vi "VFD.vi"() -> ()   [LabVIEW 2013]
uses:
  <vilib>/NI/Modbus Library/API/Master/Modbus Master.lvclass
  Variables globales/Temporales.vi
  Variables globales/Permanentes.vi
panel:
  out "Coincidentes":bool[](array[boolean])
  out "Iteración":u32
  out "Estatus (color)":u32(colorbox)
  in  "Modos":enum32{"Parámetros", "Control", "Recetas"}(tab)
  in  "Escanear":bool
  in  "Download":bool
  in  "Contenedor Fabricantes":T1(tab)
  in  "Referencias PowerFlex":T2 {"Referencia velocidad 2" items=["Potenciómetro"=1, "Teclado"=2, "Modbus"=3, "Analógica (0-10V)"=5, "Analógica (4-20mA)"=6]; "Referencia arranque 2" items=["Teclado"=1, "Terminales"=2, "Modbus"=3]; "Referencia velocidad 1" items=["Potenciómetro"=1, "Teclado"=2, "Modbus"=3, "Analógica (0-10V)"=5, "Analógica (4-20mA)"=6]; "Referencia arranque 1" items=["Teclado"=1, "Terminales"=2, "Modbus"=3]}
  in  "I/O PowerFlex":T3 {"Relevador" items=["Listo/Fallo"=0, "A frecuencia"=1, "Alimentación"=2, "Sobrefrecuencia"=6, "Sobrecorriente"=7, "Sobretensión"=8, "Modbus"=13]; "Entrada 6 (06)" items=["No asignar"=0, "Referencia vel. 2"=1, "Referencia vel. 3"=2, "Fallo auxiliar"=12, "Reset"=13, "Entrada lógica 1"=24, "Entrada lógica 2"=25]; "Entrada 5 (05)" items=["No asignar"=0, "Referencia vel. 2"=1, "Referencia vel. 3"=2, "Fallo auxiliar"=12, "Reset"=13, "Entrada lógica 1"=24, "Entrada lógica 2"=25]; "Entrada 3 (03)" items=["No asignar"=0, "Referencia vel. 2"=1, "Referencia vel. 3"=2, "Fallo auxiliar"=12, "Reset"=13, "Entrada lógica 1"=24, "Entrada lógica 2"=25, "REV 2 hilos"=50, "DIR 3 hilos"=51]; "Entrada 2 (02)" items=["No asignar"=0, "Referencia vel. 2"=1, "Referencia vel. 3"=2, "Fallo auxiliar"=12, "Reset"=13, "Entrada lógica 1"=24, "Entrada lógica 2"=25, "FWD 2 hilos"=48, "RUN 3 hilos"=49]}
  in  "Motor PowerFlex":T4={"Voltaje nominal"=0, "Frecuencia nominal"=0, "Corriente sobrecarga"=0.0, "Corriente nominal"=0.0, "Polos"=2, "Velocidad nominal"=0, "T. Aceleración"=0.0, "T. Desaleceración"=0.0, "Descargar"=FALSE} {"T. Desaleceración" format="%#_g seg"; "T. Aceleración" format="%#_g seg"; "Velocidad nominal" format="%.0f rpm"; "Voltaje nominal" format="%.0f V"; "Frecuencia nominal" format="%.0f Hz"; "Corriente sobrecarga" format="%#_g Amp"; "Corriente nominal" format="%#_g Amp"; "Polos" min=2 max=40}
  in  "Modbus PowerFlex":T5={"Velocidad datos"=0, "Identificador"=1, "Acc. pérdida comun."=0, "Tmp. pérdida comun."=1.0, "Formato RS485"=0, "Descargar"=FALSE} {"Tmp. pérdida comun." min=0.0 max=60.0 format="%#_g seg."; "Identificador" min=1 max=247; "Formato RS485" items=["RTU 8-N-1", "RTU 8-E-1", "RTU 8-O-1", "RTU 8-N-2", "RTU 8-E-2", "RTU 8-O-2"]; "Acc. pérdida comun." items=["Fallo", "Paro inercia", "Paro", "Nada"]; "Velocidad datos" items=["9600 bps", "2400 bps", "4800 bps", "9600 bps", "19200 bps", "38400 bps"]}
  in  "Referencias Schneider":T2 {"Referencia velocidad 2" items=["No asignar"=0, "Analógica (AI1)"=1, "Analógica (AI2)"=2, "Analógica (AI3)"=3, "Modbus"=164, "Potenciómetro (AIU1)"=183]; "Referencia arranque 2" items=["Terminales"=1, "Modbus"=10]; "Referencia velocidad 1" items=["No asignar"=0, "Analógica (AI1)"=1, "Analógica (AI2)"=2, "Analógica (AI3)"=3, "Modbus"=164, "Potenciómetro (AIU1)"=183]; "Referencia arranque 1" items=["Terminales"=1, "Modbus"=10]}
  in  "I/O Schneider":T6 {"Transistor" items=["Listo/Fallo"=0, "A frecuencia"=1, "Alimentación"=2, "Sobrefrecuencia"=6, "Sobrecorriente"=7, "Sobretensión"=8, "Modbus"=13]; "Relevador 2 (R2)" items=["Listo/Fallo"=0, "A frecuencia"=1, "Alimentación"=2, "Sobrefrecuencia"=6, "Sobrecorriente"=7, "Sobretensión"=8, "Modbus"=13]; "Relevador 1 (R1)" items=["Listo/Fallo"=0, "A frecuencia"=1, "Alimentación"=2, "Sobrefrecuencia"=6, "Sobrecorriente"=7, "Sobretensión"=8, "Modbus"=13]; "Entrada 6 (DI6)" items=["Listo/Fallo"=0, "A frecuencia"=1, "Alimentación"=2, "Sobrefrecuencia"=6, "Sobrecorriente"=7, "Sobretensión"=8, "Modbus"=13]; "Entrada 5 (DI5)" items=["Listo/Fallo"=0, "A frecuencia"=1, "Alimentación"=2, "Sobrefrecuencia"=6, "Sobrecorriente"=7, "Sobretensión"=8, "Modbus"=13]; "Entrada 4 (DI4)" items=["Sin asignar"=0, "Referencia vel. 2"=1, "Referencia vel. 3"=2, "Fallo auxiliar"=12, "Reset"=13, "Entrada lógica 1"=24, "Entrada lógica 2"=25]; "Entrada 3 (DI3)" items=["No asignar"=0, "Referencia vel. 2"=1, "Referencia vel. 3"=2, "Fallo auxiliar"=12, "Reset"=13, "Entrada lógica 1"=24, "Entrada lógica 2"=25]; "Entrada 2 (DI2)" items=["No asignar"=0, "Referencia vel. 2"=1, "Referencia vel. 3"=2, "Fallo auxiliar"=12, "Reset"=13, "Entrada lógica 1"=24, "Entrada lógica 2"=25, "REV 2 hilos"=50, "DIR 3 hilos"=51]; "Entrada 1 (DI1)" items=["No asignar"=0, "Referencia vel. 2"=1, "Referencia vel. 3"=2, "Fallo auxiliar"=12, "Reset"=13, "Entrada lógica 1"=24, "Entrada lógica 2"=25, "FWD 2 hilos"=48, "RUN 3 hilos"=49]}
  in  "Referencias Delta":T2 {"Referencia velocidad 2" items=["Potenciómetro"=1, "Teclado"=2, "Modbus"=3, "Analógico (0-10V)"=5, "Analógico (4-20mA)"=6]; "Referencia arranque 2" items=["Teclado"=1, "Terminales"=2, "Modbus"=3]; "Referencia velocidad 1" items=["Potenciómetro"=1, "Teclado"=2, "Modbus"=3, "Analógico (0-10V)"=5, "Analógico (4-20mA)"=6]; "Referencia arranque 1" items=["Teclado"=1, "Terminales"=2, "Modbus"=3]}
  in  "I/O Delta":T7 {"Entrada 6 (MI6)" items=["Listo/Fallo"=0, "A frecuencia"=1, "Alimentación"=2, "Sobrefrecuencia"=6, "Sobrecorriente"=7, "Sobretensión"=8, "Modbus"=13]; "Entrada 5 (MI5)" items=["Listo/Fallo"=0, "A frecuencia"=1, "Alimentación"=2, "Sobrefrecuencia"=6, "Sobrecorriente"=7, "Sobretensión"=8, "Modbus"=13]; "Entrada 4 (MI4)" items=["Sin asignar"=0, "Referencia vel. 2"=1, "Referencia vel. 3"=2, "Fallo auxiliar"=12, "Reset"=13, "Entrada lógica 1"=24, "Entrada lógica 2"=25]; "Entrada 3 (MI3)" items=["No asignar"=0, "Referencia vel. 2"=1, "Referencia vel. 3"=2, "Fallo auxiliar"=12, "Reset"=13, "Entrada lógica 1"=24, "Entrada lógica 2"=25]; "Entrada 2 (MI2)" items=["No asignar"=0, "Referencia vel. 2"=1, "Referencia vel. 3"=2, "Fallo auxiliar"=12, "Reset"=13, "Entrada lógica 1"=24, "Entrada lógica 2"=25, "REV 2 hilos"=50, "DIR 3 hilos"=51]; "Entrada 1 (MI1)" items=["No asignar"=0, "Referencia vel. 2"=1, "Referencia vel. 3"=2, "Fallo auxiliar"=12, "Reset"=13, "Entrada lógica 1"=24, "Entrada lógica 2"=25, "FWD 2 hilos"=48, "RUN 3 hilos"=49]}
  in  "Referencias ABB":T2 {"Referencia velocidad 2" items=["Potenciómetro"=1, "Teclado"=2, "Modbus"=3, "Analógico (0-10V)"=5, "Analógico (4-20mA)"=6]; "Referencia arranque 2" items=["Teclado"=1, "Terminales"=2, "Modbus"=3]; "Referencia velocidad 1" items=["Potenciómetro"=1, "Teclado"=2, "Modbus"=3, "Analógico (0-10V)"=5, "Analógico (4-20mA)"=6]; "Referencia arranque 1" items=["Teclado"=1, "Terminales"=2, "Modbus"=3]}
  in  "I/O ABB":T8 {"Entrada 4 (DI4)" items=["Sin asignar"=0, "Referencia vel. 2"=1, "Referencia vel. 3"=2, "Fallo auxiliar"=12, "Reset"=13, "Entrada lógica 1"=24, "Entrada lógica 2"=25]; "Entrada 3 (DI3)" items=["No asignar"=0, "Referencia vel. 2"=1, "Referencia vel. 3"=2, "Fallo auxiliar"=12, "Reset"=13, "Entrada lógica 1"=24, "Entrada lógica 2"=25]; "Entrada 2 (DI2)" items=["No asignar"=0, "Referencia vel. 2"=1, "Referencia vel. 3"=2, "Fallo auxiliar"=12, "Reset"=13, "Entrada lógica 1"=24, "Entrada lógica 2"=25, "REV 2 hilos"=50, "DIR 3 hilos"=51]; "Entrada 1 (DI1)" items=["No asignar"=0, "Referencia vel. 2"=1, "Referencia vel. 3"=2, "Fallo auxiliar"=12, "Reset"=13, "Entrada lógica 1"=24, "Entrada lógica 2"=25, "FWD 2 hilos"=48, "RUN 3 hilos"=49]}
  in  "Referencias LS-Electric":T2 {"Referencia velocidad 2" items=["Teclado"=0, "Analógica (V1)"=2, "Analógica (I2)"=5, "Modbus"=6]; "Referencia arranque 2" items=["Teclado"=0, "Terminales"=1, "Modbus"=3]; "Referencia velocidad 1" items=["Teclado"=0, "Analógica (V1)"=2, "Analógica (I2)"=5, "Modbus"=6]; "Referencia arranque 1" items=["Teclado"=0, "Terminales"=1, "Modbus"=3]}
  in  "I/O LS-Electric":T9 {"Relevador 2" items=["Modbus"=0, "FDT-1"=1, "FDT-2"=2, "FDT-3"=3, "FDT-4"=4, "Sobrecarga"=5, "Sobrevoltaje"=10, "Bajo voltaje"=11, "Sobrecalentamiento"=12, "RUN"=14, "STOP"=15, "Listo"=22]; "Relevador 1" items=["Modbus"=0, "FDT-1"=1, "FDT-2"=2, "FDT-3"=3, "FDT-4"=4, "Sobrecarga"=5, "Sobrevoltaje"=10, "Bajo voltaje"=11, "Sobrecalentamiento"=12, "RUN"=14, "STOP"=15, "Listo"=22]; "Entrada 5 (P5)" items=["No asignar"=0, "FWD"=1, "REV"=2, "Reset"=3, "Fallo auxiliar (BX)"=5, "Habilitar RUN"=13, "3 hilos"=14, "Segunda referencia"=15, "Segundo motor"=26]; "Entrada 4 (P4)" items=["Sin asignar"=0, "FWD"=1, "REV"=2, "Reset"=3, "Fallo auxiliar (BX)"=5, "Habilitar RUN"=13, "3 hilos"=14, "Segunda referencia"=15, "Segundo motor"=26]; "Entrada 3 (P3)" items=["No asignar"=0, "FWD"=1, "REV"=2, "Reset"=3, "Fallo auxiliar (BX)"=5, "Habilitar RUN"=13, "3 hilos"=14, "Segunda referencia"=15, "Segundo motor"=26]; "Entrada 2 (P2)" items=["No asignar"=0, "FWD"=1, "REV"=2, "Reset"=3, "Fallo auxiliar (BX)"=5, "Habilitar RUN"=13, "3 hilos"=14, "Segunda referencia"=15, "Segundo motor"=26]; "Entrada 1 (P1)" items=["No asignar"=0, "FWD"=1, "REV"=2, "Reset"=3, "Fallo auxiliar (BX)"=5, "Habilitar RUN"=13, "3 hilos"=14, "Segunda referencia"=15, "Segundo motor"=26]}
  in  "Motor LS-Electric":T10={"Frecuencia nominal"=0, "Polos"=2, "Velocidad nominal"=0, "Corriente nominal"=0.0, "Corriente sin carga"=0.0, "Voltaje nominal"=170, "Potencia nominal"=0, "Frecuencia mínima"=0.0, "Frecuencia máxima"=0.0, "T. Aceleración"=0.0, "T. Desaceleración"=0.0, "Descargar"=FALSE} {"Voltaje nominal" min=170 max=480 format="%.0f V"; "Potencia nominal" items=["0.2 kW", "0.4 kW", "0.75 kW", "1.1 kW", "1.5 kW", "2.2 kW", "3.0 kW", "3.7 kW", "4.0 kW", "5.5 kW", "7.5 kW", "11.kW"]; "T. Desaceleración" format="%#_g seg"; "T. Aceleración" format="%#_g seg"; "Frecuencia máxima" format="%#_g Hz"; "Frecuencia mínima" format="%#_g Hz"; "Polos" min=2 max=48; "Velocidad nominal" format="%.0f rpm"; "Corriente nominal" format="%#_g Amp"; "Corriente sin carga" format="%#_g Amp"; "Frecuencia nominal" items=["60 Hz", "50 Hz"]}
  in  "Modbus LS-Electric":T11={"Identificador"=1, "Velocidad datos"=0, "Formato RS485"=0, "Delay respuesta"=1, "Descargar"=FALSE} {"Delay respuesta" min=1 max=250 format="%.0f mseg."; "Formato RS485" items=["RTU 8-N-1", "RTU 8-N-2", "RTU 8-E-1", "RTU 8-O-1"]; "Velocidad datos" items=["1200 bps", "2400 bps", "4800 bps", "9600 bps", "19200 bps", "38400 bps", "56 kbps", "115 kbps"]; "Identificador" min=1 max=250}
  in  "Programa":T12 {"Programa" items=["ab1", "ab2", "ab3", "ab4"]}
  in  "Run":bool
  in  "Sentido":bool
  in  "Reset":bool
  in  "Salidas digitales":cluster{"Salida":bool, "Etiqueta":string}[](array[cluster])
  out "Entradas digitales":cluster{"Estado":bool, "Etiqueta":string}[](array[cluster])
  in  "Frecuencia":dbl format="%#_g Hz."
  in  "Recetas":T13(tab)
  in  "Recetas Allen Bradley":T14(array[cluster]) {"Modbus PowerFlex"."Tmp. pérdida comun." min=0.0 max=60.0 format="%#_g seg."; "Modbus PowerFlex"."Identificador" min=1 max=247; "Modbus PowerFlex"."Formato RS485" items=["RTU 8-N-1", "RTU 8-E-1", "RTU 8-O-1", "RTU 8-N-2", "RTU 8-E-2", "RTU 8-O-2"]; "Modbus PowerFlex"."Acc. pérdida comun." items=["Fallo", "Paro inercia", "Paro", "Nada"]; "Modbus PowerFlex"."Velocidad datos" items=["9600 bps", "2400 bps", "4800 bps", "9600 bps", "19200 bps", "38400 bps"]; "Motor PowerFlex"."T. Desaleceración" format="%#_g seg"; "Motor PowerFlex"."T. Aceleración" format="%#_g seg"; "Motor PowerFlex"."Velocidad nominal" format="%.0f rpm"; "Motor PowerFlex"."Voltaje nominal" format="%.0f V"; "Motor PowerFlex"."Frecuencia nominal" format="%.0f Hz"; "Motor PowerFlex"."Corriente sobrecarga" format="%#_g Amp"; "Motor PowerFlex"."Corriente nominal" format="%#_g Amp"; "Motor PowerFlex"."Polos" min=2 max=40; "I/O PowerFlex"."Relevador" items=["Listo/Fallo"=0, "A frecuencia"=1, "Alimentación"=2, "Sobrefrecuencia"=6, "Sobrecorriente"=7, "Sobretensión"=8, "Modbus"=13]; "I/O PowerFlex"."Entrada 6 (06)" items=["No asignar"=0, "Referencia vel. 2"=1, "Referencia vel. 3"=2, "Fallo auxiliar"=12, "Reset"=13, "Entrada lógica 1"=24, "Entrada lógica 2"=25]; "I/O PowerFlex"."Entrada 5 (05)" items=["No asignar"=0, "Referencia vel. 2"=1, "Referencia vel. 3"=2, "Fallo auxiliar"=12, "Reset"=13, "Entrada lógica 1"=24, "Entrada lógica 2"=25]; "I/O PowerFlex"."Entrada 3 (03)" items=["No asignar"=0, "Referencia vel. 2"=1, "Referencia vel. 3"=2, "Fallo auxiliar"=12, "Reset"=13, "Entrada lógica 1"=24, "Entrada lógica 2"=25, "REV 2 hilos"=50, "DIR 3 hilos"=51]; "I/O PowerFlex"."Entrada 2 (02)" items=["No asignar"=0, "Referencia vel. 2"=1, "Referencia vel. 3"=2, "Fallo auxiliar"=12, "Reset"=13, "Entrada lógica 1"=24, "Entrada lógica 2"=25, "FWD 2 hilos"=48, "RUN 3 hilos"=49]; "Referencias PowerFlex"."Referencia velocidad 2" items=["Potenciómetro"=1, "Teclado"=2, "Modbus"=3, "Analógica (0-10V)"=5, "Analógica (4-20mA)"=6]; "Referencias PowerFlex"."Referencia arranque 2" items=["Teclado"=1, "Terminales"=2, "Modbus"=3]; "Referencias PowerFlex"."Referencia velocidad 1" items=["Potenciómetro"=1, "Teclado"=2, "Modbus"=3, "Analógica (0-10V)"=5, "Analógica (4-20mA)"=6]; "Referencias PowerFlex"."Referencia arranque 1" items=["Teclado"=1, "Terminales"=2, "Modbus"=3]}
  in  "Recetas Schneider":T15(array[cluster]) {"I/O Schneider"."Transistor" items=["Listo/Fallo"=0, "A frecuencia"=1, "Alimentación"=2, "Sobrefrecuencia"=6, "Sobrecorriente"=7, "Sobretensión"=8, "Modbus"=13]; "I/O Schneider"."Relevador 2 (R2)" items=["Listo/Fallo"=0, "A frecuencia"=1, "Alimentación"=2, "Sobrefrecuencia"=6, "Sobrecorriente"=7, "Sobretensión"=8, "Modbus"=13]; "I/O Schneider"."Relevador 1 (R1)" items=["Listo/Fallo"=0, "A frecuencia"=1, "Alimentación"=2, "Sobrefrecuencia"=6, "Sobrecorriente"=7, "Sobretensión"=8, "Modbus"=13]; "I/O Schneider"."Entrada 6 (DI6)" items=["Listo/Fallo"=0, "A frecuencia"=1, "Alimentación"=2, "Sobrefrecuencia"=6, "Sobrecorriente"=7, "Sobretensión"=8, "Modbus"=13]; "I/O Schneider"."Entrada 5 (DI5)" items=["Listo/Fallo"=0, "A frecuencia"=1, "Alimentación"=2, "Sobrefrecuencia"=6, "Sobrecorriente"=7, "Sobretensión"=8, "Modbus"=13]; "I/O Schneider"."Entrada 4 (DI4)" items=["Sin asignar"=0, "Referencia vel. 2"=1, "Referencia vel. 3"=2, "Fallo auxiliar"=12, "Reset"=13, "Entrada lógica 1"=24, "Entrada lógica 2"=25]; "I/O Schneider"."Entrada 3 (DI3)" items=["No asignar"=0, "Referencia vel. 2"=1, "Referencia vel. 3"=2, "Fallo auxiliar"=12, "Reset"=13, "Entrada lógica 1"=24, "Entrada lógica 2"=25]; "I/O Schneider"."Entrada 2 (DI2)" items=["No asignar"=0, "Referencia vel. 2"=1, "Referencia vel. 3"=2, "Fallo auxiliar"=12, "Reset"=13, "Entrada lógica 1"=24, "Entrada lógica 2"=25, "REV 2 hilos"=50, "DIR 3 hilos"=51]; "I/O Schneider"."Entrada 1 (DI1)" items=["No asignar"=0, "Referencia vel. 2"=1, "Referencia vel. 3"=2, "Fallo auxiliar"=12, "Reset"=13, "Entrada lógica 1"=24, "Entrada lógica 2"=25, "FWD 2 hilos"=48, "RUN 3 hilos"=49]; "Referencias Schneider"."Referencia velocidad 2" items=["No asignar"=0, "Analógica (AI1)"=1, "Analógica (AI2)"=2, "Analógica (AI3)"=3, "Modbus"=164, "Potenciómetro (AIU1)"=183]; "Referencias Schneider"."Referencia arranque 2" items=["Terminales"=1, "Modbus"=10]; "Referencias Schneider"."Referencia velocidad 1" items=["No asignar"=0, "Analógica (AI1)"=1, "Analógica (AI2)"=2, "Analógica (AI3)"=3, "Modbus"=164, "Potenciómetro (AIU1)"=183]; "Referencias Schneider"."Referencia arranque 1" items=["Terminales"=1, "Modbus"=10]}
  in  "Recetas Delta":T16(array[cluster]) {"Referencias Delta"."Referencia velocidad 2" items=["No asignar"=0, "Analógica (AI1)"=1, "Analógica (AI2)"=2, "Analógica (AI3)"=3, "Modbus"=164, "Potenciómetro (AIU1)"=183]; "Referencias Delta"."Referencia arranque 2" items=["Terminales"=1, "Modbus"=10]; "Referencias Delta"."Referencia velocidad 1" items=["No asignar"=0, "Analógica (AI1)"=1, "Analógica (AI2)"=2, "Analógica (AI3)"=3, "Modbus"=164, "Potenciómetro (AIU1)"=183]; "Referencias Delta"."Referencia arranque 1" items=["Terminales"=1, "Modbus"=10]; "I/O Delta"."Entrada 6 (MI6)" items=["Listo/Fallo"=0, "A frecuencia"=1, "Alimentación"=2, "Sobrefrecuencia"=6, "Sobrecorriente"=7, "Sobretensión"=8, "Modbus"=13]; "I/O Delta"."Entrada 5 (MI5)" items=["Listo/Fallo"=0, "A frecuencia"=1, "Alimentación"=2, "Sobrefrecuencia"=6, "Sobrecorriente"=7, "Sobretensión"=8, "Modbus"=13]; "I/O Delta"."Entrada 4 (MI4)" items=["Sin asignar"=0, "Referencia vel. 2"=1, "Referencia vel. 3"=2, "Fallo auxiliar"=12, "Reset"=13, "Entrada lógica 1"=24, "Entrada lógica 2"=25]; "I/O Delta"."Entrada 3 (MI3)" items=["No asignar"=0, "Referencia vel. 2"=1, "Referencia vel. 3"=2, "Fallo auxiliar"=12, "Reset"=13, "Entrada lógica 1"=24, "Entrada lógica 2"=25]; "I/O Delta"."Entrada 2 (MI2)" items=["No asignar"=0, "Referencia vel. 2"=1, "Referencia vel. 3"=2, "Fallo auxiliar"=12, "Reset"=13, "Entrada lógica 1"=24, "Entrada lógica 2"=25, "REV 2 hilos"=50, "DIR 3 hilos"=51]; "I/O Delta"."Entrada 1 (MI1)" items=["No asignar"=0, "Referencia vel. 2"=1, "Referencia vel. 3"=2, "Fallo auxiliar"=12, "Reset"=13, "Entrada lógica 1"=24, "Entrada lógica 2"=25, "FWD 2 hilos"=48, "RUN 3 hilos"=49]}
  in  "Recetas ABB":T17(array[cluster]) {"Referencias ABB"."Referencia velocidad 2" items=["No asignar"=0, "Analógica (AI1)"=1, "Analógica (AI2)"=2, "Analógica (AI3)"=3, "Modbus"=164, "Potenciómetro (AIU1)"=183]; "Referencias ABB"."Referencia arranque 2" items=["Terminales"=1, "Modbus"=10]; "Referencias ABB"."Referencia velocidad 1" items=["No asignar"=0, "Analógica (AI1)"=1, "Analógica (AI2)"=2, "Analógica (AI3)"=3, "Modbus"=164, "Potenciómetro (AIU1)"=183]; "Referencias ABB"."Referencia arranque 1" items=["Terminales"=1, "Modbus"=10]; "I/O ABB"."Entrada 4 (DI4)" items=["Sin asignar"=0, "Referencia vel. 2"=1, "Referencia vel. 3"=2, "Fallo auxiliar"=12, "Reset"=13, "Entrada lógica 1"=24, "Entrada lógica 2"=25]; "I/O ABB"."Entrada 3 (DI3)" items=["No asignar"=0, "Referencia vel. 2"=1, "Referencia vel. 3"=2, "Fallo auxiliar"=12, "Reset"=13, "Entrada lógica 1"=24, "Entrada lógica 2"=25]; "I/O ABB"."Entrada 2 (DI2)" items=["No asignar"=0, "Referencia vel. 2"=1, "Referencia vel. 3"=2, "Fallo auxiliar"=12, "Reset"=13, "Entrada lógica 1"=24, "Entrada lógica 2"=25, "REV 2 hilos"=50, "DIR 3 hilos"=51]; "I/O ABB"."Entrada 1 (DI1)" items=["No asignar"=0, "Referencia vel. 2"=1, "Referencia vel. 3"=2, "Fallo auxiliar"=12, "Reset"=13, "Entrada lógica 1"=24, "Entrada lógica 2"=25, "FWD 2 hilos"=48, "RUN 3 hilos"=49]}
  in  "Recetas LS Electric":T18(array[cluster]) {"Modbus LS-Electric"."Delay respuesta" min=1 max=250 format="%.0f mseg."; "Modbus LS-Electric"."Formato RS485" items=["RTU 8-N-1", "RTU 8-N-2", "RTU 8-E-1", "RTU 8-O-1"]; "Modbus LS-Electric"."Velocidad datos" items=["1200 bps", "2400 bps", "4800 bps", "9600 bps", "19200 bps", "38400 bps", "56 kbps", "115 kbps"]; "Modbus LS-Electric"."Identificador" min=1 max=250; "Motor LS-Electric"."Voltaje nominal" min=170 max=480 format="%.0f V"; "Motor LS-Electric"."Potencia nominal" items=["0.2 kW", "0.4 kW", "0.75 kW", "1.1 kW", "1.5 kW", "2.2 kW", "3.0 kW", "3.7 kW", "4.0 kW", "5.5 kW", "7.5 kW", "11.kW"]; "Motor LS-Electric"."T. Desaceleración" format="%#_g seg"; "Motor LS-Electric"."T. Aceleración" format="%#_g seg"; "Motor LS-Electric"."Frecuencia máxima" format="%#_g Hz"; "Motor LS-Electric"."Frecuencia mínima" format="%#_g Hz"; "Motor LS-Electric"."Polos" min=2 max=48; "Motor LS-Electric"."Velocidad nominal" format="%.0f rpm"; "Motor LS-Electric"."Corriente nominal" format="%#_g Amp"; "Motor LS-Electric"."Corriente sin carga" format="%#_g Amp"; "Motor LS-Electric"."Frecuencia nominal" items=["60 Hz", "50 Hz"]; "Referencias LS-Electric"."Referencia velocidad 2" items=["No asignar"=0, "Analógica (AI1)"=1, "Analógica (AI2)"=2, "Analógica (AI3)"=3, "Modbus"=164, "Potenciómetro (AIU1)"=183]; "Referencias LS-Electric"."Referencia arranque 2" items=["Terminales"=1, "Modbus"=10]; "Referencias LS-Electric"."Referencia velocidad 1" items=["No asignar"=0, "Analógica (AI1)"=1, "Analógica (AI2)"=2, "Analógica (AI3)"=3, "Modbus"=164, "Potenciómetro (AIU1)"=183]; "Referencias LS-Electric"."Referencia arranque 1" items=["Terminales"=1, "Modbus"=10]; "I/O LS-Electric"."Relevador 2" items=["Modbus"=0, "FDT-1"=1, "FDT-2"=2, "FDT-3"=3, "FDT-4"=4, "Sobrecarga"=5, "Sobrevoltaje"=10, "Bajo voltaje"=11, "Sobrecalentamiento"=12, "RUN"=14, "STOP"=15, "Listo"=22]; "I/O LS-Electric"."Relevador 1" items=["Modbus"=0, "FDT-1"=1, "FDT-2"=2, "FDT-3"=3, "FDT-4"=4, "Sobrecarga"=5, "Sobrevoltaje"=10, "Bajo voltaje"=11, "Sobrecalentamiento"=12, "RUN"=14, "STOP"=15, "Listo"=22]; "I/O LS-Electric"."Entrada 5 (P5)" items=["No asignar"=0, "FWD"=1, "REV"=2, "Reset"=3, "Fallo auxiliar (BX)"=5, "Habilitar RUN"=13, "3 hilos"=14, "Segunda referencia"=15, "Segundo motor"=26]; "I/O LS-Electric"."Entrada 4 (P4)" items=["Sin asignar"=0, "FWD"=1, "REV"=2, "Reset"=3, "Fallo auxiliar (BX)"=5, "Habilitar RUN"=13, "3 hilos"=14, "Segunda referencia"=15, "Segundo motor"=26]; "I/O LS-Electric"."Entrada 3 (P3)" items=["No asignar"=0, "FWD"=1, "REV"=2, "Reset"=3, "Fallo auxiliar (BX)"=5, "Habilitar RUN"=13, "3 hilos"=14, "Segunda referencia"=15, "Segundo motor"=26]; "I/O LS-Electric"."Entrada 2 (P2)" items=["No asignar"=0, "FWD"=1, "REV"=2, "Reset"=3, "Fallo auxiliar (BX)"=5, "Habilitar RUN"=13, "3 hilos"=14, "Segunda referencia"=15, "Segundo motor"=26]; "I/O LS-Electric"."Entrada 1 (P1)" items=["No asignar"=0, "FWD"=1, "REV"=2, "Reset"=3, "Fallo auxiliar (BX)"=5, "Habilitar RUN"=13, "3 hilos"=14, "Segunda referencia"=15, "Segundo motor"=26]}
  out "Color Box 2":u32(colorbox)
  in  "cccc 2":u32
  out "cccc":u32
  in  "Color Box":u32(colorbox)
  out "Avance (número)":dbl format="%d%"
  out "Avance (anillo)":dbl(knob)=1.2869315802184793e-48 scale=0.0..101.0
  out "Mensaje":string
  in  "Stop":bool
  out "Salir":bool
  out "Instancia Modbus":refnum<class "Modbus Master.lvclass">
  out "Error Modbus":errorcluster
  in  "Timeout":u32
  in  "Fabricante":u32(ring)
  out "Paso":u32
  in  "Puerto COM":refnum<visa-resource-name>
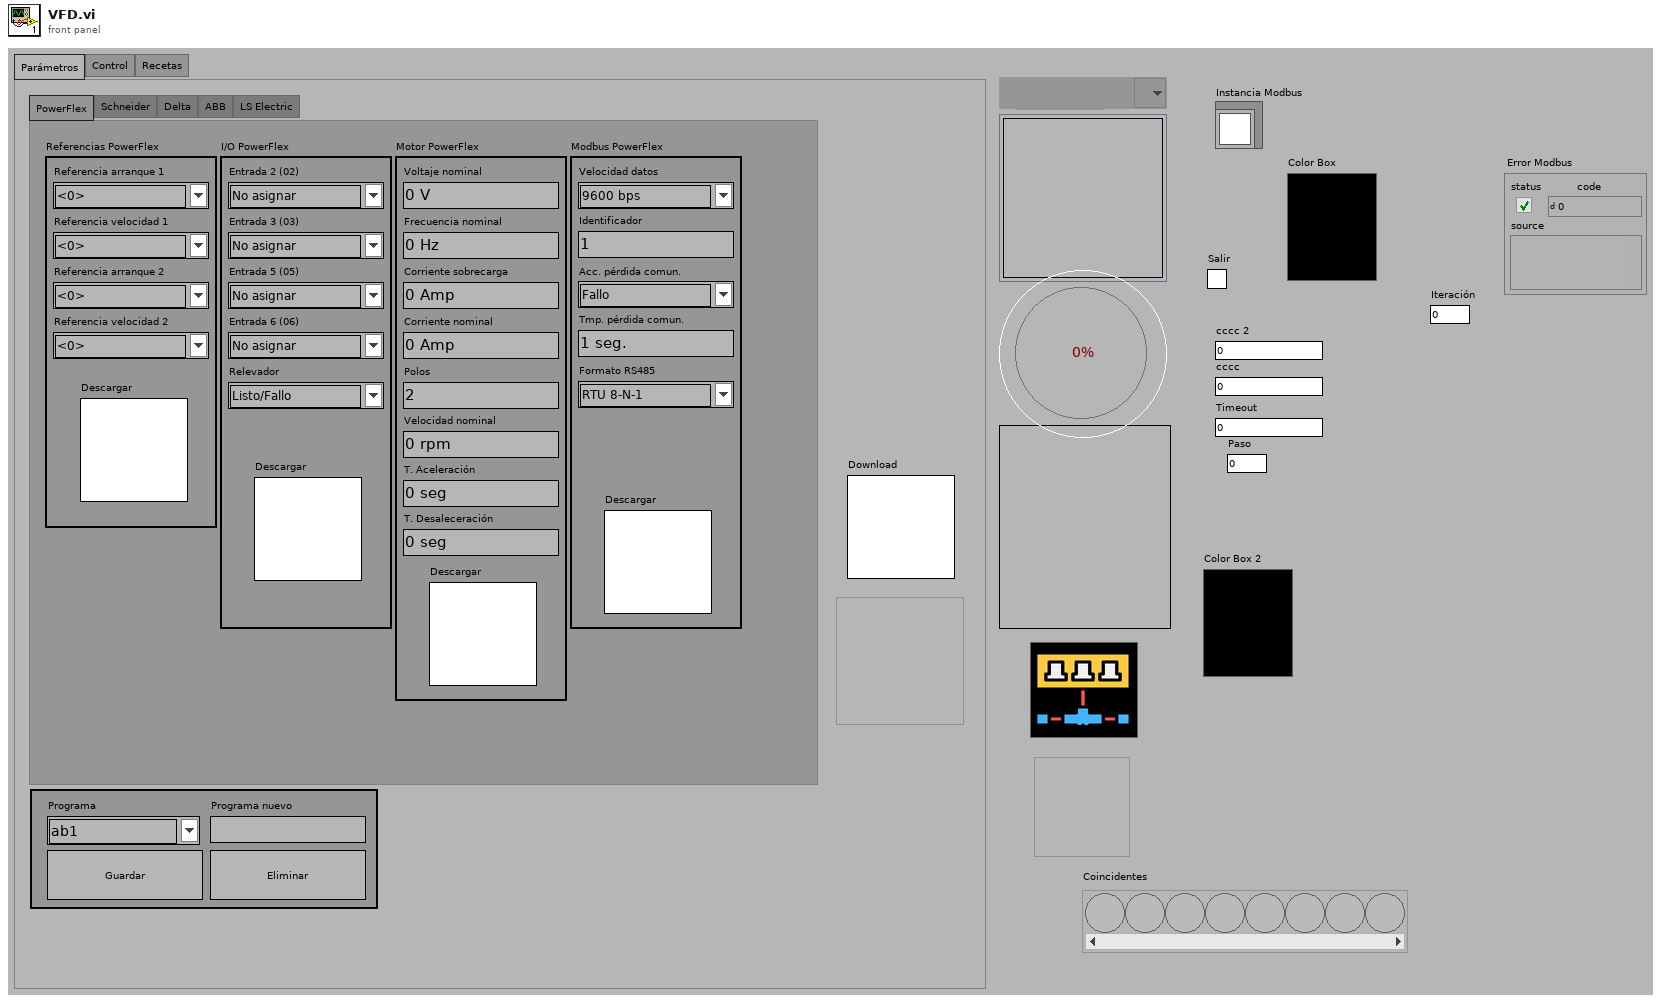
[diagram p1: front panel]
types:
  T1 = enum32{"PowerFlex", "Schneider", "Delta", "ABB", "LS Electric"}
  T2 = cluster{"Referencia arranque 1":u16, "Referencia velocidad 1":u16, "Referencia arranque 2":u16, "Referencia velocidad 2":u16, "Descargar":bool}
  T3 = cluster{"Entrada 2 (02)":u16, "Entrada 3 (03)":u16, "Entrada 5 (05)":u16, "Entrada 6 (06)":u16, "Relevador":u16, "Descargar":bool}
  T4 = cluster{"Voltaje nominal":u16, "Frecuencia nominal":u16, "Corriente sobrecarga":dbl, "Corriente nominal":dbl, "Polos":u16, "Velocidad nominal":u16, "T. Aceleración":dbl, "T. Desaleceración":dbl, "Descargar":bool}
  T5 = cluster{"Velocidad datos":u16, "Identificador":u16, "Acc. pérdida comun.":u16, "Tmp. pérdida comun.":dbl, "Formato RS485":u16, "Descargar":bool}
  T6 = cluster{"Entrada 1 (DI1)":u16, "Entrada 2 (DI2)":u16, "Entrada 3 (DI3)":u16, "Entrada 4 (DI4)":u16, "Entrada 5 (DI5)":u16, "Entrada 6 (DI6)":u16, "Relevador 1 (R1)":u16, "Relevador 2 (R2)":u16, "Transistor":u16, "Descargar":bool}
  T7 = cluster{"Entrada 1 (MI1)":u16, "Entrada 2 (MI2)":u16, "Entrada 3 (MI3)":u16, "Entrada 4 (MI4)":u16, "Entrada 5 (MI5)":u16, "Entrada 6 (MI6)":u16, "Descargar":bool}
  T8 = cluster{"Entrada 1 (DI1)":u16, "Entrada 2 (DI2)":u16, "Entrada 3 (DI3)":u16, "Entrada 4 (DI4)":u16, "Descargar":bool}
  T9 = cluster{"Entrada 1 (P1)":u16, "Entrada 2 (P2)":u16, "Entrada 3 (P3)":u16, "Entrada 4 (P4)":u16, "Entrada 5 (P5)":u16, "Relevador 1":u16, "Relevador 2":u16, "Descargar":bool}
  T10 = cluster{"Frecuencia nominal":u16, "Polos":u16, "Velocidad nominal":u16, "Corriente nominal":dbl, "Corriente sin carga":dbl, "Voltaje nominal":u16, "Potencia nominal":u16, "Frecuencia mínima":dbl, "Frecuencia máxima":dbl, "T. Aceleración":dbl, "T. Desaceleración":dbl, "Descargar":bool}
  T11 = cluster{"Identificador":u16, "Velocidad datos":u16, "Formato RS485":u16, "Delay respuesta":u16, "Descargar":bool}
  T12 = cluster{"Guardar":bool, "Eliminar":bool, "Programa":u16, "Programa nuevo":string}
  T13 = enum32{"Allen Bradley", "Schneider", "Delta", "ABB", "LS Electric"}
  T14 = cluster{"Referencias PowerFlex":cluster{"Referencia arranque 1":u16, "Referencia velocidad 1":u16, "Referencia arranque 2":u16, "Referencia velocidad 2":u16, "Descargar":bool}, "I/O PowerFlex":cluster{"Entrada 2 (02)":u16, "Entrada 3 (03)":u16, "Entrada 5 (05)":u16, "Entrada 6 (06)":u16, "Relevador":u16, "Descargar":bool}, "Motor PowerFlex":cluster{"Voltaje nominal":u16, "Frecuencia nominal":u16, "Corriente sobrecarga":dbl, "Corriente nominal":dbl, "Polos":u16, "Velocidad nominal":u16, "T. Aceleración":dbl, "T. Desaleceración":dbl, "Descargar":bool}, "Modbus PowerFlex":cluster{"Velocidad datos":u16, "Identificador":u16, "Acc. pérdida comun.":u16, "Tmp. pérdida comun.":dbl, "Formato RS485":u16, "Descargar":bool}, "Índice":u32}[]
  T15 = cluster{"Referencias Schneider":cluster{"Referencia arranque 1":u16, "Referencia velocidad 1":u16, "Referencia arranque 2":u16, "Referencia velocidad 2":u16, "Descargar":bool}, "I/O Schneider":cluster{"Entrada 1 (DI1)":u16, "Entrada 2 (DI2)":u16, "Entrada 3 (DI3)":u16, "Entrada 4 (DI4)":u16, "Entrada 5 (DI5)":u16, "Entrada 6 (DI6)":u16, "Relevador 1 (R1)":u16, "Relevador 2 (R2)":u16, "Transistor":u16, "Descargar":bool}, "Índice":u32}[]
  T16 = cluster{"Referencias Delta":cluster{"Referencia arranque 1":u16, "Referencia velocidad 1":u16, "Referencia arranque 2":u16, "Referencia velocidad 2":u16, "Descargar":bool}, "I/O Delta":cluster{"Entrada 1 (MI1)":u16, "Entrada 2 (MI2)":u16, "Entrada 3 (MI3)":u16, "Entrada 4 (MI4)":u16, "Entrada 5 (MI5)":u16, "Entrada 6 (MI6)":u16, "Descargar":bool}, "Índice":u32}[]
  T17 = cluster{"Referencias ABB":cluster{"Referencia arranque 1":u16, "Referencia velocidad 1":u16, "Referencia arranque 2":u16, "Referencia velocidad 2":u16, "Descargar":bool}, "I/O ABB":cluster{"Entrada 1 (DI1)":u16, "Entrada 2 (DI2)":u16, "Entrada 3 (DI3)":u16, "Entrada 4 (DI4)":u16, "Descargar":bool}, "Índice":u32}[]
  T18 = cluster{"Referencias LS-Electric":cluster{"Referencia arranque 1":u16, "Referencia velocidad 1":u16, "Referencia arranque 2":u16, "Referencia velocidad 2":u16, "Descargar":bool}, "I/O LS-Electric":cluster{"Entrada 1 (P1)":u16, "Entrada 2 (P2)":u16, "Entrada 3 (P3)":u16, "Entrada 4 (P4)":u16, "Entrada 5 (P5)":u16, "Relevador 1":u16, "Relevador 2":u16, "Descargar":bool}, "Motor LS-Electric":cluster{"Frecuencia nominal":u16, "Polos":u16, "Velocidad nominal":u16, "Corriente nominal":dbl, "Corriente sin carga":dbl, "Voltaje nominal":u16, "Potencia nominal":u16, "Frecuencia mínima":dbl, "Frecuencia máxima":dbl, "T. Aceleración":dbl, "T. Desaceleración":dbl, "Descargar":bool}, "Modbus LS-Electric":cluster{"Identificador":u16, "Velocidad datos":u16, "Formato RS485":u16, "Delay respuesta":u16, "Descargar":bool}, "Índice":u32}[]
  T19 = cluster{"Recetas Allen Bradley":cluster{"Referencias PowerFlex":cluster{"Referencia arranque 1":u16, "Referencia velocidad 1":u16, "Referencia arranque 2":u16, "Referencia velocidad 2":u16, "Descargar":bool}, "I/O PowerFlex":cluster{"Entrada 2 (02)":u16, "Entrada 3 (03)":u16, "Entrada 5 (05)":u16, "Entrada 6 (06)":u16, "Relevador":u16, "Descargar":bool}, "Motor PowerFlex":cluster{"Voltaje nominal":u16, "Frecuencia nominal":u16, "Corriente sobrecarga":dbl, "Corriente nominal":dbl, "Polos":u16, "Velocidad nominal":u16, "T. Aceleración":dbl, "T. Desaleceración":dbl, "Descargar":bool}, "Modbus PowerFlex":cluster{"Velocidad datos":u16, "Identificador":u16, "Acc. pérdida comun.":u16, "Tmp. pérdida comun.":dbl, "Formato RS485":u16, "Descargar":bool}, "Índice":u32}[], "Recetas Schneider":cluster{"Referencias Schneider":cluster{"Referencia arranque 1":u16, "Referencia velocidad 1":u16, "Referencia arranque 2":u16, "Referencia velocidad 2":u16, "Descargar":bool}, "I/O Schneider":cluster{"Entrada 1 (DI1)":u16, "Entrada 2 (DI2)":u16, "Entrada 3 (DI3)":u16, "Entrada 4 (DI4)":u16, "Entrada 5 (DI5)":u16, "Entrada 6 (DI6)":u16, "Relevador 1 (R1)":u16, "Relevador 2 (R2)":u16, "Transistor":u16, "Descargar":bool}, "Índice":u32}[], "Recetas Delta":cluster{"Referencias Delta":cluster{"Referencia arranque 1":u16, "Referencia velocidad 1":u16, "Referencia arranque 2":u16, "Referencia velocidad 2":u16, "Descargar":bool}, "I/O Delta":cluster{"Entrada 1 (MI1)":u16, "Entrada 2 (MI2)":u16, "Entrada 3 (MI3)":u16, "Entrada 4 (MI4)":u16, "Entrada 5 (MI5)":u16, "Entrada 6 (MI6)":u16, "Descargar":bool}, "Índice":u32}[], "Recetas ABB":cluster{"Referencias ABB":cluster{"Referencia arranque 1":u16, "Referencia velocidad 1":u16, "Referencia arranque 2":u16, "Referencia velocidad 2":u16, "Descargar":bool}, "I/O ABB":cluster{"Entrada 1 (DI1)":u16, "Entrada 2 (DI2)":u16, "Entrada 3 (DI3)":u16, "Entrada 4 (DI4)":u16, "Descargar":bool}, "Índice":u32}[], "Recetas LS Electric":cluster{"Referencias LS-Electric":cluster{"Referencia arranque 1":u16, "Referencia velocidad 1":u16, "Referencia arranque 2":u16, "Referencia velocidad 2":u16, "Descargar":bool}, "I/O LS-Electric":cluster{"Entrada 1 (P1)":u16, "Entrada 2 (P2)":u16, "Entrada 3 (P3)":u16, "Entrada 4 (P4)":u16, "Entrada 5 (P5)":u16, "Relevador 1":u16, "Relevador 2":u16, "Descargar":bool}, "Motor LS-Electric":cluster{"Frecuencia nominal":u16, "Polos":u16, "Velocidad nominal":u16, "Corriente nominal":dbl, "Corriente sin carga":dbl, "Voltaje nominal":u16, "Potencia nominal":u16, "Frecuencia mínima":dbl, "Frecuencia máxima":dbl, "T. Aceleración":dbl, "T. Desaceleración":dbl, "Descargar":bool}, "Modbus LS-Electric":cluster{"Identificador":u16, "Velocidad datos":u16, "Formato RS485":u16, "Delay respuesta":u16, "Descargar":bool}, "Índice":u32}[]}
  T20 = cluster{"Receta Allen Bradley":cluster{"Referencias PowerFlex":cluster{"Referencia arranque 1":u16, "Referencia velocidad 1":u16, "Referencia arranque 2":u16, "Referencia velocidad 2":u16, "Descargar":bool}, "I/O PowerFlex":cluster{"Entrada 2 (02)":u16, "Entrada 3 (03)":u16, "Entrada 5 (05)":u16, "Entrada 6 (06)":u16, "Relevador":u16, "Descargar":bool}, "Motor PowerFlex":cluster{"Voltaje nominal":u16, "Frecuencia nominal":u16, "Corriente sobrecarga":dbl, "Corriente nominal":dbl, "Polos":u16, "Velocidad nominal":u16, "T. Aceleración":dbl, "T. Desaleceración":dbl, "Descargar":bool}, "Modbus PowerFlex":cluster{"Velocidad datos":u16, "Identificador":u16, "Acc. pérdida comun.":u16, "Tmp. pérdida comun.":dbl, "Formato RS485":u16, "Descargar":bool}, "Índice":u32}, "Receta Schneider":cluster{"Referencias Schneider":cluster{"Referencia arranque 1":u16, "Referencia velocidad 1":u16, "Referencia arranque 2":u16, "Referencia velocidad 2":u16, "Descargar":bool}, "I/O Schneider":cluster{"Entrada 1 (DI1)":u16, "Entrada 2 (DI2)":u16, "Entrada 3 (DI3)":u16, "Entrada 4 (DI4)":u16, "Entrada 5 (DI5)":u16, "Entrada 6 (DI6)":u16, "Relevador 1 (R1)":u16, "Relevador 2 (R2)":u16, "Transistor":u16, "Descargar":bool}, "Índice":u32}, "Receta Delta":cluster{"Referencias Delta":cluster{"Referencia arranque 1":u16, "Referencia velocidad 1":u16, "Referencia arranque 2":u16, "Referencia velocidad 2":u16, "Descargar":bool}, "I/O Delta":cluster{"Entrada 1 (MI1)":u16, "Entrada 2 (MI2)":u16, "Entrada 3 (MI3)":u16, "Entrada 4 (MI4)":u16, "Entrada 5 (MI5)":u16, "Entrada 6 (MI6)":u16, "Descargar":bool}, "Índice":u32}, "Receta ABB":cluster{"Referencias ABB":cluster{"Referencia arranque 1":u16, "Referencia velocidad 1":u16, "Referencia arranque 2":u16, "Referencia velocidad 2":u16, "Descargar":bool}, "I/O ABB":cluster{"Entrada 1 (DI1)":u16, "Entrada 2 (DI2)":u16, "Entrada 3 (DI3)":u16, "Entrada 4 (DI4)":u16, "Descargar":bool}, "Índice":u32}, "Receta LS Electric":cluster{"Referencias LS-Electric":cluster{"Referencia arranque 1":u16, "Referencia velocidad 1":u16, "Referencia arranque 2":u16, "Referencia velocidad 2":u16, "Descargar":bool}, "I/O LS-Electric":cluster{"Entrada 1 (P1)":u16, "Entrada 2 (P2)":u16, "Entrada 3 (P3)":u16, "Entrada 4 (P4)":u16, "Entrada 5 (P5)":u16, "Relevador 1":u16, "Relevador 2":u16, "Descargar":bool}, "Motor LS-Electric":cluster{"Frecuencia nominal":u16, "Polos":u16, "Velocidad nominal":u16, "Corriente nominal":dbl, "Corriente sin carga":dbl, "Voltaje nominal":u16, "Potencia nominal":u16, "Frecuencia mínima":dbl, "Frecuencia máxima":dbl, "T. Aceleración":dbl, "T. Desaceleración":dbl, "Descargar":bool}, "Modbus LS-Electric":cluster{"Identificador":u16, "Velocidad datos":u16, "Formato RS485":u16, "Delay respuesta":u16, "Descargar":bool}, "Índice":u32}}
  T21 = cluster{"Referencias PowerFlex":cluster{"Referencia arranque 1":u16, "Referencia velocidad 1":u16, "Referencia arranque 2":u16, "Referencia velocidad 2":u16, "Descargar":bool}, "I/O PowerFlex":cluster{"Entrada 2 (02)":u16, "Entrada 3 (03)":u16, "Entrada 5 (05)":u16, "Entrada 6 (06)":u16, "Relevador":u16, "Descargar":bool}, "Motor PowerFlex":cluster{"Voltaje nominal":u16, "Frecuencia nominal":u16, "Corriente sobrecarga":dbl, "Corriente nominal":dbl, "Polos":u16, "Velocidad nominal":u16, "T. Aceleración":dbl, "T. Desaleceración":dbl, "Descargar":bool}, "Modbus PowerFlex":cluster{"Velocidad datos":u16, "Identificador":u16, "Acc. pérdida comun.":u16, "Tmp. pérdida comun.":dbl, "Formato RS485":u16, "Descargar":bool}, "Índice":u32}
  T22 = cluster{"Referencias Schneider":cluster{"Referencia arranque 1":u16, "Referencia velocidad 1":u16, "Referencia arranque 2":u16, "Referencia velocidad 2":u16, "Descargar":bool}, "I/O Schneider":cluster{"Entrada 1 (DI1)":u16, "Entrada 2 (DI2)":u16, "Entrada 3 (DI3)":u16, "Entrada 4 (DI4)":u16, "Entrada 5 (DI5)":u16, "Entrada 6 (DI6)":u16, "Relevador 1 (R1)":u16, "Relevador 2 (R2)":u16, "Transistor":u16, "Descargar":bool}, "Índice":u32}
  T23 = cluster{"Referencias Delta":cluster{"Referencia arranque 1":u16, "Referencia velocidad 1":u16, "Referencia arranque 2":u16, "Referencia velocidad 2":u16, "Descargar":bool}, "I/O Delta":cluster{"Entrada 1 (MI1)":u16, "Entrada 2 (MI2)":u16, "Entrada 3 (MI3)":u16, "Entrada 4 (MI4)":u16, "Entrada 5 (MI5)":u16, "Entrada 6 (MI6)":u16, "Descargar":bool}, "Índice":u32}
  T24 = cluster{"Referencias ABB":cluster{"Referencia arranque 1":u16, "Referencia velocidad 1":u16, "Referencia arranque 2":u16, "Referencia velocidad 2":u16, "Descargar":bool}, "I/O ABB":cluster{"Entrada 1 (DI1)":u16, "Entrada 2 (DI2)":u16, "Entrada 3 (DI3)":u16, "Entrada 4 (DI4)":u16, "Descargar":bool}, "Índice":u32}
  T25 = cluster{"Referencias LS-Electric":cluster{"Referencia arranque 1":u16, "Referencia velocidad 1":u16, "Referencia arranque 2":u16, "Referencia velocidad 2":u16, "Descargar":bool}, "I/O LS-Electric":cluster{"Entrada 1 (P1)":u16, "Entrada 2 (P2)":u16, "Entrada 3 (P3)":u16, "Entrada 4 (P4)":u16, "Entrada 5 (P5)":u16, "Relevador 1":u16, "Relevador 2":u16, "Descargar":bool}, "Motor LS-Electric":cluster{"Frecuencia nominal":u16, "Polos":u16, "Velocidad nominal":u16, "Corriente nominal":dbl, "Corriente sin carga":dbl, "Voltaje nominal":u16, "Potencia nominal":u16, "Frecuencia mínima":dbl, "Frecuencia máxima":dbl, "T. Aceleración":dbl, "T. Desaceleración":dbl, "Descargar":bool}, "Modbus LS-Electric":cluster{"Identificador":u16, "Velocidad datos":u16, "Formato RS485":u16, "Delay respuesta":u16, "Descargar":bool}, "Índice":u32}
  T26 = enum16{"open", "replace", "create", "open or create", "replace or create", "replace or create with confirmation"}
  T27 = typedef "LVStringsAndValuesArrayTypeDef.ctl" = cluster{"String":string, "Value":ext}[]
  T28 = cluster{"Recetas Allen Bradley":cluster{"Referencias PowerFlex":cluster{"Referencia arranque 1":u16, "Referencia velocidad 1":u16, "Referencia arranque 2":u16, "Referencia velocidad 2":u16, "Descargar":bool}, "I/O PowerFlex":cluster{"Entrada 2 (02)":u16, "Entrada 3 (03)":u16, "Entrada 5 (05)":u16, "Entrada 6 (06)":u16, "Relevador":u16, "Descargar":bool}, "Motor PowerFlex":cluster{"Voltaje nominal":u16, "Frecuencia nominal":u16, "Corriente sobrecarga":dbl, "Corriente nominal":dbl, "Polos":u16, "Velocidad nominal":u16, "T. Aceleración":dbl, "T. Desaleceración":dbl, "Descargar":bool}, "Modbus PowerFlex":cluster{"Velocidad datos":u16, "Identificador":u16, "Acc. pérdida comun.":u16, "Tmp. pérdida comun.":dbl, "Formato RS485":u16, "Descargar":bool}, "Índice":u32}[], "Recetas Schneider":cluster{"Referencias Schneider":cluster{"Referencia arranque 1":u16, "Referencia velocidad 1":u16, "Referencia arranque 2":u16, "Referencia velocidad 2":u16, "Descargar":bool}, "I/O Schneider":cluster{"Entrada 1 (DI1)":u16, "Entrada 2 (DI2)":u16, "Entrada 3 (DI3)":u16, "Entrada 4 (DI4)":u16, "Entrada 5 (DI5)":u16, "Entrada 6 (DI6)":u16, "Relevador 1 (R1)":u16, "Relevador 2 (R2)":u16, "Transistor":u16, "Descargar":bool}, "Índice":u32}[], "Recetas Delta":cluster{"Referencias Delta":cluster{"Referencia arranque 1":u16, "Referencia velocidad 1":u16, "Referencia arranque 2":u16, "Referencia velocidad 2":u16, "Descargar":bool}, "I/O Delta":cluster{"Entrada 1 (MI1)":u16, "Entrada 2 (MI2)":u16, "Entrada 3 (MI3)":u16, "Entrada 4 (MI4)":u16, "Entrada 5 (MI5)":u16, "Entrada 6 (MI6)":u16, "Descargar":bool}, "Índice":u32}[], "Recetas ABB":cluster{"Referencias ABB":cluster{"Referencia arranque 1":u16, "Referencia velocidad 1":u16, "Referencia arranque 2":u16, "Referencia velocidad 2":u16, "Descargar":bool}, "I/O ABB":cluster{"Entrada 1 (DI1)":u16, "Entrada 2 (DI2)":u16, "Entrada 3 (DI3)":u16, "Entrada 4 (DI4)":u16, "Descargar":bool}, "Índice":u32}[], "Recetas LS Electric":cluster{"Referencias LS-Electric":cluster{"Referencia arranque 1":u16, "Referencia velocidad 1":u16, "Referencia arranque 2":u16, "Referencia velocidad 2":u16, "Descargar":bool}, "I/O LS-Electric":cluster{"Entrada 1 (P1)":u16, "Entrada 2 (P2)":u16, "Entrada 3 (P3)":u16, "Entrada 4 (P4)":u16, "Entrada 5 (P5)":u16, "Relevador 1":u16, "Relevador 2":u16, "Descargar":bool}, "Motor LS-Electric 2":cluster{"Frecuencia nominal":u16, "Polos":u16, "Velocidad nominal":u16, "Corriente nominal":dbl, "Corriente sin carga":dbl, "Voltaje nominal":u16, "Potencia nominal":u16, "Frecuencia mínima":dbl, "Frecuencia máxima":dbl, "T. Aceleración":dbl, "T. Desaceleración":dbl, "Descargar":bool}, "Modbus LS-Electric":cluster{"Identificador":u16, "Velocidad datos":u16, "Formato RS485":u16, "Delay respuesta":u16, "Descargar":bool}, "Índice":u32}[]}
  T29 = cluster{"Referencias LS-Electric":cluster{"Referencia arranque 1":u16, "Referencia velocidad 1":u16, "Referencia arranque 2":u16, "Referencia velocidad 2":u16, "Descargar":bool}, "I/O LS-Electric":cluster{"Entrada 1 (P1)":u16, "Entrada 2 (P2)":u16, "Entrada 3 (P3)":u16, "Entrada 4 (P4)":u16, "Entrada 5 (P5)":u16, "Relevador 1":u16, "Relevador 2":u16, "Descargar":bool}, "Motor LS-Electric 2":cluster{"Frecuencia nominal":u16, "Polos":u16, "Velocidad nominal":u16, "Corriente nominal":dbl, "Corriente sin carga":dbl, "Voltaje nominal":u16, "Potencia nominal":u16, "Frecuencia mínima":dbl, "Frecuencia máxima":dbl, "T. Aceleración":dbl, "T. Desaceleración":dbl, "Descargar":bool}, "Modbus LS-Electric":cluster{"Identificador":u16, "Velocidad datos":u16, "Formato RS485":u16, "Delay respuesta":u16, "Descargar":bool}, "Índice":u32}[]
  T30 = cluster{"Referencias PowerFlex":cluster{"Referencia arranque 1":u16, "Referencia velocidad 1":u16, "Referencia arranque 2":u16, "Referencia velocidad 2":u16, "Descargar":bool}, "Referencias Schneider":cluster{"Referencia arranque 1":u16, "Referencia velocidad 1":u16, "Referencia arranque 2":u16, "Referencia velocidad 2":u16, "Descargar":bool}, "Referencias Delta":cluster{"Referencia arranque 1":u16, "Referencia velocidad 1":u16, "Referencia arranque 2":u16, "Referencia velocidad 2":u16, "Descargar":bool}, "Referencias ABB":cluster{"Referencia arranque 1":u16, "Referencia velocidad 1":u16, "Referencia arranque 2":u16, "Referencia velocidad 2":u16, "Descargar":bool}, "Referencias LS-Electric":cluster{"Referencia arranque 1":u16, "Referencia velocidad 1":u16, "Referencia arranque 2":u16, "Referencia velocidad 2":u16, "Descargar":bool}}
  T31 = cluster{"I/O PowerFlex":cluster{"Entrada 2 (02)":u16, "Entrada 3 (03)":u16, "Entrada 5 (05)":u16, "Entrada 6 (06)":u16, "Relevador":u16, "Descargar":bool}, "I/O Schneider":cluster{"Entrada 1 (DI1)":u16, "Entrada 2 (DI2)":u16, "Entrada 3 (DI3)":u16, "Entrada 4 (DI4)":u16, "Entrada 5 (DI5)":u16, "Entrada 6 (DI6)":u16, "Relevador 1 (R1)":u16, "Relevador 2 (R2)":u16, "Transistor":u16, "Descargar":bool}, "I/O Delta":cluster{"Entrada 1 (MI1)":u16, "Entrada 2 (MI2)":u16, "Entrada 3 (MI3)":u16, "Entrada 4 (MI4)":u16, "Entrada 5 (MI5)":u16, "Entrada 6 (MI6)":u16, "Descargar":bool}, "I/O ABB":cluster{"Entrada 1 (DI1)":u16, "Entrada 2 (DI2)":u16, "Entrada 3 (DI3)":u16, "Entrada 4 (DI4)":u16, "Descargar":bool}, "I/O LS-Electric":cluster{"Entrada 1 (P1)":u16, "Entrada 2 (P2)":u16, "Entrada 3 (P3)":u16, "Entrada 4 (P4)":u16, "Entrada 5 (P5)":u16, "Relevador 1":u16, "Relevador 2":u16, "Descargar":bool}}
  T32 = cluster{"Motor PowerFlex":cluster{"Voltaje nominal":u16, "Frecuencia nominal":u16, "Corriente sobrecarga":dbl, "Corriente nominal":dbl, "Polos":u16, "Velocidad nominal":u16, "T. Aceleración":dbl, "T. Desaleceración":dbl, "Descargar":bool}, "Motor LS-Electric":cluster{"Frecuencia nominal":u16, "Polos":u16, "Velocidad nominal":u16, "Corriente nominal":dbl, "Corriente sin carga":dbl, "Voltaje nominal":u16, "Potencia nominal":u16, "Frecuencia mínima":dbl, "Frecuencia máxima":dbl, "T. Aceleración":dbl, "T. Desaceleración":dbl, "Descargar":bool}}
  T33 = cluster{"Modbus PowerFlex":cluster{"Velocidad datos":u16, "Identificador":u16, "Acc. pérdida comun.":u16, "Tmp. pérdida comun.":dbl, "Formato RS485":u16, "Descargar":bool}, "Modbus LS-Electric":cluster{"Identificador":u16, "Velocidad datos":u16, "Formato RS485":u16, "Delay respuesta":u16, "Descargar":bool}}
  T34 = enum8{"Enabled", "Disabled", "Disabled and Grayed Out"}
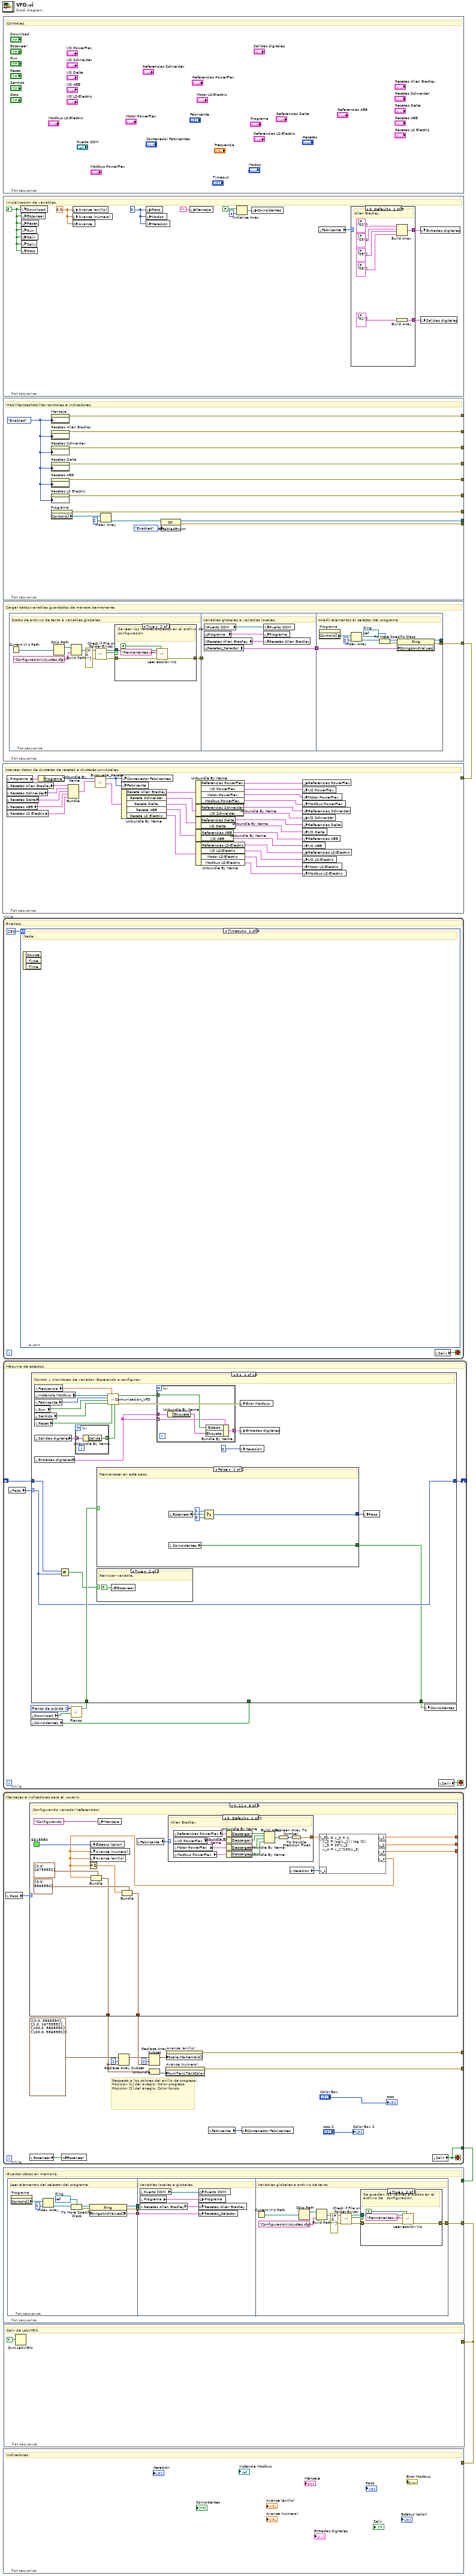
[diagram p0: block diagram]
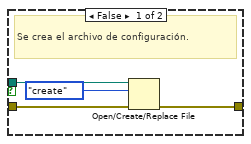
[diagram p2: hidden frame]
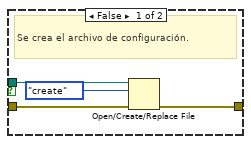
[diagram p3: hidden frame]
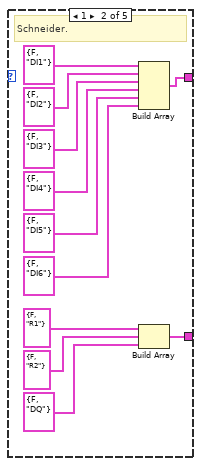
[diagram p4: hidden frame]
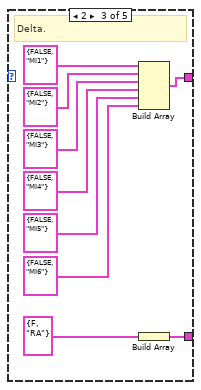
[diagram p5: hidden frame]
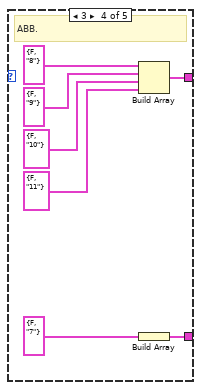
[diagram p6: hidden frame]
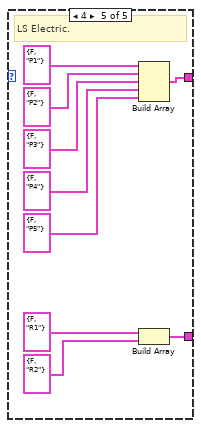
[diagram p7: hidden frame]
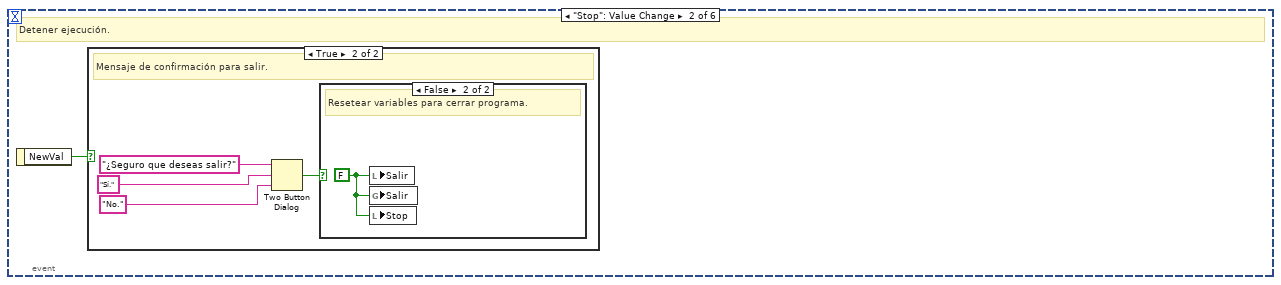
[diagram p8: hidden frame]
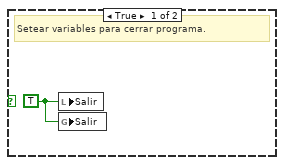
[diagram p10: hidden frame]
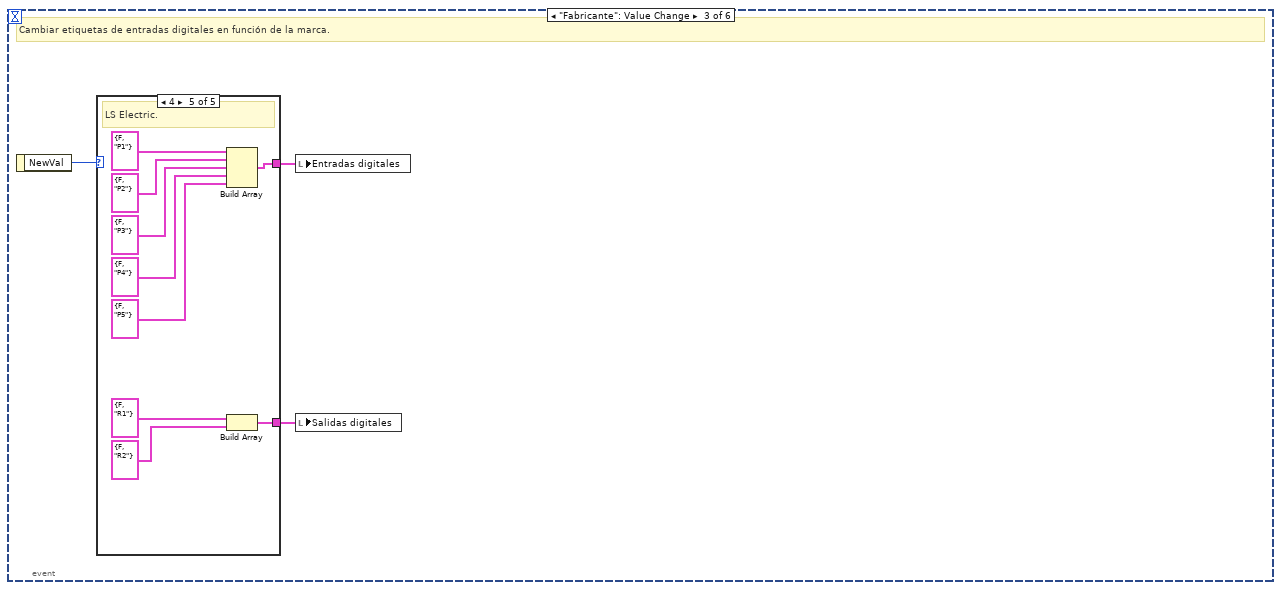
[diagram p11: hidden frame]
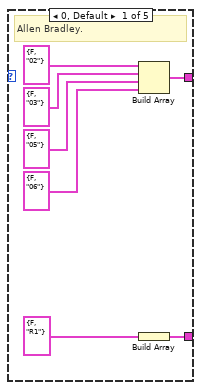
[diagram p12: hidden frame]
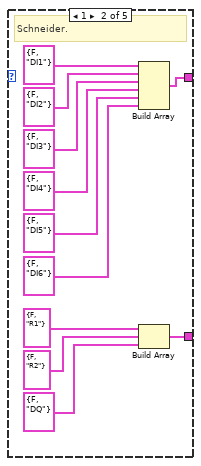
[diagram p13: hidden frame]
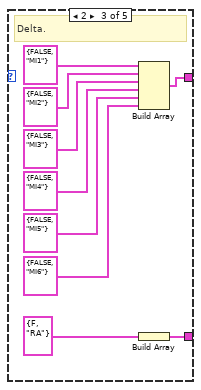
[diagram p14: hidden frame]
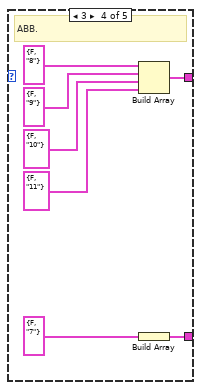
[diagram p15: hidden frame]
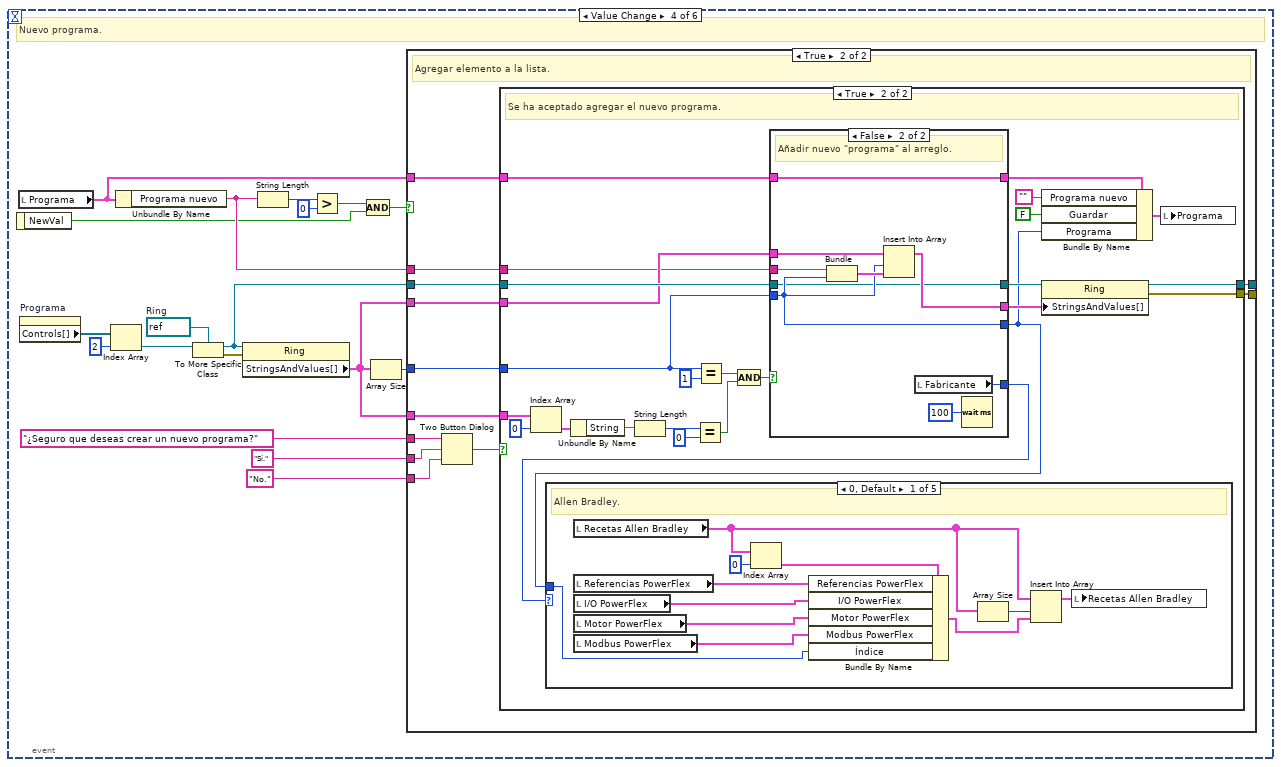
[diagram p16: hidden frame]
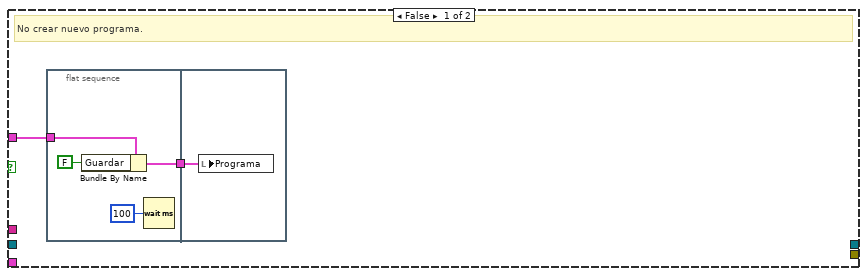
[diagram p17: hidden frame]
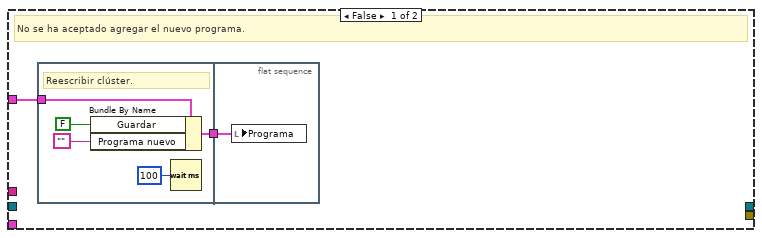
[diagram p18: hidden frame]
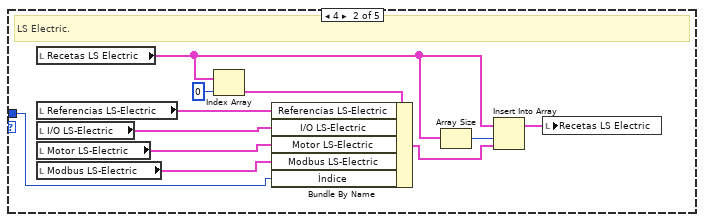
[diagram p19: hidden frame]
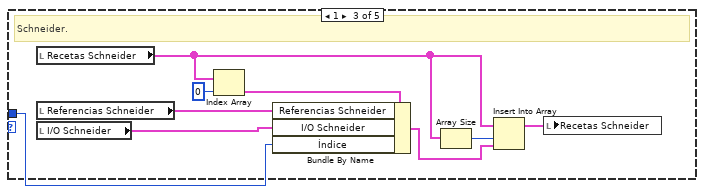
[diagram p20: hidden frame]
diagram:
  n1 = flat-sequence {
    tunnel: w2 -> [_]
    frame #0 {
      # "Acarrear datos de clústeres de recetas a clústeres principales."
      n2 = local read "Programa"() -> (w32:T12)
      n3 = local read "Recetas Allen Bradley"() -> (w30:T14)
      n4 = local read "Recetas Schneider"() -> (w29:T15)
      n5 = local read "Recetas Delta"() -> (w28:T16)
      n6 = local read "Recetas ABB"() -> (w27:T17)
      n7 = local read "Recetas LS Electric"() -> (w26:T18)
      n8 = Unbundle By Name(w32) -> ("Programa"=w31:u16)
      n9 = Bundle("Recetas Allen Bradley"=w30, "Recetas Schneider"=w29, "Recetas Delta"=w28, "Recetas ABB"=w27, "Recetas LS Electric"=w26) -> (w25:T19)  [unwired: 1 in]
      n10 = call "Búsqueda_Receta.vi"("Receta"=w25, "Índice"=w31) -> ("Recetas Out"=w23:T20, "Fabricante"=w24:u32)  [unwired: 8 in]
      n11 = local write "Contenedor Fabricantes"(w24) -> ()
      n12 = local write "Fabricante"(w24) -> ()
      n13 = Unbundle By Name(w23) -> ("Receta Allen Bradley"=w22:T21, "Receta Schneider"=w21:T22, "Receta Delta"=w20:T23, "Receta ABB"=w19:T24, "Receta LS Electric"=w18:T25)
      n14 = Unbundle By Name(w22) -> ("Referencias PowerFlex"=w17:T2, "I/O PowerFlex"=w16:T3, "Motor PowerFlex"=w15:T4, "Modbus PowerFlex"=w14:T5)
      n15 = Unbundle By Name(w21) -> ("Referencias Schneider"=w13:T2, "I/O Schneider"=w12:T6)
      n16 = Unbundle By Name(w20) -> ("Referencias Delta"=w11:T2, "I/O Delta"=w10:T7)
      n17 = Unbundle By Name(w19) -> ("Referencias ABB"=w9:T2, "I/O ABB"=w8:T8)
      n18 = Unbundle By Name(w18) -> ("Referencias LS-Electric"=w7:T2, "I/O LS-Electric"=w6:T9, "Motor LS-Electric"=w5:T10, "Modbus LS-Electric"=w4:T11)
      n19 = local write "Referencias PowerFlex"(w17) -> ()
      n20 = local write "I/O PowerFlex"(w16) -> ()
      n21 = local write "Motor PowerFlex"(w15) -> ()
      n22 = local write "Modbus PowerFlex"(w14) -> ()
      n23 = local write "Referencias Schneider"(w13) -> ()
      n24 = local write "I/O Schneider"(w12) -> ()
      n25 = local write "Referencias Delta"(w11) -> ()
      n26 = local write "I/O Delta"(w10) -> ()
      n27 = local write "Referencias ABB"(w9) -> ()
      n28 = local write "I/O ABB"(w8) -> ()
      n29 = local write "Referencias LS-Electric"(w7) -> ()
      n30 = local write "I/O LS-Electric"(w6) -> ()
      n31 = local write "Motor LS-Electric"(w5) -> ()
      n32 = local write "Modbus LS-Electric"(w4) -> ()
    }
  }
  n33 = flat-sequence {
    tunnel: [w33] -> w2
    frame #0 {
      # "Cargar datos/variables guardadas de manera permanente."
      n34 = flat-sequence {
        tunnel: [w36] -> w35
        tunnel: w35 -> [_]
        tunnel: [w54] -> w34
        tunnel: w34 -> [w60]
        tunnel: [w59] -> _
        tunnel: [w58] -> w33
        frame #0 {
          # "Datos de archivo de texto a variables globales."
          n35 = Current VI's Path() -> (path=w38:path)
          n36 = Strip Path(path=w38) -> (stripped path=w37:path)  [unwired: 1 out]
          n37 = Build Path(base path=w37, name or relative path="Configuración\\Ajustes.cfg") -> (appended path=w43:path)
          n38 = call <vilib>:"Check if File or Folder Exists.vi"("error in (no error)"=errorcluster {"status"=FALSE, "code"=0, "source"=""}, "path"=w43) -> ("error out"=w40:errorcluster, "file or folder exists?"=w39:bool, "dup path"=w41:path)  [unwired: 7 in]
          n39 = case shown="True" w39 {
            tunnel: w41 -> [w47 w51]
            tunnel: w40 -> [w46 w52]
            tunnel: [w45 w49] -> w36
            frame False {
              # "Se crea el archivo de configuración."
              n40 = Open/Create/Replace File(file path (use dialog)=w47, error in=w46, operation (0:open)=T26."create") -> (error out=w45:errorcluster)  [unwired: 3 in, 2 out]
            }
            frame True {
              # "Se leen los valores alojados en el archivo de   configuración."
              n41 = call "Leer escribir VIs.vi"("Write? (Read)"=FALSE, "error in"=w52, "VIs to save-Restore"="Permanentes.vi", "Program File Path"=w51) -> ("error out"=w49:errorcluster)  [unwired: 7 in]
            }
          }
        }
        frame #1 {
          # "Variables globales a variables locales."
          n42 = global read "Permanentes.vi" "Puerto COM"() -> (w57:refnum<visa-resource-name>)
          n43 = global read "Permanentes.vi" "Programa"() -> (w55:T12)
          n44 = global read "Permanentes.vi" "Recetas Allen Bradley"() -> (w56:T14)
          n45 = global read "Permanentes.vi" "Recetas_Selector"() -> (w54:cluster{"String":string, "Value":ext}[])
          n46 = local write "Puerto COM"(w57) -> ()
          n47 = local write "Programa"(w55) -> ()
          n48 = local write "Recetas Allen Bradley"(w56) -> ()
        }
        frame #2 {
          w66 = refnum<vi> refnum  # Ring
          # "Añadir elementos al selector del programa."
          n49 = property on="Programa" class="Clust (strict)"() -> ("Controls[]"=w64:refnum<vi>[])  [unwired: 2 in, 2 out]
          n50 = Index Array(array=w64, index=2) -> (element=w65:refnum<vi>)
          n51 = To More Specific Class(target class=w66, reference=w65) -> (specific class reference=w62:refnum<vi>, error out=w61:errorcluster)  [unwired: 1 in]
          n52 = property class="Ring"(reference=w62, error in=w61, "StringsAndValues[]"=w60) -> (reference out=w59:refnum<vi>, error out=w58:errorcluster)
        }
      }
    }
  }
  n53 = while {
    stop <- w68 stop-if-true
    # "Eventos."
    n54 = event shown="[0] Timeout" {
      selector: _ -> [_ _ _ _ _ _]
      dyn-events: _ -> [_ _ _ _ _ _]
      timeout: 250 -> [_ _ _ _ _ _]
      event Timeout {
        # "Nada."
        n55 = event-data() -> ()  [unwired: 1 in, 3 out]
      }
      event "Stop": Value Change {
        # "Detener ejecución."
        n56 = event-data() -> ("NewVal"=w69:bool)  [unwired: 1 in]
        n57 = case shown="True" w69 {
          frame False {
            # "Nada."
          }
          frame True {
            # "Mensaje de confirmación para salir."
            n58 = Two Button Dialog(message="¿Seguro que deseas salir?", 1:"No." ("F button name (\"Cancel\")"), 2:"Sí." ("T button name (\"OK\")")) -> (T button?=w70:bool)
            n59 = case shown="False" w70 {
              frame True {
                w74 = TRUE
                # "Setear variables para cerrar programa."
                n60 = local write "Salir"(w74) -> ()
                n61 = global write "Temporales.vi" "Salir"(w74) -> ()
              }
              frame False {
                w75 = FALSE
                # "Resetear variables para cerrar programa."
                n62 = local write "Salir"(w75) -> ()
                n63 = global write "Temporales.vi" "Salir"(w75) -> ()
                n64 = local write "Stop"(w75) -> ()
              }
            }
          }
        }
      }
      event "Fabricante": Value Change {
        # "Cambiar etiquetas de entradas digitales en función de la marca."
        n65 = event-data() -> ("NewVal"=w76:u32)  [unwired: 1 in]
        n66 = case shown="4" w76 {
          tunnel: [w81 w92 w101 w108 w117] -> w78
          tunnel: [w79 w89 w98 w107 w115] -> w77
          frame 0, Default {
            # "Allen Bradley."
            n67 = Build Array(cluster{bool, string} {FALSE, "02"}, cluster{bool, string} {FALSE, "03"}, cluster{bool, string} {FALSE, "05"}, cluster{bool, string} {FALSE, "06"}) -> (w81:cluster{bool, string}[])
            n68 = Build Array(cluster{bool, string} {FALSE, "R1"}) -> (w79:cluster{bool, string}[])
          }
          frame 1 {
            # "Schneider."
            n69 = Build Array(cluster{bool, string} {FALSE, "DI1"}, cluster{bool, string} {FALSE, "DI2"}, cluster{bool, string} {FALSE, "DI3"}, cluster{bool, string} {FALSE, "DI4"}, cluster{bool, string} {FALSE, "DI5"}, cluster{bool, string} {FALSE, "DI6"}) -> (w92:cluster{bool, string}[])
            n70 = Build Array(cluster{bool, string} {FALSE, "R1"}, cluster{bool, string} {FALSE, "R2"}, cluster{bool, string} {FALSE, "DQ"}) -> (w89:cluster{bool, string}[])
          }
          frame 2 {
            # "Delta."
            n71 = Build Array(cluster{bool, string} {FALSE, "MI1"}, cluster{bool, string} {FALSE, "MI2"}, cluster{bool, string} {FALSE, "MI3"}, cluster{bool, string} {FALSE, "MI4"}, cluster{bool, string} {FALSE, "MI5"}, cluster{bool, string} {FALSE, "MI6"}) -> (w101:cluster{bool, string}[])
            n72 = Build Array(cluster{bool, string} {FALSE, "RA"}) -> (w98:cluster{bool, string}[])
          }
          frame 3 {
            # "ABB."
            n73 = Build Array(cluster{bool, string} {FALSE, "8"}, cluster{bool, string} {FALSE, "9"}, cluster{bool, string} {FALSE, "10"}, cluster{bool, string} {FALSE, "11"}) -> (w108:cluster{bool, string}[])
            n74 = Build Array(cluster{bool, string} {FALSE, "7"}) -> (w107:cluster{bool, string}[])
          }
          frame 4 {
            # "LS Electric."
            n75 = Build Array(cluster{bool, string} {FALSE, "P1"}, cluster{bool, string} {FALSE, "P2"}, cluster{bool, string} {FALSE, "P3"}, cluster{bool, string} {FALSE, "P4"}, cluster{bool, string} {FALSE, "P5"}) -> (w117:cluster{bool, string}[])
            n76 = Build Array(cluster{bool, string} {FALSE, "R1"}, cluster{bool, string} {FALSE, "R2"}) -> (w115:cluster{bool, string}[])
          }
        }
        n77 = local write "Entradas digitales"(w78) -> ()
        n78 = local write "Salidas digitales"(w77) -> ()
      }
      event "Programa.Guardar": Value Change {
        w135 = refnum<vi> refnum  # Ring
        # "Nuevo programa."
        n79 = event-data() -> ("NewVal"=w125:bool)  [unwired: 1 in]
        n80 = local read "Programa"() -> (w127:T12)
        n81 = property on="Programa" class="Clust (strict)"() -> ("Controls[]"=w133:refnum<vi>[])  [unwired: 2 in, 2 out]
        n82 = Index Array(array=w133, index=2) -> (element=w134:refnum<vi>)
        n83 = Unbundle By Name(w127) -> ("Programa nuevo"=w128:string)
        n84 = To More Specific Class(target class=w135, reference=w134) -> (specific class reference=w129:refnum<vi>, error out=w136:errorcluster)  [unwired: 1 in]
        n85 = property class="Ring"(reference=w129, error in=w136) -> ("StringsAndValues[]"=w130:T27)  [unwired: 2 out]
        n86 = String Length(string=w128) -> (length=w139:i32)
        n87 = Greater?(x=w139, y=0) -> (0:w126:bool)
        n88 = Compound Arithmetic op=AND(w126, w125) -> (w137:bool)
        n89 = Array Size(array=w130) -> (size(s)=w131:i32)
        n90 = case shown="True" w137 {
          tunnel: w131 -> [_ w158]
          tunnel: w130 -> [_ w157]
          tunnel: w130 -> [_ w155]
          tunnel: w129 -> [_ w156]
          tunnel: w128 -> [_ w154]
          tunnel: w127 -> [w141 w153]
          tunnel: "¿Seguro que deseas crear un nuevo programa?" ("message") -> [_ w152]
          tunnel: "Sí." ("T button name (\"OK\")") -> [_ w151]
          tunnel: "No." ("F button name (\"Cancel\")") -> [_ w150]
          tunnel: [_ w149] -> _
          tunnel: [_ w148] -> _
          frame False {
            # "No crear nuevo programa."
            n91 = flat-sequence {
              tunnel: w141 -> [w144]
              tunnel: [w142] -> w140
              tunnel: w140 -> [w146]
              frame #0 {
                n92 = Bundle By Name(cluster=w144, "Guardar"=FALSE) -> (w142:T12)
                n93 = Wait (ms)(milliseconds to wait=u32 100) -> ()  [unwired: 1 out]
              }
              frame #1 {
                n94 = local write "Programa"(w146) -> ()
              }
            }
          }
          frame True {
            # "Agregar elemento a la lista."
            n95 = Two Button Dialog(message=w152, 1:w150, 2:w151) -> (T button?=w147:bool)
            n96 = case shown="True" w147 {
              tunnel: w158 -> [_ w191]
              tunnel: w157 -> [_ w189]
              tunnel: w156 -> [_ w180]
              tunnel: w155 -> [_ w179]
              tunnel: w154 -> [_ w178]
              tunnel: w153 -> [w159 w174]
              tunnel: [_ w170] -> w149
              tunnel: [_ w169] -> w148
              frame False {
                # "No se ha aceptado agregar el nuevo programa."
                n97 = flat-sequence {
                  tunnel: w159 -> [w164]
                  tunnel: [w162] -> w160
                  tunnel: w160 -> [w166]
                  frame #0 {
                    # "Reescribir clúster."
                    n98 = Bundle By Name(cluster=w164, "Guardar"=FALSE, "Programa nuevo"="") -> (w162:T12)
                    n99 = Wait (ms)(milliseconds to wait=u32 100) -> ()  [unwired: 1 out]
                  }
                  frame #1 {
                    n100 = local write "Programa"(w166) -> ()
                  }
                }
              }
              frame True {
                # "Se ha aceptado agregar el nuevo programa."
                n101 = Index Array(array=w189, index=0) -> (element=w187:cluster{"String":string, "Value":ext})
                n102 = Unbundle By Name(w187) -> ("String"=w186:string)
                n103 = String Length(string=w186) -> (length=w185:i32)
                n104 = Equal?(x=w185, y=0) -> (x = y?=w182:bool)
                n105 = Equal?(x=w191, y=1) -> (x = y?=w183:bool)
                n106 = Compound Arithmetic op=AND(w183, w182) -> (w181:bool)
                n107 = case shown="False" w181 {
                  tunnel: w178 -> [w250 w259]
                  tunnel: w191 -> [w247 w256]
                  tunnel: w180 -> [w242 w252]
                  tunnel: w179 -> [_ w258]
                  tunnel: [w244 w256] -> w167
                  tunnel: w174 -> [w246 w255]
                  tunnel: [w246 w255] -> w173
                  tunnel: [w243 w253] -> w171
                  tunnel: [w242 w252] -> w172
                  tunnel: [w241 w251] -> w168
                  frame True {
                    # "Reemplazar primer elemento de arreglo."
                    n108 = Bundle("Programa nuevo"=w250, 0) -> (w248:cluster{"Programa nuevo":string, i32})  [unwired: 1 in]
                    n109 = Decrement(x=w247) -> (x-1=w244:i32)
                    n110 = Build Array(w248) -> (w243:cluster{"Programa nuevo":string, i32}[])
                    n111 = local read "Fabricante"() -> (w241:u32)
                    n112 = Wait (ms)(milliseconds to wait=u32 100) -> ()  [unwired: 1 out]
                  }
                  frame False {
                    # "Añadir nuevo \"programa\" al arreglo."
                    n113 = Bundle("Programa nuevo"=w259, w256) -> (w257:cluster{"Programa nuevo":string, i32})  [unwired: 1 in]
                    n114 = Insert Into Array(array=w258, index=w256, new element=w257) -> (w253:T27)
                    n115 = local read "Fabricante"() -> (w251:u32)
                    n116 = Wait (ms)(milliseconds to wait=u32 100) -> ()  [unwired: 1 out]
                  }
                }
                n117 = case shown="0, Default" w168 {
                  tunnel: w167 -> [w193 w205 w214 w223 w232]
                  frame 0, Default {
                    # "Allen Bradley."
                    n118 = local read "Recetas Allen Bradley"() -> (w196:T14)
                    n119 = local read "Referencias PowerFlex"() -> (w202:T2)
                    n120 = local read "I/O PowerFlex"() -> (w201:T3)
                    n121 = local read "Motor PowerFlex"() -> (w200:T4)
                    n122 = local read "Modbus PowerFlex"() -> (w199:T5)
                    n123 = Index Array(array=w196, index=0) -> (element=w197:T21)
                    n124 = Bundle By Name(cluster=w197, "Referencias PowerFlex"=w202, "I/O PowerFlex"=w201, "Motor PowerFlex"=w200, "Modbus PowerFlex"=w199, "Índice"=w193) -> (w192:T21)
                    n125 = Array Size(array=w196) -> (size(s)=w195:i32)
                    n126 = Insert Into Array(array=w196, index=w195, new element=w192) -> (w194:T14)
                    n127 = local write "Recetas Allen Bradley"(w194) -> ()
                  }
                  frame 4 {
                    # "LS Electric."
                    n128 = local read "Recetas LS Electric"() -> (w203:T18)
                    n129 = local read "Referencias LS-Electric"() -> (w213:T2)
                    n130 = local read "I/O LS-Electric"() -> (w212:T9)
                    n131 = local read "Motor LS-Electric"() -> (w211:T10)
                    n132 = local read "Modbus LS-Electric"() -> (w210:T11)
                    n133 = Index Array(array=w203, index=0) -> (element=w208:T25)
                    n134 = Bundle By Name(cluster=w208, "Referencias LS-Electric"=w213, "I/O LS-Electric"=w212, "Motor LS-Electric"=w211, "Modbus LS-Electric"=w210, "Índice"=w205) -> (w204:T25)
                    n135 = Array Size(array=w203) -> (size(s)=w207:i32)
                    n136 = Insert Into Array(array=w203, index=w207, new element=w204) -> (w206:T18)
                    n137 = local write "Recetas LS Electric"(w206) -> ()
                  }
                  frame 1 {
                    # "Schneider."
                    n138 = local read "Recetas Schneider"() -> (w215:T15)
                    n139 = local read "Referencias Schneider"() -> (w222:T2)
                    n140 = local read "I/O Schneider"() -> (w221:T6)
                    n141 = Index Array(array=w215, index=0) -> (element=w219:T22)
                    n142 = Bundle By Name(cluster=w219, "Referencias Schneider"=w222, "I/O Schneider"=w221, "Índice"=w214) -> (w216:T22)
                    n143 = Array Size(array=w215) -> (size(s)=w218:i32)
                    n144 = Insert Into Array(array=w215, index=w218, new element=w216) -> (w217:T15)
                    n145 = local write "Recetas Schneider"(w217) -> ()
                  }
                  frame 2 {
                    # "Delta."
                    n146 = local read "Recetas Delta"() -> (w224:T16)
                    n147 = local read "Referencias Delta"() -> (w231:T2)
                    n148 = local read "I/O Delta"() -> (w230:T7)
                    n149 = Index Array(array=w224, index=0) -> (element=w228:T23)
                    n150 = Bundle By Name(cluster=w228, "Referencias Delta"=w231, "I/O Delta"=w230, "Índice"=w223) -> (w225:T23)
                    n151 = Array Size(array=w224) -> (size(s)=w227:i32)
                    n152 = Insert Into Array(array=w224, index=w227, new element=w225) -> (w226:T16)
                    n153 = local write "Recetas Delta"(w226) -> ()
                  }
                  frame 3 {
                    # "ABB."
                    n154 = local read "Recetas ABB"() -> (w233:T17)
                    n155 = local read "Referencias ABB"() -> (w240:T2)
                    n156 = local read "I/O ABB"() -> (w239:T8)
                    n157 = Index Array(array=w233, index=0) -> (element=w237:T24)
                    n158 = Bundle By Name(cluster=w237, "Referencias ABB"=w240, "I/O ABB"=w239, "Índice"=w232) -> (w234:T24)
                    n159 = Array Size(array=w233) -> (size(s)=w236:i32)
                    n160 = Insert Into Array(array=w233, index=w236, new element=w234) -> (w235:T17)
                    n161 = local write "Recetas ABB"(w235) -> ()
                  }
                }
                n162 = Bundle By Name(cluster=w173, "Programa nuevo"="", "Guardar"=FALSE, "Programa"=w167) -> (w176:T12)
                n163 = property class="Ring"(reference=w172, "StringsAndValues[]"=w171) -> (reference out=w170:refnum<vi>, error out=w169:errorcluster)  [unwired: 1 in]
                n164 = local write "Programa"(w176) -> ()
              }
            }
          }
        }
      }
      event "Programa.Eliminar": Value Change {
        w279 = refnum<vi> refnum  # Ring
        # "Eliminar programa seleccionado."
        n165 = event-data() -> ("NewVal"=w269:bool)  [unwired: 1 in]
        n166 = property on="Programa" class="Clust (strict)"() -> ("Controls[]"=w277:refnum<vi>[])  [unwired: 2 in, 2 out]
        n167 = local read "Programa"() -> (w274:T12)
        n168 = local read "Fabricante"() -> (w260:u32)
        n169 = local read "Recetas Allen Bradley"() -> (w266:T14)
        n170 = local read "Recetas Schneider"() -> (w265:T15)
        n171 = local read "Recetas Delta"() -> (w264:T16)
        n172 = local read "Recetas ABB"() -> (w263:T17)
        n173 = local read "Recetas LS Electric"() -> (w262:T18)
        n174 = Unbundle By Name(w274) -> ("Programa"=w281:u16)
        n175 = Index Array(array=w277, index=2) -> (element=w278:refnum<vi>)
        n176 = To More Specific Class(target class=w279, reference=w278) -> (specific class reference=w275:refnum<vi>, error out=w280:errorcluster)  [unwired: 1 in]
        n177 = Bundle("Recetas Allen Bradley"=w266, "Recetas Schneider"=w265, "Recetas Delta"=w264, "Recetas ABB"=w263, "Recetas LS Electric"=w262) -> (w261:T19)  [unwired: 1 in]
        n178 = property class="Ring"(reference=w275, error in=w280) -> ("StringsAndValues[]"=w273:T27)  [unwired: 2 out]
        n179 = Two Button Dialog(message="¿Seguro que deseas eliminar el programa seleccionado?", 1:"No." ("F button name (\"Cancel\")"), 2:"Sí." ("T button name (\"OK\")")) -> (T button?=w268:bool)
        n180 = Compound Arithmetic op=AND(w268, w269) -> (w267:bool)
        n181 = case shown="True" w267 {
          tunnel: w281 -> [_ w305]
          tunnel: w273 -> [_ w309]
          tunnel: w275 -> [_ w308]
          tunnel: [_ w307] -> _
          tunnel: [_ w306] -> _
          tunnel: w274 -> [w282 w304]
          tunnel: w261 -> [_ w299]
          tunnel: w260 -> [_ w298]
          frame False {
            # "No eliminar ningún programa."
            n182 = flat-sequence {
              tunnel: w282 -> [w287]
              tunnel: [w285] -> w283
              tunnel: w283 -> [w289]
              frame #0 {
                # "Reescribir clúster."
                n183 = Bundle By Name(cluster=w287, "Eliminar"=FALSE ("Guardar"), "Programa nuevo"="") -> (w285:T12)
                n184 = Wait (ms)(milliseconds to wait=u32 100) -> ()  [unwired: 1 out]
              }
              frame #1 {
                n185 = local write "Programa"(w289) -> ()
              }
            }
          }
          frame True {
            # "Eliminar programa seleccionado."
            n186 = flat-sequence {
              tunnel: w309 -> [w364]
              tunnel: w308 -> [w369]
              tunnel: w305 -> [w358]
              tunnel: [w368] -> w303
              tunnel: [w367] -> w302
              tunnel: w304 -> [w359]
              tunnel: [w359] -> w301
              tunnel: [w360] -> w300
              tunnel: [w378] -> w306
              tunnel: [w379] -> w307
              tunnel: w303 -> [w379]
              tunnel: w302 -> [w378]
              tunnel: w301 -> [w377]
              tunnel: w300 -> [w374]
              tunnel: [w375] -> _
              tunnel: [w374] -> w297
              frame #0 {
                # "Actualizar selector."
                n187 = Delete From Array(array=w364, length=1, index=w358) -> (array with subset deleted=w366:T27)  [unwired: 1 out]
                n188 = for {
                  tunnel: w366 -> [w373] mode=indexing
                  tunnel: [w371] -> w354 mode=indexing
                  i -> [w372]
                  n189 = Bundle By Name(cluster=w373, "Value"=w372) -> (w371:cluster{"String":string, "Value":ext})
                }
                n190 = Decrement(x=w358) -> (x-1=w363:u16)
                n191 = Array Size(array=w354) -> (size(s)=w357:i32)
                n192 = Index Array(array=w354, index=0) -> (element=w353:cluster{"String":string, "Value":ext})
                n193 = Bundle By Name(cluster=w353, "String"="", "Value"=ext 0.0) -> (w350:cluster{"String":string, "Value":ext})
                n194 = Equal To 0?(x=w358) -> (x = 0?=w362:bool)
                n195 = Build Array(w350) -> (w349:cluster{"String":string, "Value":ext}[])
                n196 = Select(t=u16 0, s=w362, f=w363) -> (s? t:f=w360:u16)
                n197 = Greater Than 0?(x=w357) -> (x > 0?=w355:bool)
                n198 = Select(t=w354, s=w355, f=w349) -> (s? t:f=w348:cluster{"String":string, "Value":ext}[])
                n199 = property class="Ring"(reference=w369, "StringsAndValues[]"=w348) -> (reference out=w368:refnum<vi>, error out=w367:errorcluster)  [unwired: 1 in]
                n200 = Wait (ms)(milliseconds to wait=u32 100) -> ()  [unwired: 1 out]
              }
              frame #1 {
                # "Actualizar clúster \"Programa\"."
                n201 = Bundle By Name(cluster=w377, "Eliminar"=FALSE, "Programa"=w374) -> (w375:T12)
                n202 = local write "Programa"(w375) -> ()
              }
            }
            n203 = flat-sequence {
              tunnel: w299 -> [w338]
              tunnel: w298 -> [w332]
              tunnel: w297 -> [w331]
              tunnel: w297 -> [w330]
              tunnel: [w330] -> w296
              tunnel: [w329] -> w295
              tunnel: w296 -> [w347]
              tunnel: w295 -> [w346]
              tunnel: [w343] -> w294
              tunnel: [w342] -> w293
              tunnel: [w341] -> w292
              tunnel: [w340] -> w291
              tunnel: [w339] -> w290
              frame #0 {
                # "Modificar arreglos de recetas."
                n204 = call "Modificación_Arreglos_Recetas.vi"("Recetas In"=w338, "Fabricante"=w332, "Índice"=w331) -> ("Recetas Out"=w329:T28)  [unwired: 8 in]
                n205 = Unbundle By Name(w329) -> ("Recetas Allen Bradley"=w337:T14, "Recetas Schneider"=w336:T15, "Recetas Delta"=w335:T16, "Recetas ABB"=w334:T17, "Recetas LS Electric"=w333:T29)
                n206 = local write "Recetas Allen Bradley"(w337) -> ()
                n207 = local write "Recetas Schneider"(w336) -> ()
                n208 = local write "Recetas Delta"(w335) -> ()
                n209 = local write "Recetas ABB"(w334) -> ()
                n210 = local write "Recetas LS Electric"(w333) -> ()
              }
              frame #1 {
                # "Buscar receta a aplicar (previa)."
                n211 = call "Búsqueda_Receta.vi"("Receta"=w346, "Índice"=w347) -> ("Recetas Out"=w344:T20, "Fabricante"=w345:u32)  [unwired: 8 in]
                n212 = local write "Fabricante"(w345) -> ()
                n213 = local write "Contenedor Fabricantes"(w345) -> ()
                n214 = Unbundle By Name(w344) -> ("Receta Allen Bradley"=w343:T21, "Receta Schneider"=w342:T22, "Receta Delta"=w341:T23, "Receta ABB"=w340:T24, "Receta LS Electric"=w339:T25)
              }
            }
            n215 = flat-sequence {
              tunnel: w294 -> [w328]
              tunnel: w293 -> [w327]
              tunnel: w292 -> [w326]
              tunnel: w291 -> [w325]
              tunnel: w290 -> [w324]
              frame #0 {
                # "Actualizar receta actual de cada marca."
                n216 = Unbundle By Name(w328) -> ("Referencias PowerFlex"=w323:T2, "I/O PowerFlex"=w322:T3, "Motor PowerFlex"=w321:T4, "Modbus PowerFlex"=w320:T5)
                n217 = Unbundle By Name(w327) -> ("Referencias Schneider"=w319:T2, "I/O Schneider"=w318:T6)
                n218 = Unbundle By Name(w326) -> ("Referencias Delta"=w317:T2, "I/O Delta"=w316:T7)
                n219 = Unbundle By Name(w325) -> ("Referencias ABB"=w315:T2, "I/O ABB"=w314:T8)
                n220 = Unbundle By Name(w324) -> ("Referencias LS-Electric"=w313:T2, "I/O LS-Electric"=w312:T9, "Motor LS-Electric"=w311:T10, "Modbus LS-Electric"=w310:T11)
                n221 = local write "Referencias PowerFlex"(w323) -> ()
                n222 = local write "I/O PowerFlex"(w322) -> ()
                n223 = local write "Motor PowerFlex"(w321) -> ()
                n224 = local write "Modbus PowerFlex"(w320) -> ()
                n225 = local write "Referencias Schneider"(w319) -> ()
                n226 = local write "I/O Schneider"(w318) -> ()
                n227 = local write "Referencias Delta"(w317) -> ()
                n228 = local write "I/O Delta"(w316) -> ()
                n229 = local write "Referencias ABB"(w315) -> ()
                n230 = local write "I/O ABB"(w314) -> ()
                n231 = local write "Referencias LS-Electric"(w313) -> ()
                n232 = local write "I/O LS-Electric"(w312) -> ()
                n233 = local write "Motor LS-Electric"(w311) -> ()
                n234 = local write "Modbus LS-Electric"(w310) -> ()
              }
            }
          }
        }
      }
      event "Programa.Programa": Value Change {
        # "Ajustar parámetros de acuerdo al programa seleccionado."
        n235 = event-data() -> ("NewVal"=w407:u16)  [unwired: 1 in]
        n236 = local read "Recetas Allen Bradley"() -> (w401:T14)
        n237 = local read "Recetas Schneider"() -> (w402:T15)
        n238 = local read "Recetas Delta"() -> (w403:T16)
        n239 = local read "Recetas ABB"() -> (w404:T17)
        n240 = local read "Recetas LS Electric"() -> (w405:T18)
        n241 = Bundle("Recetas Allen Bradley"=w401, "Recetas Schneider"=w402, "Recetas Delta"=w403, "Recetas ABB"=w404, "Recetas LS Electric"=w405) -> (w406:T19)  [unwired: 1 in]
        n242 = call "Búsqueda_Receta.vi"("Receta"=w406, "Índice"=w407) -> ("Recetas Out"=w385:T20, "Fabricante"=w400:u32)  [unwired: 8 in]
        n243 = local write "Fabricante"(w400) -> ()
        n244 = local write "Contenedor Fabricantes"(w400) -> ()
        n245 = Unbundle By Name(w385) -> ("Receta Allen Bradley"=w384:T21, "Receta Schneider"=w383:T22, "Receta Delta"=w382:T23, "Receta ABB"=w381:T24, "Receta LS Electric"=w380:T25)
        n246 = Unbundle By Name(w384) -> ("Referencias PowerFlex"=w399:T2, "I/O PowerFlex"=w398:T3, "Motor PowerFlex"=w397:T4, "Modbus PowerFlex"=w396:T5)
        n247 = Unbundle By Name(w383) -> ("Referencias Schneider"=w395:T2, "I/O Schneider"=w394:T6)
        n248 = Unbundle By Name(w382) -> ("Referencias Delta"=w393:T2, "I/O Delta"=w392:T7)
        n249 = Unbundle By Name(w381) -> ("Referencias ABB"=w391:T2, "I/O ABB"=w390:T8)
        n250 = Unbundle By Name(w380) -> ("Referencias LS-Electric"=w389:T2, "I/O LS-Electric"=w388:T9, "Motor LS-Electric"=w387:T10, "Modbus LS-Electric"=w386:T11)
        n251 = local write "Referencias PowerFlex"(w399) -> ()
        n252 = local write "I/O PowerFlex"(w398) -> ()
        n253 = local write "Motor PowerFlex"(w397) -> ()
        n254 = local write "Modbus PowerFlex"(w396) -> ()
        n255 = local write "Referencias Schneider"(w395) -> ()
        n256 = local write "I/O Schneider"(w394) -> ()
        n257 = local write "Referencias Delta"(w393) -> ()
        n258 = local write "I/O Delta"(w392) -> ()
        n259 = local write "Referencias ABB"(w391) -> ()
        n260 = local write "I/O ABB"(w390) -> ()
        n261 = local write "Referencias LS-Electric"(w389) -> ()
        n262 = local write "I/O LS-Electric"(w388) -> ()
        n263 = local write "Motor LS-Electric"(w387) -> ()
        n264 = local write "Modbus LS-Electric"(w386) -> ()
      }
    }
    n265 = local read "Salir"() -> (w68:bool)
  }
  n266 = while {
    shift-right: [w414] -> _
    shift-left: _ -> [w413]
    stop <- w415 stop-if-true
    w412 = u16 1 items=["Flanco de bajada", "Flanco de subida"] ("Subida / bajada")
    # "Máquina de estados."
    n267 = local read "Paso"() -> (w416:u32)
    n268 = local read "Download"() -> (w411:bool)
    n269 = local read "Coincidentes"() -> (w409:bool[])
    n270 = call "Flanco.vi"("Señal digital"=w411, "Subida / bajada"=w412) -> ("Señal de salida"=w410:bool)  [unwired: 9 in]
    n271 = case shown="3" w416 {
      selector: w416 -> [w420 w429 w462 w471 w540 w622 w727 w809 w908 w990 w1083 w1165 w1246]
      tunnel: [w420 w429 w462 w471 w540 w622 w727 w809 w908 w990 w1083 w1165 w1246] -> w414
      tunnel: w413 -> [_ _ w463 w472 _ _ _ _ _ _ _ _ w1247]
      tunnel: w410 -> [_ _ _ w473 _ _ _ _ _ _ _ _ w1248]
      tunnel: w409 -> [_ _ _ _ _ w618 _ w805 _ w985 _ w1160 _]
      tunnel: [w417 w425 w457 w469 w538 w617 w725 w804 w906 w983 w1081 w1158 w1244] -> w408
      frame 0, Default {
        # "Esperando escaneo."
        n272 = local read "Escanear"() -> (w421:bool)
        n273 = Initialize Array(FALSE, 4 ("dimension size")) -> (w417:bool[])
        n274 = Select(t=u32 1, s=w421, f=u32 0) -> (s? t:f=w424:u32)
        n275 = local write "Paso"(w424) -> ()
        n276 = global write "Temporales.vi" "Escanear"(w421) -> ()
      }
      frame 1 {
        # "Buscando variador."
        n277 = flat-sequence {
          tunnel: [w430] -> w426
          tunnel: [w435] -> w428
          tunnel: [w434] -> w427
          tunnel: w426 -> [w434]
          tunnel: w428 -> [_]
          tunnel: [w438] -> w425
          tunnel: w427 -> [w438]
          frame #0 {
            # "Acarrear variables."
            n278 = local read "Escanear"() -> (w433:bool)
            n279 = Initialize Array(FALSE, 4 ("dimension size")) -> (w430:bool[])
            n280 = global write "Temporales.vi" "Escanear"(w433) -> ()
          }
          frame #1 {
            # "Cerrar puerto."
            n281 = local read "Instancia Modbus"() -> (w437:refnum<class "Modbus Master.lvclass">)
            n282 = call-dynamic "Shutdown.vi"("error in"=errorcluster {"status"=FALSE, "code"=0, "source"=""}, "Modbus master in"=w437) -> ("error out"=w435:errorcluster)  [unwired: 9 in]
          }
          frame #2 {
            # "Buscando variador."
            n283 = local read "Puerto COM"() -> (w446:refnum<visa-resource-name>)
            n284 = local read "Fabricante"() -> (w442:u32)
            n285 = call "Escáner.vi"("Fabricante"=w442, "Puerto COM"=w446) -> ("error out"=w444:errorcluster, "Datos"=w439:i32[], "VFD encontrado"=w441:bool, "Modbus master out"=w443:refnum<class "Modbus Master.lvclass">, "Timeout"=w445:i32)  [unwired: 4 in]
            n286 = local write "Instancia Modbus"(w443) -> ()
            n287 = local write "Error Modbus"(w444) -> ()
            n288 = local write "Timeout"(w445) -> ()
            n289 = case shown="1" w442 {
              tunnel: w441 -> [w451 w456]
              tunnel: [w447 w453] -> w440
              tunnel: w439 -> [w448 w452]
              tunnel: [w448 w452] -> _
              frame 0, Default {
                # "Allen Bradley."
                n290 = Select(t=u32 3, s=w451, f=u32 2 ("t")) -> (s? t:f=w447:u32)
              }
              frame 1 {
                # "Schneider."
                n291 = Select(t=u32 1, s=w456, f=u32 2 ("t")) -> (s? t:f=w453:u32)
              }
            }
            n292 = local write "Paso"(w440) -> ()
          }
        }
      }
      frame 2 {
        # "Variador no encontrado."
        n293 = local read "Escanear"() -> (w467:bool)
        n294 = Initialize Array(FALSE, 4 ("dimension size")) -> (w457:bool[])
        n295 = Equal?(x=w463, y=u32 1) -> (x = y?=w461:bool)
        n296 = case shown="True" w461 {
          frame False {
            # "Nada."
          }
          frame True {
            # "Liberar variable."
            n297 = local write "Escanear"(FALSE) -> ()
          }
        }
        n298 = Select(t=u32 1, s=w467, f=u32 2) -> (s? t:f=w466:u32)
        n299 = local write "Paso"(w466) -> ()
      }
      frame 3 {
        # "Control y monitoreo de variador: Esperando a configurar."
        n300 = local read "Frecuencia"() -> (w478:dbl)
        n301 = local read "Instancia Modbus"() -> (w487:refnum<class "Modbus Master.lvclass">)
        n302 = local read "Fabricante"() -> (w486:u32)
        n303 = local read "Run"() -> (w481:bool)
        n304 = local read "Sentido"() -> (w480:bool)
        n305 = local read "Reset"() -> (w479:bool)
        n306 = local read "Salidas digitales"() -> (w477:cluster{"Salida":bool, "Etiqueta":string}[])
        n307 = local read "Entradas digitales"() -> (w482:cluster{"Estado":bool, "Etiqueta":string}[])
        n308 = Not Equal?(x=w472, y=w471) -> (x != y?=w470:bool)
        n309 = for {
          tunnel: w477 -> [w532] mode=indexing
          tunnel: [w531] -> w476 mode=indexing
          n310 = Unbundle By Name(w532) -> ("Salida"=w531:bool)
        }
        n311 = case shown="False" w473 {
          tunnel: [w490 w497] -> w475
          tunnel: [w489 w494] -> w469
          frame False {
            # "Permanecer en este paso."
            n312 = local read "Escanear"() -> (w493:bool)
            n313 = local read "Coincidentes"() -> (w489:bool[])
            n314 = Select(t=1, s=w493, f=3) -> (s? t:f=w490:i32)
          }
          frame True {
            # "Descargar parámetros."
            n315 = local read "Fabricante"() -> (w498:u32)
            n316 = case shown="4" w498 {
              tunnel: [w499 w515] -> w497
              frame 0, Default {
                # "Allen Bradley."
                n317 = local read "Referencias PowerFlex"() -> (w509:T2)
                n318 = local read "I/O PowerFlex"() -> (w508:T3)
                n319 = local read "Motor PowerFlex"() -> (w507:T4)
                n320 = local read "Modbus PowerFlex"() -> (w506:T5)
                n321 = Unbundle By Name(w509) -> ("Descargar"=w505:bool)
                n322 = Unbundle By Name(w508) -> ("Descargar"=w504:bool)
                n323 = Unbundle By Name(w507) -> ("Descargar"=w503:bool)
                n324 = Unbundle By Name(w506) -> ("Descargar"=w502:bool)
                n325 = Build Array(w505, w504, w503, w502) -> (w501:bool[])
                n326 = Boolean Array To Number(Boolean array=w501) -> (number=w500:u32)
                n327 = case shown="8" w500 {
                  tunnel: [3 4 5 6 7] -> w499
                  frame 0, Default {
                    # "Nada."
                  }
                  frame 1, 3, 5, 7, 9, 11, 13, 15 {
                    # "Configurar referencias."
                  }
                  frame 2, 6, 10, 14 {
                    # "Configurar entradas y salidas."
                  }
                  frame 4, 12 {
                    # "Configurar motor."
                  }
                  frame 8 {
                    # "Configurar Modbus."
                  }
                }
              }
              frame 4 {
                # "LS-Electric."
                n328 = local read "Referencias LS-Electric"() -> (w525:T2)
                n329 = local read "I/O LS-Electric"() -> (w524:T9)
                n330 = local read "Motor LS-Electric"() -> (w523:T10)
                n331 = local read "Modbus LS-Electric"() -> (w522:T11)
                n332 = Unbundle By Name(w525) -> ("Descargar"=w521:bool)
                n333 = Unbundle By Name(w524) -> ("Descargar"=w520:bool)
                n334 = Unbundle By Name(w523) -> ("Descargar"=w519:bool)
                n335 = Unbundle By Name(w522) -> ("Descargar"=w518:bool)
                n336 = Build Array(w521, w520, w519, w518) -> (w517:bool[])
                n337 = Boolean Array To Number(Boolean array=w517) -> (number=w516:u32)
                n338 = case shown="0, Default" w516 {
                  tunnel: [3 4 5 6 7] -> w515
                  frame 0, Default {
                    # "Nada."
                  }
                  frame 1, 3, 5, 7, 9, 11, 13, 15 {
                    # "Configurar referencias."
                  }
                  frame 2, 6, 10, 14 {
                    # "Configurar entradas y salidas."
                  }
                  frame 4, 12 {
                    # "Configurar motor."
                  }
                  frame 8 {
                    # "Configurar Modbus."
                  }
                }
              }
            }
            n339 = Initialize Array(FALSE, 4 ("dimension size")) -> (w494:bool[])
          }
        }
        n340 = case shown="True" w470 {
          frame False {
            # "Nada."
          }
          frame True {
            # "Reiniciar variable."
            n341 = local write "Escanear"(FALSE ("Download")) -> ()
          }
        }
        n342 = call "Comunicación_VFD.vi"("Salidas digitales"=w476, "Reset"=w479, "Frecuencia"=w478, "Sentido"=w480, "Run"=w481, "Fabricante"=w486, "Instancia Modbus"=w487) -> ("Error Modbus"=w485:errorcluster, "Entradas digitales"=w484:bool[])  [unwired: 3 in]
        n343 = for {
          tunnel: w484 -> [w536] mode=indexing
          tunnel: w482 -> [w537] mode=indexing
          tunnel: [w534] -> w483 mode=indexing
          tunnel: w482 -> [w533] mode=indexing
          n344 = Unbundle By Name(w537) -> ("Etiqueta"=w535:string)
          n345 = Bundle By Name(cluster=w533, "Estado"=w536, "Etiqueta"=w535) -> (w534:cluster{"Estado":bool, "Etiqueta":string})
        }
        n346 = local write "Error Modbus"(w485) -> ()
        n347 = local write "Entradas digitales"(w483) -> ()
        n348 = local write "Iteración"(u32 0 ("Paso")) -> ()
        n349 = local write "Paso"(w475) -> ()
      }
      frame 4 {
        # "Descargar parámetros a variador (Referencias de control)."
        n350 = local read "Fabricante"() -> (w539:u32)
        n351 = case shown="0, Default" w539 {
          selector: w539 -> [w543 w580]
          frame 0, Default {
            # "Allen Bradley."
            n352 = for {
              N: 10 -> [_]
              tunnel: w543 -> [w548]
              tunnel: [5] -> w542
              tunnel: [FALSE] -> w541
              # "10 intentos/iteraciones."
              n353 = local read "Iteración"() -> (w561:u32)
              n354 = local read "Instancia Modbus"() -> (w577:refnum<class "Modbus Master.lvclass">)
              n355 = local read "Referencias PowerFlex"() -> (w549:T2)
              n356 = local read "Referencias Schneider"() -> (w576:T2)
              n357 = local read "Referencias Delta"() -> (w573:T2)
              n358 = local read "Referencias ABB"() -> (w572:T2)
              n359 = local read "Referencias LS-Electric"() -> (w574:T2)
              n360 = local read "I/O PowerFlex"() -> (w557:T3)
              n361 = local read "I/O Schneider"() -> (w570:T6)
              n362 = local read "I/O Delta"() -> (w569:T7)
              n363 = local read "I/O ABB"() -> (w568:T8)
              n364 = local read "I/O LS-Electric"() -> (w567:T9)
              n365 = local read "Motor PowerFlex"() -> (w554:T4)
              n366 = local read "Motor LS-Electric"() -> (w565:T10)
              n367 = local read "Modbus PowerFlex"() -> (w551:T5)
              n368 = local read "Modbus LS-Electric"() -> (w563:T11)
              n369 = Bundle By Name(cluster=w549, "Descargar"=TRUE) -> (w559:T2)
              n370 = Bundle By Name(cluster=w557, "Descargar"=FALSE) -> (w556:T3)
              n371 = Bundle By Name(cluster=w554, "Descargar"=FALSE) -> (w553:T4)
              n372 = Bundle By Name(cluster=w551, "Descargar"=FALSE) -> (w550:T5)
              n373 = Bundle("Referencias PowerFlex"=w559, "Referencias Schneider"=w576, "Referencias Delta"=w573, "Referencias ABB"=w572, "Referencias LS-Electric"=w574) -> (w575:T30)  [unwired: 1 in]
              n374 = Bundle("I/O PowerFlex"=w556, "I/O Schneider"=w570, "I/O Delta"=w569, "I/O ABB"=w568, "I/O LS-Electric"=w567) -> (w571:T31)  [unwired: 1 in]
              n375 = Bundle("Motor PowerFlex"=w553, "Motor LS-Electric"=w565) -> (w566:T32)  [unwired: 1 in]
              n376 = Bundle("Modbus PowerFlex"=w550, "Modbus LS-Electric"=w563) -> (w564:T33)  [unwired: 1 in]
              n377 = call "Descarga_VFD.vi"("Fabricante"=w548, "Modbus"=w564, "Iteraciones (In)"=w561, "Motor"=w566, "I/O"=w571, "Referencias"=w575, "Instancia Modbus"=w577) -> ("Error Modbus"=w562:errorcluster, "Iteraciones (Out)"=w545:u32)  [unwired: 3 in]
              n378 = local write "Error Modbus"(w562) -> ()
              n379 = local write "Iteración"(w545) -> ()
            }
            n380 = local write "Download"(w541) -> ()
            n381 = local write "Paso"(w542) -> ()
          }
          frame 4 {
            # "LS-Electric."
            n382 = for {
              N: 10 -> [_]
              tunnel: w580 -> [w585]
              tunnel: [5] -> w579
              tunnel: [FALSE] -> w578
              # "10 intentos/iteraciones."
              n383 = local read "Iteración"() -> (w602:u32)
              n384 = local read "Instancia Modbus"() -> (w614:refnum<class "Modbus Master.lvclass">)
              n385 = local read "Referencias PowerFlex"() -> (w597:T2)
              n386 = local read "Referencias Schneider"() -> (w613:T2)
              n387 = local read "Referencias Delta"() -> (w611:T2)
              n388 = local read "Referencias ABB"() -> (w610:T2)
              n389 = local read "Referencias LS-Electric"() -> (w596:T2)
              n390 = local read "I/O PowerFlex"() -> (w594:T3)
              n391 = local read "I/O Schneider"() -> (w608:T6)
              n392 = local read "I/O Delta"() -> (w607:T7)
              n393 = local read "I/O ABB"() -> (w606:T8)
              n394 = local read "I/O LS-Electric"() -> (w593:T9)
              n395 = local read "Motor PowerFlex"() -> (w591:T4)
              n396 = local read "Motor LS-Electric"() -> (w590:T10)
              n397 = local read "Modbus PowerFlex"() -> (w588:T5)
              n398 = local read "Modbus LS-Electric"() -> (w587:T11)
              n399 = Bundle By Name(cluster=w596, "Descargar"=TRUE) -> (w595:T2)
              n400 = Bundle By Name(cluster=w593, "Descargar"=FALSE) -> (w592:T9)
              n401 = Bundle By Name(cluster=w590, "Descargar"=FALSE) -> (w589:T10)
              n402 = Bundle By Name(cluster=w587, "Descargar"=FALSE) -> (w586:T11)
              n403 = Bundle("Referencias PowerFlex"=w597, "Referencias Schneider"=w613, "Referencias Delta"=w611, "Referencias ABB"=w610, "Referencias LS-Electric"=w595) -> (w612:T30)  [unwired: 1 in]
              n404 = Bundle("I/O PowerFlex"=w594, "I/O Schneider"=w608, "I/O Delta"=w607, "I/O ABB"=w606, "I/O LS-Electric"=w592) -> (w609:T31)  [unwired: 1 in]
              n405 = Bundle("Motor PowerFlex"=w591, "Motor LS-Electric"=w589) -> (w605:T32)  [unwired: 1 in]
              n406 = Bundle("Modbus PowerFlex"=w588, "Modbus LS-Electric"=w586) -> (w604:T33)  [unwired: 1 in]
              n407 = call "Descarga_VFD.vi"("Fabricante"=w585, "Modbus"=w604, "Iteraciones (In)"=w602, "Motor"=w605, "I/O"=w609, "Referencias"=w612, "Instancia Modbus"=w614) -> ("Error Modbus"=w603:errorcluster, "Iteraciones (Out)"=w582:u32)  [unwired: 3 in]
              n408 = local write "Error Modbus"(w603) -> ()
              n409 = local write "Iteración"(w582) -> ()
            }
            n410 = local write "Download"(w578) -> ()
            n411 = local write "Paso"(w579) -> ()
          }
        }
        n412 = local read "Coincidentes"() -> (w538:bool[])
      }
      frame 5 {
        # "Revisar parámetros de variador (Referencias de control)."
        n413 = local read "Fabricante"() -> (w621:u32)
        n414 = case shown="0, Default" w621 {
          selector: w621 -> [w626 w677]
          tunnel: [w623 w674] -> w619
          frame 0, Default {
            # "Allen Bradley."
            n415 = for {
              N: 10 -> [_]
              tunnel: w626 -> [w632]
              tunnel: [w631] -> w625
              tunnel: [FALSE] -> w624
              tunnel: [w628] -> w623
              # "10 intentos/iteraciones."
              n416 = local read "Iteración"() -> (w653:u32)
              n417 = local read "Instancia Modbus"() -> (w669:refnum<class "Modbus Master.lvclass">)
              n418 = local read "Referencias PowerFlex"() -> (w633:T2)
              n419 = local read "Referencias Schneider"() -> (w668:T2)
              n420 = local read "Referencias Delta"() -> (w665:T2)
              n421 = local read "Referencias ABB"() -> (w664:T2)
              n422 = local read "Referencias LS-Electric"() -> (w666:T2)
              n423 = local read "I/O PowerFlex"() -> (w649:T3)
              n424 = local read "I/O Schneider"() -> (w662:T6)
              n425 = local read "I/O Delta"() -> (w661:T7)
              n426 = local read "I/O ABB"() -> (w660:T8)
              n427 = local read "I/O LS-Electric"() -> (w659:T9)
              n428 = local read "Motor PowerFlex"() -> (w646:T4)
              n429 = local read "Motor LS-Electric"() -> (w657:T10)
              n430 = local read "Modbus PowerFlex"() -> (w643:T5)
              n431 = local read "Modbus LS-Electric"() -> (w655:T11)
              n432 = local read "I/O PowerFlex"() -> (w634:T3)
              n433 = local read "Motor PowerFlex"() -> (w635:T4)
              n434 = local read "Modbus PowerFlex"() -> (w636:T5)
              n435 = Bundle By Name(cluster=w633, "Descargar"=TRUE) -> (w651:T2)
              n436 = Bundle By Name(cluster=w649, "Descargar"=FALSE) -> (w648:T3)
              n437 = Bundle By Name(cluster=w646, "Descargar"=FALSE) -> (w645:T4)
              n438 = Bundle By Name(cluster=w643, "Descargar"=FALSE) -> (w642:T5)
              n439 = Unbundle By Name(w634) -> ("Descargar"=w637:bool)
              n440 = Unbundle By Name(w635) -> ("Descargar"=w638:bool)
              n441 = Unbundle By Name(w636) -> ("Descargar"=w639:bool)
              n442 = Build Array(w637, w638, w639) -> (w640:bool[])
              n443 = Boolean Array To Number(Boolean array=w640) -> (number=w641:u32)
              n444 = Bundle("Referencias PowerFlex"=w651, "Referencias Schneider"=w668, "Referencias Delta"=w665, "Referencias ABB"=w664, "Referencias LS-Electric"=w666) -> (w667:T30)  [unwired: 1 in]
              n445 = Bundle("I/O PowerFlex"=w648, "I/O Schneider"=w662, "I/O Delta"=w661, "I/O ABB"=w660, "I/O LS-Electric"=w659) -> (w663:T31)  [unwired: 1 in]
              n446 = Bundle("Motor PowerFlex"=w645, "Motor LS-Electric"=w657) -> (w658:T32)  [unwired: 1 in]
              n447 = Bundle("Modbus PowerFlex"=w642, "Modbus LS-Electric"=w655) -> (w656:T33)  [unwired: 1 in]
              n448 = case shown="0, Default" w641 {
                tunnel: [12 6 8 10] -> w631
                frame 0, Default {
                  # "Control de VFD."
                }
                frame 1, 3, 5, 7 {
                  # "Configurar entradas y salidas."
                }
                frame 2, 6 {
                  # "Configurar motor."
                }
                frame 4 {
                  # "Configurar Modbus."
                }
              }
              n449 = call "Revisión_VFD.vi"("Fabricante"=w632, "Modbus"=w656, "Iteración (In)"=w653, "Motor"=w658, "I/O"=w663, "Referencias"=w667, "Instancia Modbus"=w669) -> ("Error Modbus"=w654:errorcluster, "Iteración (Out)"=w629:u32, "Coincidentes"=w628:bool[])  [unwired: 2 in]
              n450 = local write "Error Modbus"(w654) -> ()
              n451 = local write "Iteración"(w629) -> ()
            }
            n452 = local write "Download"(w624) -> ()
            n453 = local write "Paso"(w625) -> ()
          }
          frame 4 {
            # "LS-Electric."
            n454 = for {
              N: 10 -> [_]
              tunnel: w677 -> [w683]
              tunnel: [w682] -> w676
              tunnel: [FALSE] -> w675
              tunnel: [w679] -> w674
              # "10 intentos/iteraciones."
              n455 = local read "Iteración"() -> (w708:u32)
              n456 = local read "Instancia Modbus"() -> (w720:refnum<class "Modbus Master.lvclass">)
              n457 = local read "Referencias PowerFlex"() -> (w695:T2)
              n458 = local read "Referencias Schneider"() -> (w719:T2)
              n459 = local read "Referencias Delta"() -> (w717:T2)
              n460 = local read "Referencias ABB"() -> (w716:T2)
              n461 = local read "Referencias LS-Electric"() -> (w694:T2)
              n462 = local read "I/O PowerFlex"() -> (w692:T3)
              n463 = local read "I/O Schneider"() -> (w714:T6)
              n464 = local read "I/O Delta"() -> (w713:T7)
              n465 = local read "I/O ABB"() -> (w712:T8)
              n466 = local read "I/O LS-Electric"() -> (w691:T9)
              n467 = local read "Motor PowerFlex"() -> (w689:T4)
              n468 = local read "Motor LS-Electric"() -> (w688:T10)
              n469 = local read "Modbus PowerFlex"() -> (w686:T5)
              n470 = local read "Modbus LS-Electric"() -> (w685:T11)
              n471 = local read "I/O LS-Electric"() -> (w696:T9)
              n472 = local read "Motor LS-Electric"() -> (w697:T10)
              n473 = local read "Modbus LS-Electric"() -> (w698:T11)
              n474 = Bundle By Name(cluster=w694, "Descargar"=TRUE) -> (w693:T2)
              n475 = Bundle By Name(cluster=w691, "Descargar"=FALSE) -> (w690:T9)
              n476 = Bundle By Name(cluster=w688, "Descargar"=FALSE) -> (w687:T10)
              n477 = Bundle By Name(cluster=w685, "Descargar"=FALSE) -> (w684:T11)
              n478 = Unbundle By Name(w696) -> ("Descargar"=w699:bool)
              n479 = Unbundle By Name(w697) -> ("Descargar"=w700:bool)
              n480 = Unbundle By Name(w698) -> ("Descargar"=w701:bool)
              n481 = Build Array(w699, w700, w701) -> (w702:bool[])
              n482 = Boolean Array To Number(Boolean array=w702) -> (number=w703:u32)
              n483 = Bundle("Referencias PowerFlex"=w695, "Referencias Schneider"=w719, "Referencias Delta"=w717, "Referencias ABB"=w716, "Referencias LS-Electric"=w693) -> (w718:T30)  [unwired: 1 in]
              n484 = Bundle("I/O PowerFlex"=w692, "I/O Schneider"=w714, "I/O Delta"=w713, "I/O ABB"=w712, "I/O LS-Electric"=w690) -> (w715:T31)  [unwired: 1 in]
              n485 = Bundle("Motor PowerFlex"=w689, "Motor LS-Electric"=w687) -> (w711:T32)  [unwired: 1 in]
              n486 = Bundle("Modbus PowerFlex"=w686, "Modbus LS-Electric"=w684) -> (w710:T33)  [unwired: 1 in]
              n487 = case shown="0, Default" w703 {
                tunnel: [12 6 8 10] -> w682
                frame 0, Default {
                  # "Control de VFD."
                }
                frame 1, 3, 5, 7 {
                  # "Configurar entradas y salidas."
                }
                frame 2, 6 {
                  # "Configurar motor."
                }
                frame 4 {
                  # "Configurar Modbus."
                }
              }
              n488 = call "Revisión_VFD.vi"("Fabricante"=w683, "Modbus"=w710, "Iteración (In)"=w708, "Motor"=w711, "I/O"=w715, "Referencias"=w718, "Instancia Modbus"=w720) -> ("Error Modbus"=w709:errorcluster, "Iteración (Out)"=w680:u32, "Coincidentes"=w679:bool[])  [unwired: 2 in]
              n489 = local write "Error Modbus"(w709) -> ()
              n490 = local write "Iteración"(w680) -> ()
            }
            n491 = local write "Download"(w675) -> ()
            n492 = local write "Paso"(w676) -> ()
          }
        }
        n493 = Index Array(array=w619, index=0) -> (element=w616:bool)
        n494 = Replace Array Subset(array=w618, new element=w616, index=0) -> (w617:bool[])
      }
      frame 6 {
        # "Descargar parámetros a variador (Función de entradas y salidas)."
        n495 = local read "Fabricante"() -> (w726:u32)
        n496 = case shown="0, Default" w726 {
          selector: w726 -> [w730 w767]
          frame 0, Default {
            # "Allen Bradley."
            n497 = for {
              N: 10 -> [_]
              tunnel: w730 -> [w735]
              tunnel: [7] -> w729
              tunnel: [FALSE] -> w728
              # "10 intentos/iteraciones."
              n498 = local read "Iteración"() -> (w748:u32)
              n499 = local read "Instancia Modbus"() -> (w764:refnum<class "Modbus Master.lvclass">)
              n500 = local read "Referencias PowerFlex"() -> (w736:T2)
              n501 = local read "Referencias Schneider"() -> (w763:T2)
              n502 = local read "Referencias Delta"() -> (w760:T2)
              n503 = local read "Referencias ABB"() -> (w759:T2)
              n504 = local read "Referencias LS-Electric"() -> (w761:T2)
              n505 = local read "I/O PowerFlex"() -> (w744:T3)
              n506 = local read "I/O Schneider"() -> (w757:T6)
              n507 = local read "I/O Delta"() -> (w756:T7)
              n508 = local read "I/O ABB"() -> (w755:T8)
              n509 = local read "I/O LS-Electric"() -> (w754:T9)
              n510 = local read "Motor PowerFlex"() -> (w741:T4)
              n511 = local read "Motor LS-Electric"() -> (w752:T10)
              n512 = local read "Modbus PowerFlex"() -> (w738:T5)
              n513 = local read "Modbus LS-Electric"() -> (w750:T11)
              n514 = Bundle By Name(cluster=w736, "Descargar"=FALSE) -> (w746:T2)
              n515 = Bundle By Name(cluster=w744, "Descargar"=TRUE) -> (w743:T3)
              n516 = Bundle By Name(cluster=w741, "Descargar"=FALSE) -> (w740:T4)
              n517 = Bundle By Name(cluster=w738, "Descargar"=FALSE) -> (w737:T5)
              n518 = Bundle("Referencias PowerFlex"=w746, "Referencias Schneider"=w763, "Referencias Delta"=w760, "Referencias ABB"=w759, "Referencias LS-Electric"=w761) -> (w762:T30)  [unwired: 1 in]
              n519 = Bundle("I/O PowerFlex"=w743, "I/O Schneider"=w757, "I/O Delta"=w756, "I/O ABB"=w755, "I/O LS-Electric"=w754) -> (w758:T31)  [unwired: 1 in]
              n520 = Bundle("Motor PowerFlex"=w740, "Motor LS-Electric"=w752) -> (w753:T32)  [unwired: 1 in]
              n521 = Bundle("Modbus PowerFlex"=w737, "Modbus LS-Electric"=w750) -> (w751:T33)  [unwired: 1 in]
              n522 = call "Descarga_VFD.vi"("Fabricante"=w735, "Modbus"=w751, "Iteraciones (In)"=w748, "Motor"=w753, "I/O"=w758, "Referencias"=w762, "Instancia Modbus"=w764) -> ("Error Modbus"=w749:errorcluster, "Iteraciones (Out)"=w732:u32)  [unwired: 3 in]
              n523 = local write "Error Modbus"(w749) -> ()
              n524 = local write "Iteración"(w732) -> ()
            }
            n525 = local write "Download"(w728) -> ()
            n526 = local write "Paso"(w729) -> ()
          }
          frame 4 {
            # "LS-Electric."
            n527 = for {
              N: 10 -> [_]
              tunnel: w767 -> [w772]
              tunnel: [7] -> w766
              tunnel: [FALSE] -> w765
              # "10 intentos/iteraciones."
              n528 = local read "Iteración"() -> (w789:u32)
              n529 = local read "Instancia Modbus"() -> (w801:refnum<class "Modbus Master.lvclass">)
              n530 = local read "Referencias PowerFlex"() -> (w784:T2)
              n531 = local read "Referencias Schneider"() -> (w800:T2)
              n532 = local read "Referencias Delta"() -> (w798:T2)
              n533 = local read "Referencias ABB"() -> (w797:T2)
              n534 = local read "Referencias LS-Electric"() -> (w783:T2)
              n535 = local read "I/O PowerFlex"() -> (w781:T3)
              n536 = local read "I/O Schneider"() -> (w795:T6)
              n537 = local read "I/O Delta"() -> (w794:T7)
              n538 = local read "I/O ABB"() -> (w793:T8)
              n539 = local read "I/O LS-Electric"() -> (w780:T9)
              n540 = local read "Motor PowerFlex"() -> (w778:T4)
              n541 = local read "Motor LS-Electric"() -> (w777:T10)
              n542 = local read "Modbus PowerFlex"() -> (w775:T5)
              n543 = local read "Modbus LS-Electric"() -> (w774:T11)
              n544 = Bundle By Name(cluster=w783, "Descargar"=FALSE) -> (w782:T2)
              n545 = Bundle By Name(cluster=w780, "Descargar"=TRUE) -> (w779:T9)
              n546 = Bundle By Name(cluster=w777, "Descargar"=FALSE) -> (w776:T10)
              n547 = Bundle By Name(cluster=w774, "Descargar"=FALSE) -> (w773:T11)
              n548 = Bundle("Referencias PowerFlex"=w784, "Referencias Schneider"=w800, "Referencias Delta"=w798, "Referencias ABB"=w797, "Referencias LS-Electric"=w782) -> (w799:T30)  [unwired: 1 in]
              n549 = Bundle("I/O PowerFlex"=w781, "I/O Schneider"=w795, "I/O Delta"=w794, "I/O ABB"=w793, "I/O LS-Electric"=w779) -> (w796:T31)  [unwired: 1 in]
              n550 = Bundle("Motor PowerFlex"=w778, "Motor LS-Electric"=w776) -> (w792:T32)  [unwired: 1 in]
              n551 = Bundle("Modbus PowerFlex"=w775, "Modbus LS-Electric"=w773) -> (w791:T33)  [unwired: 1 in]
              n552 = call "Descarga_VFD.vi"("Fabricante"=w772, "Modbus"=w791, "Iteraciones (In)"=w789, "Motor"=w792, "I/O"=w796, "Referencias"=w799, "Instancia Modbus"=w801) -> ("Error Modbus"=w790:errorcluster, "Iteraciones (Out)"=w769:u32)  [unwired: 3 in]
              n553 = local write "Error Modbus"(w790) -> ()
              n554 = local write "Iteración"(w769) -> ()
            }
            n555 = local write "Download"(w765) -> ()
            n556 = local write "Paso"(w766) -> ()
          }
        }
        n557 = local read "Coincidentes"() -> (w725:bool[])
      }
      frame 7 {
        # "Revisar parámetros de variador (Función de entradas y salidas)."
        n558 = local read "Fabricante"() -> (w808:u32)
        n559 = case shown="0, Default" w808 {
          selector: w808 -> [w813 w861]
          tunnel: [w810 w858] -> w806
          frame 0, Default {
            # "Allen Bradley."
            n560 = for {
              N: 10 -> [_]
              tunnel: w813 -> [w820]
              tunnel: [w819] -> w812
              tunnel: [FALSE] -> w811
              tunnel: [w816] -> w810
              # "10 intentos/iteraciones."
              n561 = local read "Iteración"() -> (w839:u32)
              n562 = local read "Instancia Modbus"() -> (w854:refnum<class "Modbus Master.lvclass">)
              n563 = local read "Referencias PowerFlex"() -> (w821:T2)
              n564 = local read "Referencias Schneider"() -> (w853:T2)
              n565 = local read "Referencias Delta"() -> (w850:T2)
              n566 = local read "Referencias ABB"() -> (w849:T2)
              n567 = local read "Referencias LS-Electric"() -> (w851:T2)
              n568 = local read "I/O PowerFlex"() -> (w835:T3)
              n569 = local read "I/O Schneider"() -> (w848:T6)
              n570 = local read "I/O Delta"() -> (w847:T7)
              n571 = local read "I/O ABB"() -> (w846:T8)
              n572 = local read "I/O LS-Electric"() -> (w845:T9)
              n573 = local read "Motor PowerFlex"() -> (w832:T4)
              n574 = local read "Motor LS-Electric"() -> (w843:T10)
              n575 = local read "Modbus PowerFlex"() -> (w829:T5)
              n576 = local read "Modbus LS-Electric"() -> (w841:T11)
              n577 = local read "Motor PowerFlex"() -> (w822:T4)
              n578 = local read "Modbus PowerFlex"() -> (w823:T5)
              n579 = Bundle By Name(cluster=w821, "Descargar"=FALSE) -> (w837:T2)
              n580 = Bundle By Name(cluster=w835, "Descargar"=TRUE) -> (w834:T3)
              n581 = Bundle By Name(cluster=w832, "Descargar"=FALSE) -> (w831:T4)
              n582 = Bundle By Name(cluster=w829, "Descargar"=FALSE) -> (w828:T5)
              n583 = Unbundle By Name(w822) -> ("Descargar"=w824:bool)
              n584 = Unbundle By Name(w823) -> ("Descargar"=w825:bool)
              n585 = Build Array(w824, w825) -> (w826:bool[])
              n586 = Boolean Array To Number(Boolean array=w826) -> (number=w827:u32)
              n587 = Bundle("Referencias PowerFlex"=w837, "Referencias Schneider"=w853, "Referencias Delta"=w850, "Referencias ABB"=w849, "Referencias LS-Electric"=w851) -> (w852:T30)  [unwired: 1 in]
              n588 = Bundle("I/O PowerFlex"=w834, "I/O Schneider"=w848, "I/O Delta"=w847, "I/O ABB"=w846, "I/O LS-Electric"=w845) -> (w815:T31)  [unwired: 1 in]
              n589 = Bundle("Motor PowerFlex"=w831, "Motor LS-Electric"=w843) -> (w844:T32)  [unwired: 1 in]
              n590 = Bundle("Modbus PowerFlex"=w828, "Modbus LS-Electric"=w841) -> (w842:T33)  [unwired: 1 in]
              n591 = case shown="0, Default" w827 {
                tunnel: [12 8 10] -> w819
                frame 0, Default {
                  # "Control de VFD."
                }
                frame 1, 3 {
                  # "Configurar motor."
                }
                frame 2 {
                  # "Configurar Modbus."
                }
              }
              n592 = call "Revisión_VFD.vi"("Fabricante"=w820, "Modbus"=w842, "Iteración (In)"=w839, "Motor"=w844, "I/O"=w815, "Referencias"=w852, "Instancia Modbus"=w854) -> ("Error Modbus"=w840:errorcluster, "Iteración (Out)"=w817:u32, "Coincidentes"=w816:bool[])  [unwired: 2 in]
              n593 = local write "Error Modbus"(w840) -> ()
              n594 = local write "Iteración"(w817) -> ()
            }
            n595 = local write "Download"(w811) -> ()
            n596 = local write "Paso"(w812) -> ()
          }
          frame 4 {
            # "LS-Electric."
            n597 = for {
              N: 10 -> [_]
              tunnel: w861 -> [w867]
              tunnel: [w866] -> w860
              tunnel: [FALSE] -> w859
              tunnel: [w863] -> w858
              # "10 intentos/iteraciones."
              n598 = local read "Iteración"() -> (w890:u32)
              n599 = local read "Instancia Modbus"() -> (w902:refnum<class "Modbus Master.lvclass">)
              n600 = local read "Referencias PowerFlex"() -> (w879:T2)
              n601 = local read "Referencias Schneider"() -> (w901:T2)
              n602 = local read "Referencias Delta"() -> (w899:T2)
              n603 = local read "Referencias ABB"() -> (w898:T2)
              n604 = local read "Referencias LS-Electric"() -> (w878:T2)
              n605 = local read "I/O PowerFlex"() -> (w876:T3)
              n606 = local read "I/O Schneider"() -> (w896:T6)
              n607 = local read "I/O Delta"() -> (w895:T7)
              n608 = local read "I/O ABB"() -> (w894:T8)
              n609 = local read "I/O LS-Electric"() -> (w875:T9)
              n610 = local read "Motor PowerFlex"() -> (w873:T4)
              n611 = local read "Motor LS-Electric"() -> (w872:T10)
              n612 = local read "Modbus PowerFlex"() -> (w870:T5)
              n613 = local read "Modbus LS-Electric"() -> (w869:T11)
              n614 = local read "Motor LS-Electric"() -> (w880:T10)
              n615 = local read "Modbus LS-Electric"() -> (w881:T11)
              n616 = Bundle By Name(cluster=w878, "Descargar"=FALSE) -> (w877:T2)
              n617 = Bundle By Name(cluster=w875, "Descargar"=TRUE) -> (w874:T9)
              n618 = Bundle By Name(cluster=w872, "Descargar"=FALSE) -> (w871:T10)
              n619 = Bundle By Name(cluster=w869, "Descargar"=FALSE) -> (w868:T11)
              n620 = Unbundle By Name(w880) -> ("Descargar"=w882:bool)
              n621 = Unbundle By Name(w881) -> ("Descargar"=w883:bool)
              n622 = Build Array(w882, w883) -> (w884:bool[])
              n623 = Boolean Array To Number(Boolean array=w884) -> (number=w885:u32)
              n624 = Bundle("Referencias PowerFlex"=w879, "Referencias Schneider"=w901, "Referencias Delta"=w899, "Referencias ABB"=w898, "Referencias LS-Electric"=w877) -> (w900:T30)  [unwired: 1 in]
              n625 = Bundle("I/O PowerFlex"=w876, "I/O Schneider"=w896, "I/O Delta"=w895, "I/O ABB"=w894, "I/O LS-Electric"=w874) -> (w897:T31)  [unwired: 1 in]
              n626 = Bundle("Motor PowerFlex"=w873, "Motor LS-Electric"=w871) -> (w893:T32)  [unwired: 1 in]
              n627 = Bundle("Modbus PowerFlex"=w870, "Modbus LS-Electric"=w868) -> (w892:T33)  [unwired: 1 in]
              n628 = case shown="0, Default" w885 {
                tunnel: [12 8 10] -> w866
                frame 0, Default {
                  # "Control de VFD."
                }
                frame 1, 3 {
                  # "Configurar motor."
                }
                frame 2 {
                  # "Configurar Modbus."
                }
              }
              n629 = call "Revisión_VFD.vi"("Fabricante"=w867, "Modbus"=w892, "Iteración (In)"=w890, "Motor"=w893, "I/O"=w897, "Referencias"=w900, "Instancia Modbus"=w902) -> ("Error Modbus"=w891:errorcluster, "Iteración (Out)"=w864:u32, "Coincidentes"=w863:bool[])  [unwired: 2 in]
              n630 = local write "Error Modbus"(w891) -> ()
              n631 = local write "Iteración"(w864) -> ()
            }
            n632 = local write "Download"(w859) -> ()
            n633 = local write "Paso"(w860) -> ()
          }
        }
        n634 = Index Array(array=w806, index=1) -> (element=w803:bool)
        n635 = Replace Array Subset(array=w805, new element=w803, index=1) -> (w804:bool[])
      }
      frame 8 {
        # "Descargar parámetros a variador (Características de motor)."
        n636 = local read "Fabricante"() -> (w907:u32)
        n637 = case shown="0, Default" w907 {
          selector: w907 -> [w911 w948]
          frame 0, Default {
            # "Allen Bradley."
            n638 = for {
              N: 10 -> [_]
              tunnel: w911 -> [w916]
              tunnel: [9] -> w910
              tunnel: [FALSE] -> w909
              # "10 intentos/iteraciones."
              n639 = local read "Iteración"() -> (w929:u32)
              n640 = local read "Instancia Modbus"() -> (w945:refnum<class "Modbus Master.lvclass">)
              n641 = local read "Referencias PowerFlex"() -> (w917:T2)
              n642 = local read "Referencias Schneider"() -> (w944:T2)
              n643 = local read "Referencias Delta"() -> (w941:T2)
              n644 = local read "Referencias ABB"() -> (w940:T2)
              n645 = local read "Referencias LS-Electric"() -> (w942:T2)
              n646 = local read "I/O PowerFlex"() -> (w925:T3)
              n647 = local read "I/O Schneider"() -> (w938:T6)
              n648 = local read "I/O Delta"() -> (w937:T7)
              n649 = local read "I/O ABB"() -> (w936:T8)
              n650 = local read "I/O LS-Electric"() -> (w935:T9)
              n651 = local read "Motor PowerFlex"() -> (w922:T4)
              n652 = local read "Motor LS-Electric"() -> (w933:T10)
              n653 = local read "Modbus PowerFlex"() -> (w919:T5)
              n654 = local read "Modbus LS-Electric"() -> (w931:T11)
              n655 = Bundle By Name(cluster=w917, "Descargar"=FALSE) -> (w927:T2)
              n656 = Bundle By Name(cluster=w925, "Descargar"=FALSE) -> (w924:T3)
              n657 = Bundle By Name(cluster=w922, "Descargar"=TRUE) -> (w921:T4)
              n658 = Bundle By Name(cluster=w919, "Descargar"=FALSE) -> (w918:T5)
              n659 = Bundle("Referencias PowerFlex"=w927, "Referencias Schneider"=w944, "Referencias Delta"=w941, "Referencias ABB"=w940, "Referencias LS-Electric"=w942) -> (w943:T30)  [unwired: 1 in]
              n660 = Bundle("I/O PowerFlex"=w924, "I/O Schneider"=w938, "I/O Delta"=w937, "I/O ABB"=w936, "I/O LS-Electric"=w935) -> (w939:T31)  [unwired: 1 in]
              n661 = Bundle("Motor PowerFlex"=w921, "Motor LS-Electric"=w933) -> (w934:T32)  [unwired: 1 in]
              n662 = Bundle("Modbus PowerFlex"=w918, "Modbus LS-Electric"=w931) -> (w932:T33)  [unwired: 1 in]
              n663 = call "Descarga_VFD.vi"("Fabricante"=w916, "Modbus"=w932, "Iteraciones (In)"=w929, "Motor"=w934, "I/O"=w939, "Referencias"=w943, "Instancia Modbus"=w945) -> ("Error Modbus"=w930:errorcluster, "Iteraciones (Out)"=w913:u32)  [unwired: 3 in]
              n664 = local write "Error Modbus"(w930) -> ()
              n665 = local write "Iteración"(w913) -> ()
            }
            n666 = local write "Download"(w909) -> ()
            n667 = local write "Paso"(w910) -> ()
          }
          frame 4 {
            # "LS-Electric."
            n668 = for {
              N: 10 -> [_]
              tunnel: w948 -> [w953]
              tunnel: [9] -> w947
              tunnel: [FALSE] -> w946
              # "10 intentos/iteraciones."
              n669 = local read "Iteración"() -> (w970:u32)
              n670 = local read "Instancia Modbus"() -> (w982:refnum<class "Modbus Master.lvclass">)
              n671 = local read "Referencias PowerFlex"() -> (w965:T2)
              n672 = local read "Referencias Schneider"() -> (w981:T2)
              n673 = local read "Referencias Delta"() -> (w979:T2)
              n674 = local read "Referencias ABB"() -> (w978:T2)
              n675 = local read "Referencias LS-Electric"() -> (w964:T2)
              n676 = local read "I/O PowerFlex"() -> (w962:T3)
              n677 = local read "I/O Schneider"() -> (w976:T6)
              n678 = local read "I/O Delta"() -> (w975:T7)
              n679 = local read "I/O ABB"() -> (w974:T8)
              n680 = local read "I/O LS-Electric"() -> (w961:T9)
              n681 = local read "Motor PowerFlex"() -> (w959:T4)
              n682 = local read "Motor LS-Electric"() -> (w958:T10)
              n683 = local read "Modbus PowerFlex"() -> (w956:T5)
              n684 = local read "Modbus LS-Electric"() -> (w955:T11)
              n685 = Bundle By Name(cluster=w964, "Descargar"=FALSE) -> (w963:T2)
              n686 = Bundle By Name(cluster=w961, "Descargar"=FALSE) -> (w960:T9)
              n687 = Bundle By Name(cluster=w958, "Descargar"=TRUE) -> (w957:T10)
              n688 = Bundle By Name(cluster=w955, "Descargar"=FALSE) -> (w954:T11)
              n689 = Bundle("Referencias PowerFlex"=w965, "Referencias Schneider"=w981, "Referencias Delta"=w979, "Referencias ABB"=w978, "Referencias LS-Electric"=w963) -> (w980:T30)  [unwired: 1 in]
              n690 = Bundle("I/O PowerFlex"=w962, "I/O Schneider"=w976, "I/O Delta"=w975, "I/O ABB"=w974, "I/O LS-Electric"=w960) -> (w977:T31)  [unwired: 1 in]
              n691 = Bundle("Motor PowerFlex"=w959, "Motor LS-Electric"=w957) -> (w973:T32)  [unwired: 1 in]
              n692 = Bundle("Modbus PowerFlex"=w956, "Modbus LS-Electric"=w954) -> (w972:T33)  [unwired: 1 in]
              n693 = call "Descarga_VFD.vi"("Fabricante"=w953, "Modbus"=w972, "Iteraciones (In)"=w970, "Motor"=w973, "I/O"=w977, "Referencias"=w980, "Instancia Modbus"=w982) -> ("Error Modbus"=w971:errorcluster, "Iteraciones (Out)"=w950:u32)  [unwired: 3 in]
              n694 = local write "Error Modbus"(w971) -> ()
              n695 = local write "Iteración"(w950) -> ()
            }
            n696 = local write "Download"(w946) -> ()
            n697 = local write "Paso"(w947) -> ()
          }
        }
        n698 = local read "Coincidentes"() -> (w906:bool[])
      }
      frame 9 {
        # "Revisar parámetros de variador (Características de motor)."
        n699 = local read "Fabricante"() -> (w989:u32)
        n700 = case shown="4" w989 {
          selector: w989 -> [w994 w1039]
          tunnel: [w991 w1036] -> w987
          frame 0, Default {
            # "Allen Bradley."
            n701 = for {
              N: 10 -> [_]
              tunnel: w994 -> [w1000]
              tunnel: [w999] -> w993
              tunnel: [FALSE] -> w992
              tunnel: [w996] -> w991
              # "10 intentos/iteraciones."
              n702 = local read "Iteración"() -> (w1017:u32)
              n703 = local read "Instancia Modbus"() -> (w1033:refnum<class "Modbus Master.lvclass">)
              n704 = local read "Referencias PowerFlex"() -> (w1001:T2)
              n705 = local read "Referencias Schneider"() -> (w1032:T2)
              n706 = local read "Referencias Delta"() -> (w1029:T2)
              n707 = local read "Referencias ABB"() -> (w1028:T2)
              n708 = local read "Referencias LS-Electric"() -> (w1030:T2)
              n709 = local read "I/O PowerFlex"() -> (w1013:T3)
              n710 = local read "I/O Schneider"() -> (w1026:T6)
              n711 = local read "I/O Delta"() -> (w1025:T7)
              n712 = local read "I/O ABB"() -> (w1024:T8)
              n713 = local read "I/O LS-Electric"() -> (w1023:T9)
              n714 = local read "Motor PowerFlex"() -> (w1010:T4)
              n715 = local read "Motor LS-Electric"() -> (w1021:T10)
              n716 = local read "Modbus PowerFlex"() -> (w1007:T5)
              n717 = local read "Modbus LS-Electric"() -> (w1019:T11)
              n718 = local read "Modbus PowerFlex"() -> (w1002:T5)
              n719 = Bundle By Name(cluster=w1001, "Descargar"=FALSE) -> (w1015:T2)
              n720 = Bundle By Name(cluster=w1013, "Descargar"=FALSE) -> (w1012:T3)
              n721 = Bundle By Name(cluster=w1010, "Descargar"=TRUE) -> (w1009:T4)
              n722 = Bundle By Name(cluster=w1007, "Descargar"=FALSE) -> (w1006:T5)
              n723 = Unbundle By Name(w1002) -> ("Descargar"=w1003:bool)
              n724 = Build Array(w1003) -> (w1004:bool[])
              n725 = Boolean Array To Number(Boolean array=w1004) -> (number=w1005:u32)
              n726 = Bundle("Referencias PowerFlex"=w1015, "Referencias Schneider"=w1032, "Referencias Delta"=w1029, "Referencias ABB"=w1028, "Referencias LS-Electric"=w1030) -> (w1031:T30)  [unwired: 1 in]
              n727 = Bundle("I/O PowerFlex"=w1012, "I/O Schneider"=w1026, "I/O Delta"=w1025, "I/O ABB"=w1024, "I/O LS-Electric"=w1023) -> (w1027:T31)  [unwired: 1 in]
              n728 = Bundle("Motor PowerFlex"=w1009, "Motor LS-Electric"=w1021) -> (w1022:T32)  [unwired: 1 in]
              n729 = Bundle("Modbus PowerFlex"=w1006, "Modbus LS-Electric"=w1019) -> (w1020:T33)  [unwired: 1 in]
              n730 = case shown="0, Default" w1005 {
                tunnel: [12 10] -> w999
                frame 0, Default {
                  # "Control de VFD."
                }
                frame 1 {
                  # "Configurar Modbus."
                }
              }
              n731 = call "Revisión_VFD.vi"("Fabricante"=w1000, "Modbus"=w1020, "Iteración (In)"=w1017, "Motor"=w1022, "I/O"=w1027, "Referencias"=w1031, "Instancia Modbus"=w1033) -> ("Error Modbus"=w1018:errorcluster, "Iteración (Out)"=w997:u32, "Coincidentes"=w996:bool[])  [unwired: 2 in]
              n732 = local write "Error Modbus"(w1018) -> ()
              n733 = local write "Iteración"(w997) -> ()
            }
            n734 = local write "Download"(w992) -> ()
            n735 = local write "Paso"(w993) -> ()
          }
          frame 4 {
            # "LS-Electric."
            n736 = for {
              N: 10 -> [_]
              tunnel: w1039 -> [w1045]
              tunnel: [w1044] -> w1038
              tunnel: [FALSE] -> w1037
              tunnel: [w1041] -> w1036
              # "10 intentos/iteraciones."
              n737 = local read "Iteración"() -> (w1066:u32)
              n738 = local read "Instancia Modbus"() -> (w1078:refnum<class "Modbus Master.lvclass">)
              n739 = local read "Referencias PowerFlex"() -> (w1057:T2)
              n740 = local read "Referencias Schneider"() -> (w1077:T2)
              n741 = local read "Referencias Delta"() -> (w1075:T2)
              n742 = local read "Referencias ABB"() -> (w1074:T2)
              n743 = local read "Referencias LS-Electric"() -> (w1056:T2)
              n744 = local read "I/O PowerFlex"() -> (w1054:T3)
              n745 = local read "I/O Schneider"() -> (w1072:T6)
              n746 = local read "I/O Delta"() -> (w1071:T7)
              n747 = local read "I/O ABB"() -> (w1070:T8)
              n748 = local read "I/O LS-Electric"() -> (w1053:T9)
              n749 = local read "Motor PowerFlex"() -> (w1051:T4)
              n750 = local read "Motor LS-Electric"() -> (w1050:T10)
              n751 = local read "Modbus PowerFlex"() -> (w1048:T5)
              n752 = local read "Modbus LS-Electric"() -> (w1047:T11)
              n753 = local read "Modbus LS-Electric"() -> (w1058:T11)
              n754 = Bundle By Name(cluster=w1056, "Descargar"=FALSE) -> (w1055:T2)
              n755 = Bundle By Name(cluster=w1053, "Descargar"=FALSE) -> (w1052:T9)
              n756 = Bundle By Name(cluster=w1050, "Descargar"=TRUE) -> (w1049:T10)
              n757 = Bundle By Name(cluster=w1047, "Descargar"=FALSE) -> (w1046:T11)
              n758 = Unbundle By Name(w1058) -> ("Descargar"=w1059:bool)
              n759 = Build Array(w1059) -> (w1060:bool[])
              n760 = Boolean Array To Number(Boolean array=w1060) -> (number=w1061:u32)
              n761 = Bundle("Referencias PowerFlex"=w1057, "Referencias Schneider"=w1077, "Referencias Delta"=w1075, "Referencias ABB"=w1074, "Referencias LS-Electric"=w1055) -> (w1076:T30)  [unwired: 1 in]
              n762 = Bundle("I/O PowerFlex"=w1054, "I/O Schneider"=w1072, "I/O Delta"=w1071, "I/O ABB"=w1070, "I/O LS-Electric"=w1052) -> (w1073:T31)  [unwired: 1 in]
              n763 = Bundle("Motor PowerFlex"=w1051, "Motor LS-Electric"=w1049) -> (w1069:T32)  [unwired: 1 in]
              n764 = Bundle("Modbus PowerFlex"=w1048, "Modbus LS-Electric"=w1046) -> (w1068:T33)  [unwired: 1 in]
              n765 = case shown="0, Default" w1061 {
                tunnel: [12 10] -> w1044
                frame 0, Default {
                  # "Control de VFD."
                }
                frame 1 {
                  # "Configurar Modbus."
                }
              }
              n766 = call "Revisión_VFD.vi"("Fabricante"=w1045, "Modbus"=w1068, "Iteración (In)"=w1066, "Motor"=w1069, "I/O"=w1073, "Referencias"=w1076, "Instancia Modbus"=w1078) -> ("Error Modbus"=w1067:errorcluster, "Iteración (Out)"=w1042:u32, "Coincidentes"=w1041:bool[])  [unwired: 2 in]
              n767 = local write "Error Modbus"(w1067) -> ()
              n768 = local write "Iteración"(w1042) -> ()
            }
            n769 = local write "Download"(w1037) -> ()
            n770 = local write "Paso"(w1038) -> ()
          }
        }
        n771 = Index Array(array=w987, index=2) -> (element=w984:bool)
        n772 = Replace Array Subset(array=w985, new element=w984, index=2) -> (w983:bool[])
      }
      frame 10 {
        # "Descargar parámetros a variador (Modbus)."
        n773 = local read "Fabricante"() -> (w1082:u32)
        n774 = case shown="0, Default" w1082 {
          selector: w1082 -> [w1086 w1123]
          frame 0, Default {
            # "Allen Bradley."
            n775 = for {
              N: 10 -> [_]
              tunnel: w1086 -> [w1091]
              tunnel: [11] -> w1085
              tunnel: [FALSE] -> w1084
              # "10 intentos/iteraciones."
              n776 = local read "Iteración"() -> (w1104:u32)
              n777 = local read "Instancia Modbus"() -> (w1120:refnum<class "Modbus Master.lvclass">)
              n778 = local read "Referencias PowerFlex"() -> (w1092:T2)
              n779 = local read "Referencias Schneider"() -> (w1119:T2)
              n780 = local read "Referencias Delta"() -> (w1116:T2)
              n781 = local read "Referencias ABB"() -> (w1115:T2)
              n782 = local read "Referencias LS-Electric"() -> (w1117:T2)
              n783 = local read "I/O PowerFlex"() -> (w1100:T3)
              n784 = local read "I/O Schneider"() -> (w1113:T6)
              n785 = local read "I/O Delta"() -> (w1112:T7)
              n786 = local read "I/O ABB"() -> (w1111:T8)
              n787 = local read "I/O LS-Electric"() -> (w1110:T9)
              n788 = local read "Motor PowerFlex"() -> (w1097:T4)
              n789 = local read "Motor LS-Electric"() -> (w1108:T10)
              n790 = local read "Modbus PowerFlex"() -> (w1094:T5)
              n791 = local read "Modbus LS-Electric"() -> (w1106:T11)
              n792 = Bundle By Name(cluster=w1092, "Descargar"=FALSE) -> (w1102:T2)
              n793 = Bundle By Name(cluster=w1100, "Descargar"=FALSE) -> (w1099:T3)
              n794 = Bundle By Name(cluster=w1097, "Descargar"=FALSE) -> (w1096:T4)
              n795 = Bundle By Name(cluster=w1094, "Descargar"=TRUE) -> (w1093:T5)
              n796 = Bundle("Referencias PowerFlex"=w1102, "Referencias Schneider"=w1119, "Referencias Delta"=w1116, "Referencias ABB"=w1115, "Referencias LS-Electric"=w1117) -> (w1118:T30)  [unwired: 1 in]
              n797 = Bundle("I/O PowerFlex"=w1099, "I/O Schneider"=w1113, "I/O Delta"=w1112, "I/O ABB"=w1111, "I/O LS-Electric"=w1110) -> (w1114:T31)  [unwired: 1 in]
              n798 = Bundle("Motor PowerFlex"=w1096, "Motor LS-Electric"=w1108) -> (w1109:T32)  [unwired: 1 in]
              n799 = Bundle("Modbus PowerFlex"=w1093, "Modbus LS-Electric"=w1106) -> (w1107:T33)  [unwired: 1 in]
              n800 = call "Descarga_VFD.vi"("Fabricante"=w1091, "Modbus"=w1107, "Iteraciones (In)"=w1104, "Motor"=w1109, "I/O"=w1114, "Referencias"=w1118, "Instancia Modbus"=w1120) -> ("Error Modbus"=w1105:errorcluster, "Iteraciones (Out)"=w1088:u32)  [unwired: 3 in]
              n801 = local write "Error Modbus"(w1105) -> ()
              n802 = local write "Iteración"(w1088) -> ()
            }
            n803 = local write "Download"(w1084) -> ()
            n804 = local write "Paso"(w1085) -> ()
          }
          frame 4 {
            # "LS-Electric."
            n805 = for {
              N: 10 -> [_]
              tunnel: w1123 -> [w1128]
              tunnel: [11] -> w1122
              tunnel: [FALSE] -> w1121
              # "10 intentos/iteraciones."
              n806 = local read "Iteración"() -> (w1145:u32)
              n807 = local read "Instancia Modbus"() -> (w1157:refnum<class "Modbus Master.lvclass">)
              n808 = local read "Referencias PowerFlex"() -> (w1140:T2)
              n809 = local read "Referencias Schneider"() -> (w1156:T2)
              n810 = local read "Referencias Delta"() -> (w1154:T2)
              n811 = local read "Referencias ABB"() -> (w1153:T2)
              n812 = local read "Referencias LS-Electric"() -> (w1139:T2)
              n813 = local read "I/O PowerFlex"() -> (w1137:T3)
              n814 = local read "I/O Schneider"() -> (w1151:T6)
              n815 = local read "I/O Delta"() -> (w1150:T7)
              n816 = local read "I/O ABB"() -> (w1149:T8)
              n817 = local read "I/O LS-Electric"() -> (w1136:T9)
              n818 = local read "Motor PowerFlex"() -> (w1134:T4)
              n819 = local read "Motor LS-Electric"() -> (w1133:T10)
              n820 = local read "Modbus PowerFlex"() -> (w1131:T5)
              n821 = local read "Modbus LS-Electric"() -> (w1130:T11)
              n822 = Bundle By Name(cluster=w1139, "Descargar"=FALSE) -> (w1138:T2)
              n823 = Bundle By Name(cluster=w1136, "Descargar"=FALSE) -> (w1135:T9)
              n824 = Bundle By Name(cluster=w1133, "Descargar"=FALSE) -> (w1132:T10)
              n825 = Bundle By Name(cluster=w1130, "Descargar"=TRUE) -> (w1129:T11)
              n826 = Bundle("Referencias PowerFlex"=w1140, "Referencias Schneider"=w1156, "Referencias Delta"=w1154, "Referencias ABB"=w1153, "Referencias LS-Electric"=w1138) -> (w1155:T30)  [unwired: 1 in]
              n827 = Bundle("I/O PowerFlex"=w1137, "I/O Schneider"=w1151, "I/O Delta"=w1150, "I/O ABB"=w1149, "I/O LS-Electric"=w1135) -> (w1152:T31)  [unwired: 1 in]
              n828 = Bundle("Motor PowerFlex"=w1134, "Motor LS-Electric"=w1132) -> (w1148:T32)  [unwired: 1 in]
              n829 = Bundle("Modbus PowerFlex"=w1131, "Modbus LS-Electric"=w1129) -> (w1147:T33)  [unwired: 1 in]
              n830 = call "Descarga_VFD.vi"("Fabricante"=w1128, "Modbus"=w1147, "Iteraciones (In)"=w1145, "Motor"=w1148, "I/O"=w1152, "Referencias"=w1155, "Instancia Modbus"=w1157) -> ("Error Modbus"=w1146:errorcluster, "Iteraciones (Out)"=w1125:u32)  [unwired: 3 in]
              n831 = local write "Error Modbus"(w1146) -> ()
              n832 = local write "Iteración"(w1125) -> ()
            }
            n833 = local write "Download"(w1121) -> ()
            n834 = local write "Paso"(w1122) -> ()
          }
        }
        n835 = local read "Coincidentes"() -> (w1081:bool[])
      }
      frame 11 {
        # "Revisar parámetros de variador (Modbus)."
        n836 = local read "Fabricante"() -> (w1164:u32)
        n837 = case shown="0, Default" w1164 {
          selector: w1164 -> [w1169 w1208]
          tunnel: [w1166 w1205] -> w1162
          frame 0, Default {
            # "Allen Bradley."
            n838 = for {
              N: 10 -> [_]
              tunnel: w1169 -> [w1175]
              tunnel: [12] -> w1168
              tunnel: [FALSE] -> w1167
              tunnel: [w1171] -> w1166
              # "10 intentos/iteraciones."
              n839 = local read "Iteración"() -> (w1188:u32)
              n840 = local read "Instancia Modbus"() -> (w1204:refnum<class "Modbus Master.lvclass">)
              n841 = local read "Referencias PowerFlex"() -> (w1176:T2)
              n842 = local read "Referencias Schneider"() -> (w1203:T2)
              n843 = local read "Referencias Delta"() -> (w1200:T2)
              n844 = local read "Referencias ABB"() -> (w1199:T2)
              n845 = local read "Referencias LS-Electric"() -> (w1201:T2)
              n846 = local read "I/O PowerFlex"() -> (w1184:T3)
              n847 = local read "I/O Schneider"() -> (w1197:T6)
              n848 = local read "I/O Delta"() -> (w1196:T7)
              n849 = local read "I/O ABB"() -> (w1195:T8)
              n850 = local read "I/O LS-Electric"() -> (w1194:T9)
              n851 = local read "Motor PowerFlex"() -> (w1181:T4)
              n852 = local read "Motor LS-Electric"() -> (w1192:T10)
              n853 = local read "Modbus PowerFlex"() -> (w1178:T5)
              n854 = local read "Modbus LS-Electric"() -> (w1190:T11)
              n855 = Bundle By Name(cluster=w1176, "Descargar"=FALSE) -> (w1186:T2)
              n856 = Bundle By Name(cluster=w1184, "Descargar"=FALSE) -> (w1183:T3)
              n857 = Bundle By Name(cluster=w1181, "Descargar"=FALSE) -> (w1180:T4)
              n858 = Bundle By Name(cluster=w1178, "Descargar"=TRUE) -> (w1177:T5)
              n859 = Bundle("Referencias PowerFlex"=w1186, "Referencias Schneider"=w1203, "Referencias Delta"=w1200, "Referencias ABB"=w1199, "Referencias LS-Electric"=w1201) -> (w1202:T30)  [unwired: 1 in]
              n860 = Bundle("I/O PowerFlex"=w1183, "I/O Schneider"=w1197, "I/O Delta"=w1196, "I/O ABB"=w1195, "I/O LS-Electric"=w1194) -> (w1198:T31)  [unwired: 1 in]
              n861 = Bundle("Motor PowerFlex"=w1180, "Motor LS-Electric"=w1192) -> (w1193:T32)  [unwired: 1 in]
              n862 = Bundle("Modbus PowerFlex"=w1177, "Modbus LS-Electric"=w1190) -> (w1191:T33)  [unwired: 1 in]
              n863 = call "Revisión_VFD.vi"("Fabricante"=w1175, "Modbus"=w1191, "Iteración (In)"=w1188, "Motor"=w1193, "I/O"=w1198, "Referencias"=w1202, "Instancia Modbus"=w1204) -> ("Error Modbus"=w1189:errorcluster, "Iteración (Out)"=w1172:u32, "Coincidentes"=w1171:bool[])  [unwired: 2 in]
              n864 = local write "Error Modbus"(w1189) -> ()
              n865 = local write "Iteración"(w1172) -> ()
            }
            n866 = local write "Download"(w1167) -> ()
            n867 = local write "Paso"(w1168) -> ()
          }
          frame 4 {
            # "LS-Electric."
            n868 = for {
              N: 10 -> [_]
              tunnel: w1208 -> [w1214]
              tunnel: [12] -> w1207
              tunnel: [FALSE] -> w1206
              tunnel: [w1210] -> w1205
              # "10 intentos/iteraciones."
              n869 = local read "Iteración"() -> (w1231:u32)
              n870 = local read "Instancia Modbus"() -> (w1243:refnum<class "Modbus Master.lvclass">)
              n871 = local read "Referencias PowerFlex"() -> (w1226:T2)
              n872 = local read "Referencias Schneider"() -> (w1242:T2)
              n873 = local read "Referencias Delta"() -> (w1240:T2)
              n874 = local read "Referencias ABB"() -> (w1239:T2)
              n875 = local read "Referencias LS-Electric"() -> (w1225:T2)
              n876 = local read "I/O PowerFlex"() -> (w1223:T3)
              n877 = local read "I/O Schneider"() -> (w1237:T6)
              n878 = local read "I/O Delta"() -> (w1236:T7)
              n879 = local read "I/O ABB"() -> (w1235:T8)
              n880 = local read "I/O LS-Electric"() -> (w1222:T9)
              n881 = local read "Motor PowerFlex"() -> (w1220:T4)
              n882 = local read "Motor LS-Electric"() -> (w1219:T10)
              n883 = local read "Modbus PowerFlex"() -> (w1217:T5)
              n884 = local read "Modbus LS-Electric"() -> (w1216:T11)
              n885 = Bundle By Name(cluster=w1225, "Descargar"=FALSE) -> (w1224:T2)
              n886 = Bundle By Name(cluster=w1222, "Descargar"=FALSE) -> (w1221:T9)
              n887 = Bundle By Name(cluster=w1219, "Descargar"=FALSE) -> (w1218:T10)
              n888 = Bundle By Name(cluster=w1216, "Descargar"=TRUE) -> (w1215:T11)
              n889 = Bundle("Referencias PowerFlex"=w1226, "Referencias Schneider"=w1242, "Referencias Delta"=w1240, "Referencias ABB"=w1239, "Referencias LS-Electric"=w1224) -> (w1241:T30)  [unwired: 1 in]
              n890 = Bundle("I/O PowerFlex"=w1223, "I/O Schneider"=w1237, "I/O Delta"=w1236, "I/O ABB"=w1235, "I/O LS-Electric"=w1221) -> (w1238:T31)  [unwired: 1 in]
              n891 = Bundle("Motor PowerFlex"=w1220, "Motor LS-Electric"=w1218) -> (w1234:T32)  [unwired: 1 in]
              n892 = Bundle("Modbus PowerFlex"=w1217, "Modbus LS-Electric"=w1215) -> (w1233:T33)  [unwired: 1 in]
              n893 = call "Revisión_VFD.vi"("Fabricante"=w1214, "Modbus"=w1233, "Iteración (In)"=w1231, "Motor"=w1234, "I/O"=w1238, "Referencias"=w1241, "Instancia Modbus"=w1243) -> ("Error Modbus"=w1232:errorcluster, "Iteración (Out)"=w1211:u32, "Coincidentes"=w1210:bool[])  [unwired: 2 in]
              n894 = local write "Error Modbus"(w1232) -> ()
              n895 = local write "Iteración"(w1211) -> ()
            }
            n896 = local write "Download"(w1206) -> ()
            n897 = local write "Paso"(w1207) -> ()
          }
        }
        n898 = Index Array(array=w1162, index=3) -> (element=w1159:bool)
        n899 = Replace Array Subset(array=w1160, new element=w1159, index=3) -> (w1158:bool[])
      }
      frame 12 {
        # "Control y monitoreo de variador: Se ha hecho la configuración."
        n900 = local read "Frecuencia"() -> (w1253:dbl)
        n901 = local read "Instancia Modbus"() -> (w1262:refnum<class "Modbus Master.lvclass">)
        n902 = local read "Fabricante"() -> (w1261:u32)
        n903 = local read "Run"() -> (w1256:bool)
        n904 = local read "Sentido"() -> (w1255:bool)
        n905 = local read "Reset"() -> (w1254:bool)
        n906 = local read "Salidas digitales"() -> (w1252:cluster{"Salida":bool, "Etiqueta":string}[])
        n907 = local read "Entradas digitales"() -> (w1257:cluster{"Estado":bool, "Etiqueta":string}[])
        n908 = Not Equal?(x=w1247, y=w1246) -> (x != y?=w1245:bool)
        n909 = for {
          tunnel: w1252 -> [w1307] mode=indexing
          tunnel: [w1306] -> w1251 mode=indexing
          n910 = Unbundle By Name(w1307) -> ("Salida"=w1306:bool)
        }
        n911 = case shown="True" w1248 {
          tunnel: [w1265 w1272] -> w1250
          tunnel: [w1264 w1269] -> w1244
          frame False {
            # "Permanecer en este paso."
            n912 = local read "Escanear"() -> (w1268:bool)
            n913 = local read "Coincidentes"() -> (w1264:bool[])
            n914 = Select(t=1, s=w1268, f=12) -> (s? t:f=w1265:i32)
          }
          frame True {
            # "Descargar parámetros."
            n915 = local read "Fabricante"() -> (w1273:u32)
            n916 = case shown="4" w1273 {
              tunnel: [w1274 w1290] -> w1272
              frame 0, Default {
                # "Allen Bradley."
                n917 = local read "Referencias PowerFlex"() -> (w1284:T2)
                n918 = local read "I/O PowerFlex"() -> (w1283:T3)
                n919 = local read "Motor PowerFlex"() -> (w1282:T4)
                n920 = local read "Modbus PowerFlex"() -> (w1281:T5)
                n921 = Unbundle By Name(w1284) -> ("Descargar"=w1280:bool)
                n922 = Unbundle By Name(w1283) -> ("Descargar"=w1279:bool)
                n923 = Unbundle By Name(w1282) -> ("Descargar"=w1278:bool)
                n924 = Unbundle By Name(w1281) -> ("Descargar"=w1277:bool)
                n925 = Build Array(w1280, w1279, w1278, w1277) -> (w1276:bool[])
                n926 = Boolean Array To Number(Boolean array=w1276) -> (number=w1275:u32)
                n927 = case shown="0, Default" w1275 {
                  tunnel: [12 4 5 6 7] -> w1274
                  frame 0, Default {
                    # "Nada."
                  }
                  frame 1, 3, 5, 7, 9, 11, 13, 15 {
                    # "Configurar referencias."
                  }
                  frame 2, 6, 10, 14 {
                    # "Configurar entradas y salidas."
                  }
                  frame 4, 12 {
                    # "Configurar motor."
                  }
                  frame 8 {
                    # "Configurar Modbus."
                  }
                }
              }
              frame 4 {
                # "LS-Electric."
                n928 = local read "Referencias LS-Electric"() -> (w1300:T2)
                n929 = local read "I/O LS-Electric"() -> (w1299:T9)
                n930 = local read "Motor LS-Electric"() -> (w1298:T10)
                n931 = local read "Modbus LS-Electric"() -> (w1297:T11)
                n932 = Unbundle By Name(w1300) -> ("Descargar"=w1296:bool)
                n933 = Unbundle By Name(w1299) -> ("Descargar"=w1295:bool)
                n934 = Unbundle By Name(w1298) -> ("Descargar"=w1294:bool)
                n935 = Unbundle By Name(w1297) -> ("Descargar"=w1293:bool)
                n936 = Build Array(w1296, w1295, w1294, w1293) -> (w1292:bool[])
                n937 = Boolean Array To Number(Boolean array=w1292) -> (number=w1291:u32)
                n938 = case shown="0, Default" w1291 {
                  tunnel: [12 4 5 6 7] -> w1290
                  frame 0, Default {
                    # "Nada."
                  }
                  frame 1, 3, 5, 7, 9, 11, 13, 15 {
                    # "Configurar referencias."
                  }
                  frame 2, 6, 10, 14 {
                    # "Configurar entradas y salidas."
                  }
                  frame 4, 12 {
                    # "Configurar motor."
                  }
                  frame 8 {
                    # "Configurar Modbus."
                  }
                }
              }
            }
            n939 = Initialize Array(FALSE, 4 ("dimension size")) -> (w1269:bool[])
          }
        }
        n940 = case shown="True" w1245 {
          frame False {
            # "Nada."
          }
          frame True {
            # "Reiniciar variable."
            n941 = local write "Escanear"(FALSE ("Download")) -> ()
          }
        }
        n942 = call "Comunicación_VFD.vi"("Salidas digitales"=w1251, "Reset"=w1254, "Frecuencia"=w1253, "Sentido"=w1255, "Run"=w1256, "Fabricante"=w1261, "Instancia Modbus"=w1262) -> ("Error Modbus"=w1260:errorcluster, "Entradas digitales"=w1259:bool[])  [unwired: 3 in]
        n943 = for {
          tunnel: w1259 -> [w1311] mode=indexing
          tunnel: w1257 -> [w1312] mode=indexing
          tunnel: [w1309] -> w1258 mode=indexing
          tunnel: w1257 -> [w1308] mode=indexing
          n944 = Unbundle By Name(w1312) -> ("Etiqueta"=w1310:string)
          n945 = Bundle By Name(cluster=w1308, "Estado"=w1311, "Etiqueta"=w1310) -> (w1309:cluster{"Estado":bool, "Etiqueta":string})
        }
        n946 = local write "Error Modbus"(w1260) -> ()
        n947 = local write "Entradas digitales"(w1258) -> ()
        n948 = local write "Iteración"(u32 0 ("Paso")) -> ()
        n949 = local write "Paso"(w1250) -> ()
      }
    }
    n950 = local write "Coincidentes"(w408) -> ()
    n951 = local read "Salir"() -> (w415:bool)
  }
  n952 = while {
    tunnel: [w1318] -> _
    tunnel: [w1317] -> _
    tunnel: [w1313] -> w3
    stop <- w1313 stop-if-true
    # "Respecto a los colores del anillo de progreso:\nPosición [1] del arreglo: Color progreso.\nPosición [2] del arreglo: Color fondo."
    # "Mensajes e indicadores para el usuario."
    n953 = local read "Paso"() -> (w1328:u32)
    n954 = case shown="4..11" w1328 {
      tunnel: [w1333 w1342 w1352 w1360 w1377 w1475] -> w1320
      tunnel: [w1332 w1341 w1351 w1359 w1376 w1474] -> w1316
      tunnel: [_ _ _ _ _ w1467] -> _
      tunnel: [_ _ _ _ _ w1466] -> _
      tunnel: [_ _ _ _ _ w1465] -> _
      frame 0, Default {
        w1331 = 0.0
        # "Esperando a escaneo."
        n955 = Increment(x=w1331) -> (x+1=w1334:dbl)
        n956 = local write "Estatus (color)"(u32 11908789) -> ()
        n957 = local write "Avance (número)"(w1331) -> ()
        n958 = local write "Avance (anillo)"(w1331) -> ()
        n959 = Bundle(cluster=cluster{dbl, i32} {0.0, 16759552}, w1331) -> (w1332:cluster{dbl, i32})  [unwired: 1 in]
        n960 = local write "Mensaje"("Seleccione fabricante.\nY después pulse el botón\npara comenzar la búsqueda.") -> ()
        n961 = Bundle(cluster=cluster{dbl, i32} {0.0, 9868950}, w1334) -> (w1333:cluster{dbl, i32})  [unwired: 1 in]
      }
      frame 1 {
        # "Buscando variador."
        n962 = global read "Temporales.vi" "Estatus"() -> (w1347:string)
        n963 = global read "Temporales.vi" "Avance"() -> (w1344:dbl)
        n964 = call "Alarma parpadeante (elemento).vi"("Color ON2"=u32 16744448, "Color ON1"=u32 16744512, "Color OFF"=u32 11908789) -> ("Color (alarma)"=w1337:u32)  [unwired: 8 in]
        n965 = Increment(x=w1344) -> (x+1=w1343:dbl)
        n966 = local write "Mensaje"(w1347) -> ()
        n967 = local write "Avance (número)"(w1344) -> ()
        n968 = local write "Avance (anillo)"(w1344) -> ()
        n969 = local write "Estatus (color)"(w1337) -> ()
        n970 = Bundle(cluster=cluster{dbl, i32} {0.0, 16759552}, w1344) -> (w1341:cluster{dbl, i32})  [unwired: 1 in]
        n971 = Bundle(cluster=cluster{dbl, i32} {0.0, 9868950}, w1343) -> (w1342:cluster{dbl, i32})  [unwired: 1 in]
      }
      frame 2 {
        w1350 = 100.0
        # "Variador no encontrado."
        n972 = Increment(x=w1350) -> (x+1=w1353:dbl)
        n973 = local write "Estatus (color)"(u32 8388608 ("Estatus (color)")) -> ()
        n974 = local write "Avance (número)"(w1350) -> ()
        n975 = local write "Avance (anillo)"(w1350) -> ()
        n976 = Bundle(cluster=cluster{dbl, i32} {0.0, 8388608}, w1350) -> (w1351:cluster{dbl, i32})  [unwired: 1 in]
        n977 = local write "Mensaje"("No se encontró variador.\nIntentar de nuevo.") -> ()
        n978 = Bundle(cluster=cluster{dbl, i32} {0.0, 9868950}, w1353) -> (w1352:cluster{dbl, i32})  [unwired: 1 in]
      }
      frame 3 {
        w1358 = 100.0
        # "Variador encontrado."
        n979 = Increment(x=w1358) -> (x+1=w1361:dbl)
        n980 = local write "Estatus (color)"(u32 6618880 ("Estatus (color)")) -> ()
        n981 = local write "Avance (número)"(w1358) -> ()
        n982 = local write "Avance (anillo)"(w1358) -> ()
        n983 = Bundle(cluster=cluster{dbl, i32} {0.0, 16759552}, w1358) -> (w1359:cluster{dbl, i32})  [unwired: 1 in]
        n984 = local write "Mensaje"("Se encontró variador.\nConfigurar.") -> ()
        n985 = Bundle(cluster=cluster{dbl, i32} {0.0, 9868950}, w1361) -> (w1360:cluster{dbl, i32})  [unwired: 1 in]
      }
      frame 12 {
        w1375 = 100.0
        # "Variador configurado."
        n986 = local read "Fabricante"() -> (w1373:u32)
        n987 = Increment(x=w1375) -> (x+1=w1378:dbl)
        n988 = local write "Estatus (color)"(u32 6618880 ("Estatus (color)")) -> ()
        n989 = local write "Avance (número)"(w1375) -> ()
        n990 = local write "Avance (anillo)"(w1375) -> ()
        n991 = Bundle(cluster=cluster{dbl, i32} {0.0, 16759552}, w1375) -> (w1376:cluster{dbl, i32})  [unwired: 1 in]
        n992 = Bundle(cluster=cluster{dbl, i32} {0.0, 9868950}, w1378) -> (w1377:cluster{dbl, i32})  [unwired: 1 in]
        n993 = case shown="4" w1373 {
          tunnel: [w1412 w1440] -> w1368
          tunnel: [w1411 w1439] -> w1367
          tunnel: [w1410 w1438] -> w1366
          tunnel: [w1409 w1437] -> w1365
          frame 0, Default {
            # "Allen Bradley."
            n994 = local read "Referencias PowerFlex"() -> (w1413:T2)
            n995 = local read "Coincidentes"() -> (w1414:bool[])
            n996 = local read "I/O PowerFlex"() -> (w1417:T3)
            n997 = local read "Coincidentes"() -> (w1421:bool[])
            n998 = local read "Motor PowerFlex"() -> (w1418:T4)
            n999 = local read "Coincidentes"() -> (w1423:bool[])
            n1000 = local read "Modbus PowerFlex"() -> (w1419:T5)
            n1001 = local read "Coincidentes"() -> (w1427:bool[])
            n1002 = Unbundle By Name(w1413) -> ("Descargar"=w1416:bool)
            n1003 = Index Array(array=w1414, index=0) -> (element=w1432:bool)
            n1004 = Unbundle By Name(w1417) -> ("Descargar"=w1422:bool)
            n1005 = Index Array(array=w1421, index=1) -> (element=w1431:bool)
            n1006 = Unbundle By Name(w1418) -> ("Descargar"=w1425:bool)
            n1007 = Index Array(array=w1423, index=2) -> (element=w1430:bool)
            n1008 = Unbundle By Name(w1419) -> ("Descargar"=w1428:bool)
            n1009 = Index Array(array=w1427, index=3) -> (element=w1429:bool)
            n1010 = Build Array(w1416, w1432) -> (w1433:bool[])
            n1011 = Build Array(w1422, w1431) -> (w1434:bool[])
            n1012 = Build Array(w1425, w1430) -> (w1435:bool[])
            n1013 = Build Array(w1428, w1429) -> (w1436:bool[])
            n1014 = Boolean Array To Number(Boolean array=w1433) -> (number=w1412:u32)
            n1015 = Boolean Array To Number(Boolean array=w1434) -> (number=w1411:u32)
            n1016 = Boolean Array To Number(Boolean array=w1435) -> (number=w1410:u32)
            n1017 = Boolean Array To Number(Boolean array=w1436) -> (number=w1409:u32)
          }
          frame 4 {
            # "LS-Electric."
            n1018 = local read "Referencias LS-Electric"() -> (w1441:T2)
            n1019 = local read "Coincidentes"() -> (w1442:bool[])
            n1020 = local read "I/O LS-Electric"() -> (w1445:T9)
            n1021 = local read "Coincidentes"() -> (w1449:bool[])
            n1022 = local read "Motor LS-Electric"() -> (w1446:T10)
            n1023 = local read "Coincidentes"() -> (w1451:bool[])
            n1024 = local read "Modbus LS-Electric"() -> (w1447:T11)
            n1025 = local read "Coincidentes"() -> (w1455:bool[])
            n1026 = Unbundle By Name(w1441) -> ("Descargar"=w1444:bool)
            n1027 = Index Array(array=w1442, index=0) -> (element=w1460:bool)
            n1028 = Unbundle By Name(w1445) -> ("Descargar"=w1450:bool)
            n1029 = Index Array(array=w1449, index=1) -> (element=w1459:bool)
            n1030 = Unbundle By Name(w1446) -> ("Descargar"=w1453:bool)
            n1031 = Index Array(array=w1451, index=2) -> (element=w1458:bool)
            n1032 = Unbundle By Name(w1447) -> ("Descargar"=w1456:bool)
            n1033 = Index Array(array=w1455, index=3) -> (element=w1457:bool)
            n1034 = Build Array(w1444, w1460) -> (w1461:bool[])
            n1035 = Build Array(w1450, w1459) -> (w1462:bool[])
            n1036 = Build Array(w1453, w1458) -> (w1463:bool[])
            n1037 = Build Array(w1456, w1457) -> (w1464:bool[])
            n1038 = Boolean Array To Number(Boolean array=w1461) -> (number=w1440:u32)
            n1039 = Boolean Array To Number(Boolean array=w1462) -> (number=w1439:u32)
            n1040 = Boolean Array To Number(Boolean array=w1463) -> (number=w1438:u32)
            n1041 = Boolean Array To Number(Boolean array=w1464) -> (number=w1437:u32)
          }
        }
        n1042 = case shown="1" w1368 {
          tunnel: ["" w1405 w1406] -> w1369
          frame 0, Default {
            # "Nada."
          }
          frame 1 {
            # "Error de configuración."
            n1043 = Concatenate Strings("-Hubo un error al intentar configurar referencias.", "\r") -> (w1405:string)
          }
          frame 3 {
            # "Configuración correcta."
            n1044 = Concatenate Strings("-Referencias configuradas correctamente.", "\r") -> (w1406:string)
          }
        }
        n1045 = case shown="1" w1367 {
          tunnel: ["" w1397 w1400] -> w1370
          frame 0, Default {
            # "Nada."
          }
          frame 1 {
            # "Error de configuración."
            n1046 = Concatenate Strings("-Hubo un error al intentar configurar I/O.", "\r") -> (w1397:string)
          }
          frame 3 {
            # "Configuración correcta."
            n1047 = Concatenate Strings("-I/O configuradas correctamente.", "\r") -> (w1400:string)
          }
        }
        n1048 = case shown="0, Default" w1366 {
          tunnel: ["" w1390 w1393] -> w1371
          frame 0, Default {
            # "Nada."
          }
          frame 1 {
            # "Error de configuración."
            n1049 = Concatenate Strings("-Hubo un error al intentar configurar las características del motor.", "\r") -> (w1390:string)
          }
          frame 3 {
            # "Configuración correcta."
            n1050 = Concatenate Strings("-Características del motor configuradas correctamente.", "\r") -> (w1393:string)
          }
        }
        n1051 = case shown="1" w1365 {
          tunnel: ["" w1384 w1387] -> w1372
          frame 0, Default {
            # "Nada."
          }
          frame 1 {
            # "Error de configuración."
            n1052 = Concatenate Strings("-Parámetros Modbus configurados correctamente.", "\r") -> (w1384:string)
          }
          frame 3 {
            # "Error de configuración."
            n1053 = Concatenate Strings("-Hubo un error al intentar configurar los parámetros Modbus.", "\r") -> (w1387:string)
          }
        }
        n1054 = Concatenate Strings(w1369, w1370, w1371, w1372) -> (w1364:string)
        n1055 = local write "Mensaje"(w1364) -> ()
      }
      frame 4..11 {
        # "Configurando variador (referencias)."
        n1056 = local write "Estatus (color)"(u32 6618880 ("Estatus (color)")) -> ()
        n1057 = local write "Mensaje"("Configurando.") -> ()
        n1058 = local read "Fabricante"() -> (w1471:u32)
        n1059 = case shown="0, Default" w1471 {
          tunnel: [w1479 w1490] -> w1470
          frame 0, Default {
            # "Allen Bradley."
            n1060 = local read "Referencias PowerFlex"() -> (w1480:T2)
            n1061 = local read "I/O PowerFlex"() -> (w1481:T3)
            n1062 = local read "Motor PowerFlex"() -> (w1482:T4)
            n1063 = local read "Modbus PowerFlex"() -> (w1483:T5)
            n1064 = Unbundle By Name(w1480) -> ("Descargar"=w1484:bool)
            n1065 = Unbundle By Name(w1481) -> ("Descargar"=w1485:bool)
            n1066 = Unbundle By Name(w1482) -> ("Descargar"=w1486:bool)
            n1067 = Unbundle By Name(w1483) -> ("Descargar"=w1487:bool)
            n1068 = Build Array(w1484, w1485, w1486, w1487) -> (w1488:bool[])
            n1069 = Boolean Array To Number(Boolean array=w1488) -> (number=w1489:u32)
            n1070 = To Double Precision Float(number=w1489) -> (double precision float=w1479:dbl)
          }
          frame 4 {
            # "LS-Electric."
            n1071 = local read "Referencias LS-Electric"() -> (w1491:T2)
            n1072 = local read "I/O LS-Electric"() -> (w1492:T9)
            n1073 = local read "Motor LS-Electric"() -> (w1493:T10)
            n1074 = local read "Modbus LS-Electric"() -> (w1494:T11)
            n1075 = Unbundle By Name(w1491) -> ("Descargar"=w1495:bool)
            n1076 = Unbundle By Name(w1492) -> ("Descargar"=w1496:bool)
            n1077 = Unbundle By Name(w1493) -> ("Descargar"=w1497:bool)
            n1078 = Unbundle By Name(w1494) -> ("Descargar"=w1498:bool)
            n1079 = Build Array(w1495, w1496, w1497, w1498) -> (w1499:bool[])
            n1080 = Boolean Array To Number(Boolean array=w1499) -> (number=w1500:u32)
            n1081 = To Double Precision Float(number=w1500) -> (double precision float=w1490:dbl)
          }
        }
        n1082 = local read "Iteración"() -> (w1469:u32)
        n1083 = formula code="y_1 = x_0 + 1;\ny_2 = log(y_1) / log (2);\ny_3 = 20*y_2;\ny_4 = x_1*100/y_3;"("x_0"=w1470, "x_1"=w1469) -> ("y_1"=w1467:dbl, "y_2"=w1466:dbl, "y_3"=w1465:dbl, "y_4"=w1468:dbl)
        n1084 = Increment(x=w1468) -> (x+1=w1476:dbl)
        n1085 = local write "Avance (número)"(w1468) -> ()
        n1086 = local write "Avance (anillo)"(w1468) -> ()
        n1087 = Bundle(cluster=cluster{dbl, i32} {0.0, 16759552}, w1468) -> (w1474:cluster{dbl, i32})  [unwired: 1 in]
        n1088 = Bundle(cluster=cluster{dbl, i32} {0.0, 9868950}, w1476) -> (w1475:cluster{dbl, i32})  [unwired: 1 in]
      }
    }
    n1089 = local read "Escanear"() -> (w1327:bool)
    n1090 = global write "Temporales.vi" "Escanear"(w1327) -> ()
    n1091 = Replace Array Subset(array=cluster{dbl, u32}[] [{0.0, 9868950}, {1.0, 16759552}, {100.0, 9868950}, {100.0, 9868950}] ("Scale.Marker Values[]"), new element=w1316, index=1) -> (w1325:cluster{dbl, u32}[])
    n1092 = Replace Array Subset(array=w1325, new element=w1320, index=2) -> (w1326:cluster{dbl, u32}[])
    n1093 = Unbundle(w1316) -> (w1319:i32)  [unwired: 1 out]
    n1094 = property on="Avance (número)" class="DigNum (strict)"("NumText.TextColor"=w1319) -> (error out=w1318:errorcluster)  [unwired: 2 in, 1 out]
    n1095 = property on="Avance (anillo)" class="Knob (strict)"("Scale.MarkerVals[]"=w1326) -> (error out=w1317:errorcluster)  [unwired: 2 in, 1 out]
    n1096 = local read "Fabricante"() -> (w1314:u32)
    n1097 = local write "Contenedor Fabricantes"(w1314) -> ()
    n1098 = local read "Salir"() -> (w1313:bool)
    "cccc" <- "Color Box"
    "Color Box 2" <- "cccc 2"
  }
  n1099 = flat-sequence {
    frame #0 {
      # "Controles."
    }
  }
  n1100 = flat-sequence {
    frame #0 {
      w1509 = 0.0
      w1504 = u32 0
      w1505 = FALSE ("Salir")
      # "Inicialización de variables."
      n1101 = local write "Download"(w1505) -> ()
      n1102 = local write "Escanear"(w1505) -> ()
      n1103 = local write "Reset"(w1505) -> ()
      n1104 = local write "Run"(w1505) -> ()
      n1105 = global write "Temporales.vi" "Salir"(w1505) -> ()
      n1106 = local write "Salir"(w1505) -> ()
      n1107 = local write "Stop"(w1505) -> ()
      n1108 = local write "Avance (anillo)"(w1509) -> ()
      n1109 = local write "Avance (número)"(w1509) -> ()
      n1110 = global write "Temporales.vi" "Avance"(w1509) -> ()
      n1111 = local write "Paso"(w1504) -> ()
      n1112 = local write "Modos"(w1504) -> ()
      n1113 = local write "Iteración"(w1504) -> ()
      n1114 = local write "Mensaje"("") -> ()
      n1115 = Initialize Array(FALSE, 4 ("dimension size")) -> (w1501:bool[])
      n1116 = local write "Coincidentes"(w1501) -> ()
      n1117 = local read "Fabricante"() -> (w1508:u32)
      n1118 = case shown="0, Default" w1508 {
        tunnel: [w1513 w1524 w1533 w1540 w1549] -> w1507
        tunnel: [w1511 w1521 w1530 w1539 w1547] -> w1506
        frame 0, Default {
          # "Allen Bradley."
          n1119 = Build Array(cluster{bool, string} {FALSE, "02"}, cluster{bool, string} {FALSE, "03"}, cluster{bool, string} {FALSE, "05"}, cluster{bool, string} {FALSE, "06"}) -> (w1513:cluster{bool, string}[])
          n1120 = Build Array(cluster{bool, string} {FALSE, "R1"}) -> (w1511:cluster{bool, string}[])
        }
        frame 1 {
          # "Schneider."
          n1121 = Build Array(cluster{bool, string} {FALSE, "DI1"}, cluster{bool, string} {FALSE, "DI2"}, cluster{bool, string} {FALSE, "DI3"}, cluster{bool, string} {FALSE, "DI4"}, cluster{bool, string} {FALSE, "DI5"}, cluster{bool, string} {FALSE, "DI6"}) -> (w1524:cluster{bool, string}[])
          n1122 = Build Array(cluster{bool, string} {FALSE, "R1"}, cluster{bool, string} {FALSE, "R2"}, cluster{bool, string} {FALSE, "DQ"}) -> (w1521:cluster{bool, string}[])
        }
        frame 2 {
          # "Delta."
          n1123 = Build Array(cluster{bool, string} {FALSE, "MI1"}, cluster{bool, string} {FALSE, "MI2"}, cluster{bool, string} {FALSE, "MI3"}, cluster{bool, string} {FALSE, "MI4"}, cluster{bool, string} {FALSE, "MI5"}, cluster{bool, string} {FALSE, "MI6"}) -> (w1533:cluster{bool, string}[])
          n1124 = Build Array(cluster{bool, string} {FALSE, "RA"}) -> (w1530:cluster{bool, string}[])
        }
        frame 3 {
          # "ABB."
          n1125 = Build Array(cluster{bool, string} {FALSE, "8"}, cluster{bool, string} {FALSE, "9"}, cluster{bool, string} {FALSE, "10"}, cluster{bool, string} {FALSE, "11"}) -> (w1540:cluster{bool, string}[])
          n1126 = Build Array(cluster{bool, string} {FALSE, "7"}) -> (w1539:cluster{bool, string}[])
        }
        frame 4 {
          # "LS Electric."
          n1127 = Build Array(cluster{bool, string} {FALSE, "P1"}, cluster{bool, string} {FALSE, "P2"}, cluster{bool, string} {FALSE, "P3"}, cluster{bool, string} {FALSE, "P4"}, cluster{bool, string} {FALSE, "P5"}) -> (w1549:cluster{bool, string}[])
          n1128 = Build Array(cluster{bool, string} {FALSE, "R1"}, cluster{bool, string} {FALSE, "R2"}) -> (w1547:cluster{bool, string}[])
        }
      }
      n1129 = local write "Entradas digitales"(w1507) -> ()
      n1130 = local write "Salidas digitales"(w1506) -> ()
    }
  }
  n1131 = flat-sequence {
    tunnel: [w1567] -> _
    tunnel: [w1562] -> _
    tunnel: [w1561] -> _
    tunnel: [w1559] -> _
    tunnel: [w1558] -> _
    tunnel: [w1557] -> _
    tunnel: [w1556] -> _
    tunnel: [w1555] -> _
    tunnel: [w1554] -> _
    frame #0 {
      w1560 = T34."Enabled" ("Disabled")
      # "Habilitar/deshabilitar controles e indicadores."
      n1132 = property on="Mensaje" class="Str"("DisabledEnum"=w1560) -> (error out=w1567:errorcluster)  [unwired: 2 in, 1 out]
      n1133 = property on="Recetas Allen Bradley" class="Arr (strict)"("DisabledEnum"=w1560) -> (error out=w1554:errorcluster)  [unwired: 2 in, 1 out]
      n1134 = property on="Recetas Schneider" class="Arr (strict)"("DisabledEnum"=w1560) -> (error out=w1555:errorcluster)  [unwired: 2 in, 1 out]
      n1135 = property on="Recetas Delta" class="Arr (strict)"("DisabledEnum"=w1560) -> (error out=w1556:errorcluster)  [unwired: 2 in, 1 out]
      n1136 = property on="Recetas ABB" class="Arr (strict)"("DisabledEnum"=w1560) -> (error out=w1557:errorcluster)  [unwired: 2 in, 1 out]
      n1137 = property on="Recetas LS Electric" class="Arr (strict)"("DisabledEnum"=w1560) -> (error out=w1558:errorcluster)  [unwired: 2 in, 1 out]
      n1138 = property on="Programa" class="Clust (strict)"() -> (error out=w1559:errorcluster, "Controls[]"=w1566:refnum<vi>[])  [unwired: 2 in, 1 out]
      n1139 = Index Array(array=w1566, index=2) -> (element=w1564:refnum<vi>)
      n1140 = property class="Ctl"(reference=w1564, "DisabledEnum"=T34."Enabled" ("Disabled")) -> (reference out=w1561:refnum<vi>, error out=w1562:errorcluster)  [unwired: 1 in]
    }
  }
  n1141 = flat-sequence {
    tunnel: w3 -> [_]
    tunnel: [w1571] -> w1
    frame #0 {
      # "Guardar datos en memoria."
      n1142 = flat-sequence {
        tunnel: [w1574] -> w1570
        tunnel: [w1573] -> w1569
        tunnel: [w1572] -> w1568
        tunnel: w1570 -> [_]
        tunnel: w1569 -> [_]
        tunnel: w1568 -> [w1581]
        tunnel: [w1585] -> w1571
        frame #0 {
          w1580 = refnum<vi> refnum  # Ring
          # "Leer elementos del selector del programa."
          n1143 = property on="Programa" class="Clust (strict)"() -> ("Controls[]"=w1578:refnum<vi>[])  [unwired: 2 in, 2 out]
          n1144 = Index Array(array=w1578, index=2) -> (element=w1579:refnum<vi>)
          n1145 = To More Specific Class(target class=w1580, reference=w1579) -> (specific class reference=w1576:refnum<vi>, error out=w1575:errorcluster)  [unwired: 1 in]
          n1146 = property class="Ring"(reference=w1576, error in=w1575) -> (reference out=w1574:refnum<vi>, error out=w1573:errorcluster, "StringsAndValues[]"=w1572:T27)
        }
        frame #1 {
          # "Variables locales a globales."
          n1147 = local read "Puerto COM"() -> (w1584:refnum<visa-resource-name>)
          n1148 = local read "Programa"() -> (w1582:T12)
          n1149 = local read "Recetas Allen Bradley"() -> (w1583:T14)
          n1150 = global write "Permanentes.vi" "Puerto COM"(w1584) -> ()
          n1151 = global write "Permanentes.vi" "Programa"(w1582) -> ()
          n1152 = global write "Permanentes.vi" "Recetas Allen Bradley"(w1583) -> ()
          n1153 = global write "Permanentes.vi" "Recetas_Selector"(w1581) -> ()
        }
        frame #2 {
          # "Variables globales a archivo de texto."
          n1154 = Current VI's Path() -> (path=w1587:path)
          n1155 = Strip Path(path=w1587) -> (stripped path=w1586:path)  [unwired: 1 out]
          n1156 = Build Path(base path=w1586, name or relative path="Configuración\\Ajustes.cfg") -> (appended path=w1592:path)
          n1157 = call <vilib>:"Check if File or Folder Exists.vi"("error in (no error)"=errorcluster {"status"=FALSE, "code"=0, "source"=""}, "path"=w1592) -> ("error out"=w1589:errorcluster, "file or folder exists?"=w1588:bool, "dup path"=w1590:path)  [unwired: 7 in]
          n1158 = case shown="True" w1588 {
            tunnel: w1590 -> [w1596 w1600]
            tunnel: w1589 -> [w1595 w1601]
            tunnel: [w1594 w1598] -> w1585
            frame False {
              # "Se crea el archivo de configuración."
              n1159 = Open/Create/Replace File(file path (use dialog)=w1596, error in=w1595, operation (0:open)=T26."create") -> (error out=w1594:errorcluster)  [unwired: 3 in, 2 out]
            }
            frame True {
              # "Se guardan los valores alojados en el archivo de   configuración."
              n1160 = call "Leer escribir VIs.vi"("Write? (Read)"=TRUE, "error in"=w1601, "VIs to save-Restore"="Permanentes.vi", "Program File Path"=w1600) -> ("error out"=w1598:errorcluster)  [unwired: 7 in]
            }
          }
        }
      }
    }
  }
  n1161 = flat-sequence {
    tunnel: w1 -> [_]
    frame #0 {
      # "Indicadores."
    }
  }
  n1162 = flat-sequence {
    tunnel: w1 -> [_]
    frame #0 {
      # "Salir de LabVIEW."
      n1163 = Quit LabVIEW(quit? (T)=TRUE) -> ()
    }
  }
